vi "Position_TOTAL_R21_april_18.vi"(5 "Distance Between \nCameras  (*unit)":sgl=2.5) -> (12 "dX, dY\nLeft Cam":cluster{"X":sgl[], "Y":sgl[]}={"X"=[-5.750775, -4.1849813, -3.081379, -2.0098581, 0.0], "Y"=[7.9585915, 7.9595685, 7.960258, 7.960927, 0.0]}, 13 "Position Valid":bool=TRUE, 14 "Left Camera Real Coordinates":cluster{"X":sgl, "Y":sgl}={"X"=7.9602513, "Y"=5.592073}, 16 "dX, dY\nRight Cam":cluster{"X":sgl[], "Y":sgl[]}={"X"=[-7.3032045, -5.737411, -4.6338086, -3.5622878, -1.5524296], "Y"=[7.2714148, 7.2723923, 7.2730813, 7.273751, -0.68717635]}, 18 "Robot Coordinates":cluster{"X":sgl, "Y":sgl}={"X"=7.616663, "Y"=6.3682876}, 19 "Orietnation\n(current)":sgl=-23.843685 format="%#_13g")   [LabVIEW 2015]
uses:
  <vilib>/Analysis/NI_AALPro.lvlib
  <vilib>/myRIO/Instrument Drivers/Onboard IO/DIO/DIO.lvlib
  <vilib>/Analysis/coordinate.llb/2D Cartesian Coordinate Rotation (Array).vi
  <vilib>/Instr/_visa.llb/VISA Configure Serial Port (Instr).vi
panel:
  out "Current Cam State - L":T1(ring)
  out "Valid Beacon Sets_":bool[](array[boolean])=[TRUE, TRUE, TRUE, TRUE, FALSE]
  in  "Distance Threshold\nRef Triangles (*unit)":sgl=30.0
  out "dA2 4":sgl=9.6935425 format="%#_13g"
  out "dA2 2":sgl=9.6935425 format="%#_13g"
  out "dA2 3":sgl=9.6935425 format="%#_13g"
  out "Current Cam State - R":T1(ring)
  out "Beacon Scales - Left":sgl[](array[numeric])=[76.306, 116.841255, 157.35043, 195.67218, 0.0]
  out "Beacon Scales - Right":sgl[](array[numeric])=[76.306, 116.841255, 157.35043, 195.67218, 0.0]
  in  "New Orientation \nThreshold":sgl=10.0
  in  "Moving Average\nWindow Length":u8=5
  out "Current Recovery State -L":enum16{"Generic Sweep", "Recovery Search"}(ring)=enum."Recovery Search"
  out "Current Move Delta - L 2":u16
  out "Next Recovery State - Left":enum16{"Generic Sweep", "Recovery Search"}(ring)=enum."Recovery Search"
  out "Next Recovery State - Right":enum16{"Generic Sweep", "Recovery Search"}(ring)=enum."Recovery Search"
  out "Current Recovery State - Right":enum16{"Generic Sweep", "Recovery Search"}(ring)=enum."Recovery Search"
  in  "Initial Recovery State  - Right":enum16{"Generic Sweep", "Recovery Search"}(ring)=enum."Recovery Search"
  in  "Initial Recovery State - L":enum16{"Generic Sweep", "Recovery Search"}(ring)=enum."Recovery Search"
  out "Next Tracking State - Right":enum16{"Track", "Reactive Predict", ""}(ring)
  out "Current Tracking State - Right 2":enum16{"Track", "Reactive Predict", ""}(ring)
  in  "Initial Tracking State - Right":enum16{"Track", "Reactive Predict", ""}(ring)
  out "Last Track Angle - R":sgl=98.61328
  out "Next Tracking State - Left":enum16{"Track", "Reactive Predict", ""}(ring)
  in  "Initial Tracking State - Left":enum16{"Track", "Reactive Predict", ""}(ring)
  out "Current Tracking State - Left":enum16{"Track", "Reactive Predict", ""}(ring)
  in  "Timeout to \nEnable Reactive Predict":u16=5
  out "Tracking Timeout\nCount - R":i32
  in  "Tracking Timeout\nThreshold":i32=10
  out "Tracking Timeout\nCount - L":i32
  in  "Search Direction - in - Right":bool=TRUE
  out "Next Main State - Right":T2(ring)=enum."Tracking"
  in  "Recovery Search\nDirection - R":bool
  out "Recovery Mode Count in Right":i32
  out "Frames Processed\nCount - in Right":i32
  out "Recovery Search\nmove Count - Right":u16
  out "Recovery Search\nAttempt Count - Right":u16
  in  "Mounting Offset - Right":sgl=45.0
  in  "Tracking Angle - Right":sgl=98.60307
  in  "Current Servo Position\n- Right":u16
  out "New Data  Flag\nRight Servo":bool
  in  "Track Angle Valid  - Right":bool=TRUE
  out "Current Main State - Right":T2(ring)=enum."Tracking"
  in  "Initial Main State- Right":T2(ring)
  in  "Recovery Search\nDirection - L 2":bool
  in  "Max Recovery Count\n(Recovery Search) 2":u16
  in  "Max Recovery\nSearch Attempts 2":u16
  in  "Image Lock - Right 2":bool
  out "Last Track Angle - L":sgl=87.24609
  in  "Recovery Search\nDirection - L":bool=TRUE
  out "Next Main State - Left":T2(ring)=enum."Tracking"
  out "Current Move Delta - L":u16
  in  "Max Recovery Count\n(Recovery Search)":u16=10
  in  "Max Recovery\nSearch Attempts":u16=3
  out "Recovery Search\nAttempt Count - in - L":u16
  out "Recovery Search\nmove Count - in - L":u16
  in  "Image Lock - Right":bool=TRUE
  out "Recovery Mode Count - in Left":u16
  in  "Middle Beacon\nCoordinates":cluster{"X":sgl, "Y":sgl}={"X"=0.0, "Y"=2.5}
  in  "Min Num Frames\nper Search":i32=2
  in  "Wait Tick Threshold":i32=10
  out "Frames Processed\nCount - in -L":i32
  in  "Maximum Move \nServo Threshold":i16=300
  in  "Minimum Delta \nServo Threshold":i16=3
  in  "Mounting Offset - Left":sgl=-45.0
  in  "Search Step Size":u16=50
  in  "Search Direction - in - L":bool
  in  "Current Servo Position\n- Left":u16
  in  "Tracking Angle - Left":sgl=87.25689
  out "New Data  Flag\nLeft Servo":bool
  in  "Track Angle Valid - Left":bool=TRUE
  in  "Image Lock - Left":bool=TRUE
  in  "Initial Main State - Left":T2(ring)
  out "Current Main State - Left":T2(ring)=enum."Tracking"
  in  "Position Calc\nTimer":u32=100 caption="Position Calc Timer"
  in  "Fetch Input\n(mSec)":u32=20 caption="Update Camera Input\n(mSec)"
  out "Right Data\nInput Flag\n- Internal":bool=TRUE
  in  "Position Calc\nReady":bool
  out "This Servo \nAngle - Right":sgl=98.90625
  in  "Beacon Angles -R":sgl[](array[numeric])=[111.28093, 105.355774, 98.60307, 92.04714, 103.90625]
  in  "Beacon Angles - L":sgl[](array[numeric])=[101.98467, 94.59042, 87.25689, 80.30646, 91.66016]
  in  "Valid Angles -R":bool[](array[boolean])=[TRUE, TRUE, TRUE, TRUE, FALSE]
  in  "Valid Angles - L":bool[](array[boolean])=[TRUE, TRUE, TRUE, TRUE, FALSE]
  out "Left Data\nInput Flag\n- Internal":bool
  in  "Check Shared Var Timer":u32=50 caption="Main Loop\n Timer (ms)"
  out "Left_Flag 2":bool
  out "Right_Flag 2":bool
  out "Beacons Found\n- Left (Bool Array) 2":bool[](array[boolean])=[TRUE, TRUE, TRUE, TRUE, FALSE]
  out "LEFT Beacon Coord - X px (IN) 2":sgl[](array[numeric])=[76.306, 116.841255, 157.35043, 195.67218, 0.0]
  out "LEFT Beacon Position - Y px (IN) 2":sgl[](array[numeric])=[154.30304, 148.59094, 148.39949, 146.94655, 0.0]
  out "This Servo \nAngle - Left":sgl=86.66016
  in  "Compliance Slope":u8=128
  out "deltaMoveServo\n- R":i16
  out "Move Respond - R":bool
  out "Move Respond - L":bool
  out "Last Position":cluster{"X":sgl, "Y":sgl}={"X"=7.6261, "Y"=6.350474}
  out "Last Orientation":sgl=-23.876373
  in  "Distance\nBetween Beacons \n- Tolerance":sgl=0.35 format="%#_13g"
  in  "Distance\nBetween Beacons":sgl=1.0 format="%#_13g"
  out "dT":dbl=143.499
  out "Position Valid\nHistory":bool[](array[boolean])=[TRUE, FALSE, FALSE, TRUE, TRUE, FALSE, TRUE, TRUE, TRUE, TRUE, TRUE, TRUE, FALSE, TRUE, FALSE]
  out "Orientation\nHistory":sgl[](array[numeric])=[-23.876373, 0.0, 0.0, -23.938759, -24.0458, 0.0, -23.14014, -22.504314, -22.596928, -22.90728, -23.237453, -23.75214, 0.0, -23.808718, 0.0]
  out "Robot Coordinates\nHistory":cluster{sgl, sgl}[](array[cluster])=[{7.6261, 6.350474}, {0.0, 0.0}, {0.0, 0.0}, {7.63815, 6.33973}, {7.6316156, 6.322055}, {0.0, 0.0}, {7.6863523, 6.2558875}, {7.688662, 6.2228284}, {7.6736236, 6.2455945}, {7.6880507, 6.2819676}, {7.6893277, 6.3140097}, {7.668109, 6.3330927}, {0.0, 0.0}, {7.6506357, 6.3142757}, {0.0, 0.0}]
  in  "New Position \nThreshold":sgl=2.5
  out "Orientation Avgd":sgl=-23.876373
  in  "History Size":u8=15
  in  "Max Y (arena)":sgl=15.0
  in  "Max X (arena)":sgl=35.0
  in  "New Position\nWeight":sgl=0.5 format="%#_13g"
  in  "Max Std Dev (3)":sgl=0.2 format="%#_13g"
  in  "Max Std Dev (4)":sgl=0.2 format="%#_13g"
  out "Post Filtering\n- Valid Beacons":bool[](array[boolean])=[FALSE, TRUE, TRUE, TRUE, FALSE]
  out "Robot Coordinates - Avgd":cluster{"X":sgl, "Y":sgl}={"X"=7.6261, "Y"=6.350474}
  out "Real Position in Course 2":cluster{"X":dbl[], "Y":dbl[]}(graph)={"X"=[7.626100046018056], "Y"=[6.35047366782369]}
  out "Position \nLock Status":bool=TRUE
  out "Right Camera Real Coordinate":cluster{"X":sgl, "Y":sgl}={"X"=7.2730746, "Y"=7.1445026}
  out "deltaMoveServo\n- L":i16
  in  "Search Step Size\n(deg)":sgl=15.0 format="%#_13g"
  out "Beacons Found\n- Right (Bool Array)":bool[](array[boolean])=[TRUE, TRUE, TRUE, TRUE, FALSE]
  out "RIGHT Beacon Position - Y px (IN)":sgl[](array[numeric])=[153.02994, 149.48933, 150.4864, 150.33003, 0.0]
  out "RIGHT Beacon Coord - X px (IN)":sgl[](array[numeric])=[91.3685, 123.99656, 161.27843, 197.4523, 0.0]
  in  "Right Servo\nID":string="\u0001"
  in  "Servo Comm\nWait Time - (ms)":i32
  in  "Left Servo\nID":string="\u0000"
  out "dT - Comm Loop":u32=19
  in  "Servo Comm\nLoop Time (ms)":i32=20
  in  "close comms":bool
  in  "Max Read\nTx Attempts":u8=3
  in  "Max Write\nTx Attempts":u8=3
  out "Current R (10bit)":u16=696
  out "Servo Moving - R":bool
  out "Servo Moving - L":bool
  out "Current L (10bit)":u16=347
  in  "SERVO ENABLE":bool=TRUE
  out "Move Servo - L":bool
  out "Move Servo - R":bool
  in  "Servo Goal Position\n - Right":u16=695
  in  "Move Servo\nThreshold (deg)":sgl=2.0 format="%#_13g"
  in  "Servo Algorithm\nCycle Time(ms)":i32=25
  in  "Servo Goal Position\n - Left":u16=349
  in  "Current Angle\n - Left (internal)":sgl=86.66016
  in  "Current Angle\n - Right (internal)":sgl=98.90625
  in  "stop":bool
  in  "Num of Beacons (Total)":i8=5
  out "Angle to Pixel Ratios":T3={"Angle to Pixel\nRatio - Horizontal"=0.18125, "Angle to Pixel\nRatio - Vertical"=0.1875} {"Angle to Pixel\nRatio - Vertical" format="%#_13g"; "Angle to Pixel\nRatio - Horizontal" format="%#_13g"}
  in  "Cam AOV Vertical (deg)":sgl=45.0
  in  "Cam AOV Horizontal (deg)":sgl=58.0
  in  "Image Height (px)":sgl=240.0
  in  "Image Width (px)":sgl=320.0
  out "Beacon Coordinates - Left Image":T4={"Beacon Position - X px"=[76.306, 116.841255, 157.35043, 195.67218, 0.0], "Beacon Position - Y px"=[154.30304, 148.59094, 148.39949, 146.94655, 0.0]}
  out "Beacon Coordinates - Right Image":T4={"Beacon Position - X px"=[91.3685, 123.99656, 161.27843, 197.4523, 0.0], "Beacon Position - Y px"=[153.02994, 149.48933, 150.4864, 150.33003, 0.0]}
  out "Distance to LBF":sgl[](array[numeric])=[0.024284193, 0.015691843, 0.008273765, 0.028971607, 0.03291407]
  out "Local Coordinates - Calculated":cluster{sgl[], sgl[]}(graph)={[-2.0384164, -0.70265853, 0.4090246, 1.3811935, 0.0], [9.602626, 8.751521, 8.536832, 8.085801, 0.0]}
  out "Local Coordinates - Rotated":cluster{dbl[], dbl[]}(graph)={[1.5524295802029098, -5.750774735805926, -4.1849814062260675, -3.0813788557258652, -2.009858210562305, 0.0], [0.6871763361707266, 7.9585912385832795, 7.959568450875426, 7.960257859242679, 7.960927027680405, 0.0]}
  out "All Object Coordinates \n- Local - Rotated":cluster{"X":sgl[], "Y":sgl[]}={"X"=[1.5524296, -5.750775, -4.1849813, -3.081379, -2.0098581, 0.0], "Y"=[0.68717635, 7.9585915, 7.9595685, 7.960258, 7.960927, 0.0]}
  out "Local Coordinates - Normalized":cluster{sgl[], dbl[]}(graph)={[1.6977187, -2.0372734, -0.60508364, 0.4043527, 1.3844445, 0.0], [0.0, 9.605212211608887, 8.972328186035156, 8.526259422302246, 8.093157768249512, 0.0]}
  in  "Max Std Dev (5)":sgl=0.2 format="%#_13g"
  out "All Object Coordinates \n- Local":cluster{"X":sgl[], "Y":sgl[]}={"X"=[1.6977187, -2.0372734, -0.60508364, 0.4043527, 1.3844445, 0.0], "Y"=[0.0, 9.605212, 8.972328, 8.526259, 8.093158, 0.0]}
  out "LOCAL\nBeacon Coordinates\nRelative to Robot":cluster{"dX_beacon":sgl[], "dY_beacon":sgl[]}={"dX_beacon"=[-2.0384164, -0.70265853, 0.4090246, 1.3811935, 0.0], "dY_beacon"=[9.602626, 8.751521, 8.536832, 8.085801, 0.0]}
  in  "Real Beacon\n - Coordinates":cluster{"X":dbl[], "Y":dbl[]}={"X"=[0.0, 0.0, 0.0, 0.0, 0.0, 0.0], "Y"=[0.5, 1.5, 2.5, 3.5, 4.5, 0.0]}
  # "POSITION CALCULATION VARIABLES"
  # "OUTPUT VALUES"
  # "CONFIG VALUES"
  # "FILTER CONFIG VALUES"
  # "FEEDBACK INPUT VALUES"
  # "INPUT VALUES"
  # "INTERMEDIATE VALUES"
  # "IMAGE TO ANGLE VARIABLES"
  # "VISION PROCESSEING INPUTS"
  # "Use moving average for previous orientation thresholds"
  # "INPUTS"
  # "CONFIG"
  # "OUTPUT VALUES"
  # "*********************"
  # "unfiltered"
  # "NEW FILTER VALS"
  # "Inter Beacon Distance Filtering"
  # "SERVO CONTROL VARIABLES"
  # "SERVO CONTROL VARIABLES"
  # "CONFIG"
  # "SHARED VARIABLE INPUTS"
  # "LOCAL VARIABLE INPUTS"
  # "INTERNRAL VARIABLES"
  # "SEARCH ROUTINE VARIABLES"
  # "MISC"
  # "SERVO IDs"
  # "CONTROL DELAYS"
  # "COMM LOOP DELAY"
  # "COMM PROTOCOL"
  # "SETTINGS"
  # "Make function of distance^^"
  # "**** only left side starts search\nat previously known good angle"
  # "LEFT SERVO"
  # "RIGHT SERVO"
  # "Main State Machine"
  # "Recovery State Machine"
  # "Current Track Angle Inputs"
  # "Servo Status Inputs"
  # "Main State Machine Inputs"
  # "Recovery State Machine Inputs"
  # "Current Track Angle Inputs"
  # "Servo Status Inputs"
  # "Recovery State Machine Feedback"
  # "Tracking State Machine Inputs"
  # "Tracking State Machine Inputs"
  # "NOTE: Must be 1 bigger than amount of beacons"
  # "NOTE: Must be 1 bigger than amount of beacons"
types:
  T1 = enum16{"Super Close Range", "Short Range", "Long Range"}
  T2 = enum16{"Start Up Search", "Tracking", "Recovery Mode", ""}
  T3 = cluster{"Angle to Pixel\nRatio - Horizontal":sgl, "Angle to Pixel\nRatio - Vertical":sgl}
  T4 = cluster{"Beacon Position - X px":sgl[], "Beacon Position - Y px":sgl[]}
  T5 = cluster{"Tracking Coordinates":cluster{"X":dbl, "Y":dbl}, "Current Valid":bool, "Current State - Out":enum16{"Sub - 2", "Sub - 3", "Sub - 4", "Normal - 5"}}
  T6 = enum16{"Sub - 2", "Sub - 3", "Sub - 4", "Normal - 5"}
  T7 = cluster{"Array of Double":dbl[], "Array of Double":dbl[]}
  T8 = typedef "DIO.lvlib/DIO Reference.ctl" = cluster{"myRIO Reference":T9, "DIO Channels List":T13}
  T9 = typedef "myRIO Generic Hardware Reference.ctl" = cluster{"myRIO Model":T10, "myRIO Hardware Reference":T11}
  T10 = typedef "Hardware Version Enum.ctl" = enum16{"Unknown", "myRIO-1900", "myRIO-1950", "roboRIO"}
  T11 = typedef "myRIO v1.0 Reference.ctl" = cluster{"Generic FPGA Reference":T12, "Allow multiple opens":bool}
  T12 = typedef "Generic FPGA Reference.ctl" = refnum<k20>
  T13 = typedef "DIO Channels List.ctl" = T14[]
  T14 = typedef "DIO Channels Enum.ctl" = enum16{"Not Connected", "C/DIO0", "C/DIO1", "C/DIO2", "C/DIO3", "C/DIO4", "C/DIO5", "C/DIO6", "C/DIO7", "A/DIO0", "A/DIO1", "A/DIO2", "A/DIO3", "A/DIO4", "A/DIO5", "A/DIO6", "A/DIO7", "A/DIO8", "A/DIO9", "A/DIO10", "A/DIO11", "A/DIO12", "A/DIO13", "A/DIO14", "A/DIO15", "B/DIO0", "B/DIO1", "B/DIO2", "B/DIO3", "B/DIO4", "B/DIO5", "B/DIO6", "B/DIO7", "B/DIO8", "B/DIO9", "B/DIO10", "B/DIO11", "B/DIO12", "B/DIO13", "B/DIO14", "B/DIO15", "LED0", "LED1", "LED2", "LED3", "Button0", "DIO/DIO0", "DIO/DIO1", "DIO/DIO2", "DIO/DIO3", "DIO/DIO4", "DIO/DIO5", "DIO/DIO6", "DIO/DIO7", "DIO/DIO8", "DIO/DIO9", "SPI/CS0", "SPI/CS1", "SPI/CS2", "SPI/CS3", "LED RADIO (Green)", "LED RADIO (Red)", "LED COMM (Green)", "LED COMM (Red)", "LED MODE (Green)", "LED MODE (Red)"}
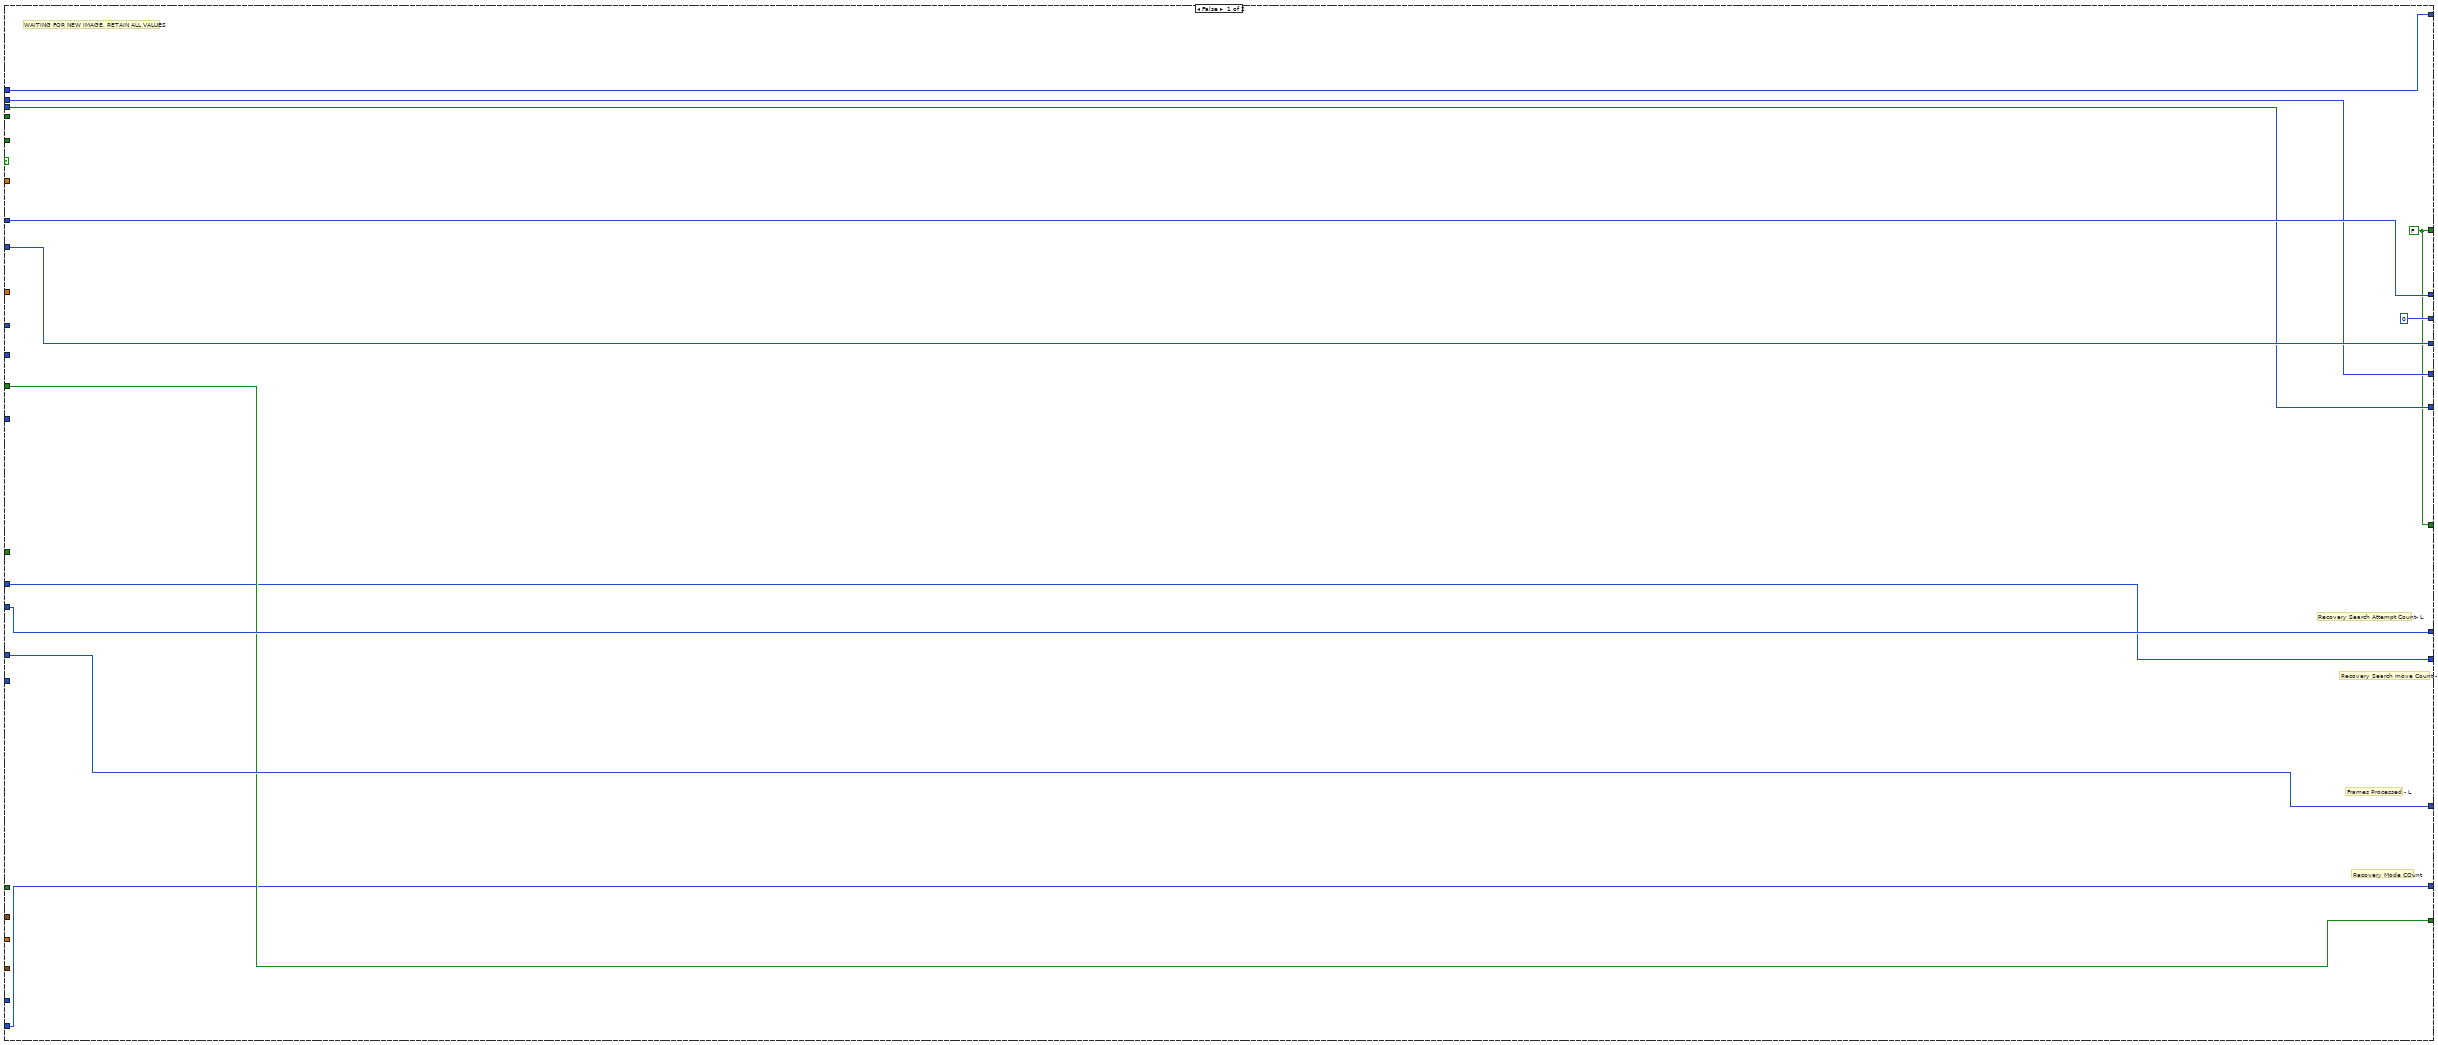
[diagram p2: hidden frame]
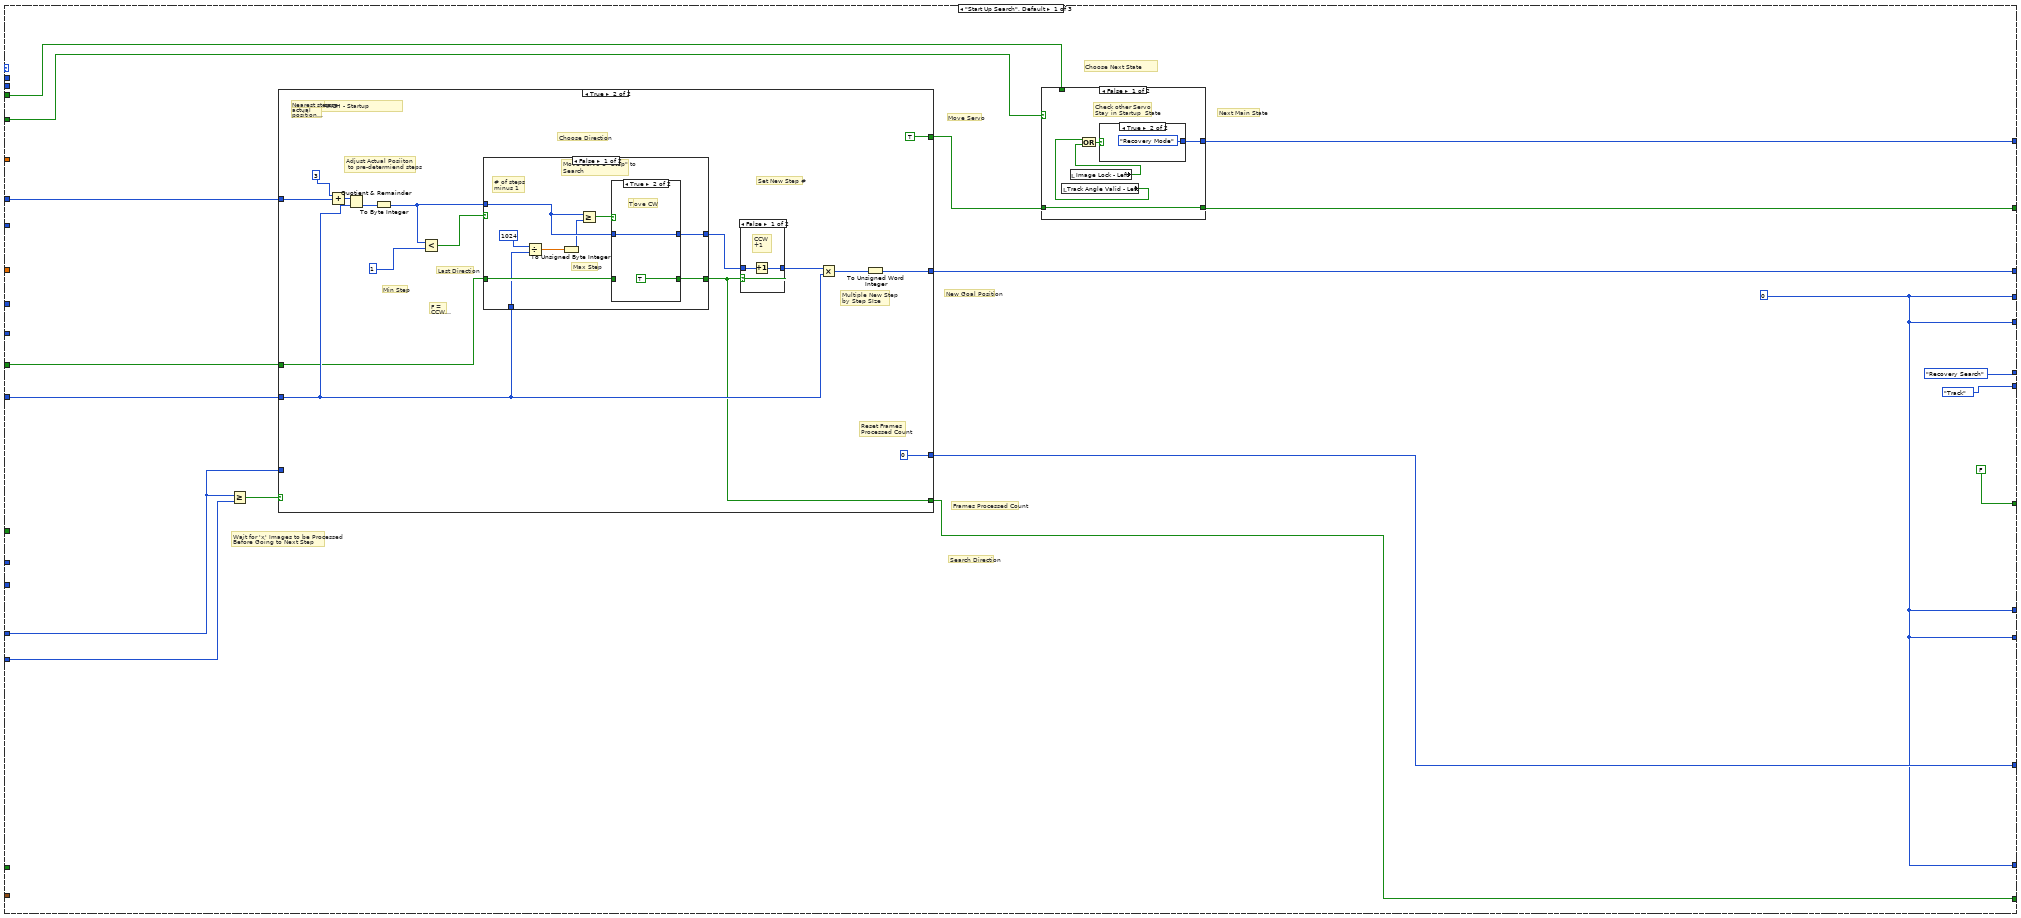
[diagram p3: hidden frame]
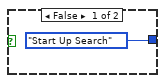
[diagram p4: hidden frame]
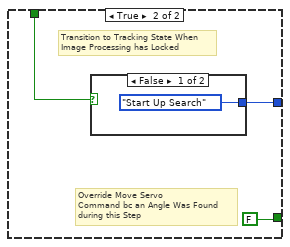
[diagram p5: hidden frame]
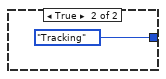
[diagram p6: hidden frame]
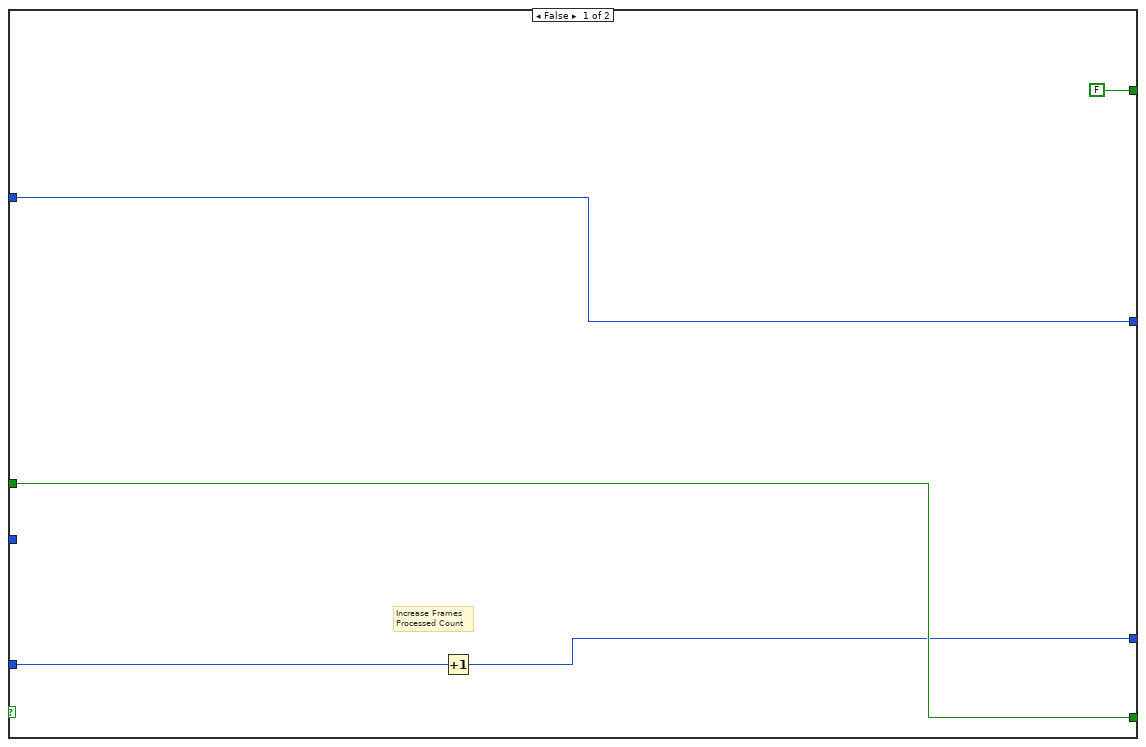
[diagram p7: hidden frame]
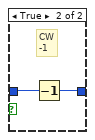
[diagram p8: hidden frame]
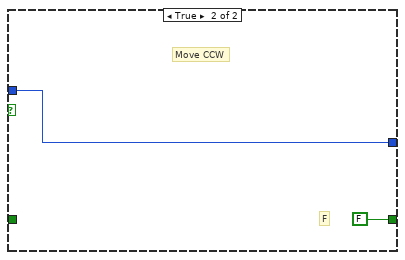
[diagram p10: hidden frame]
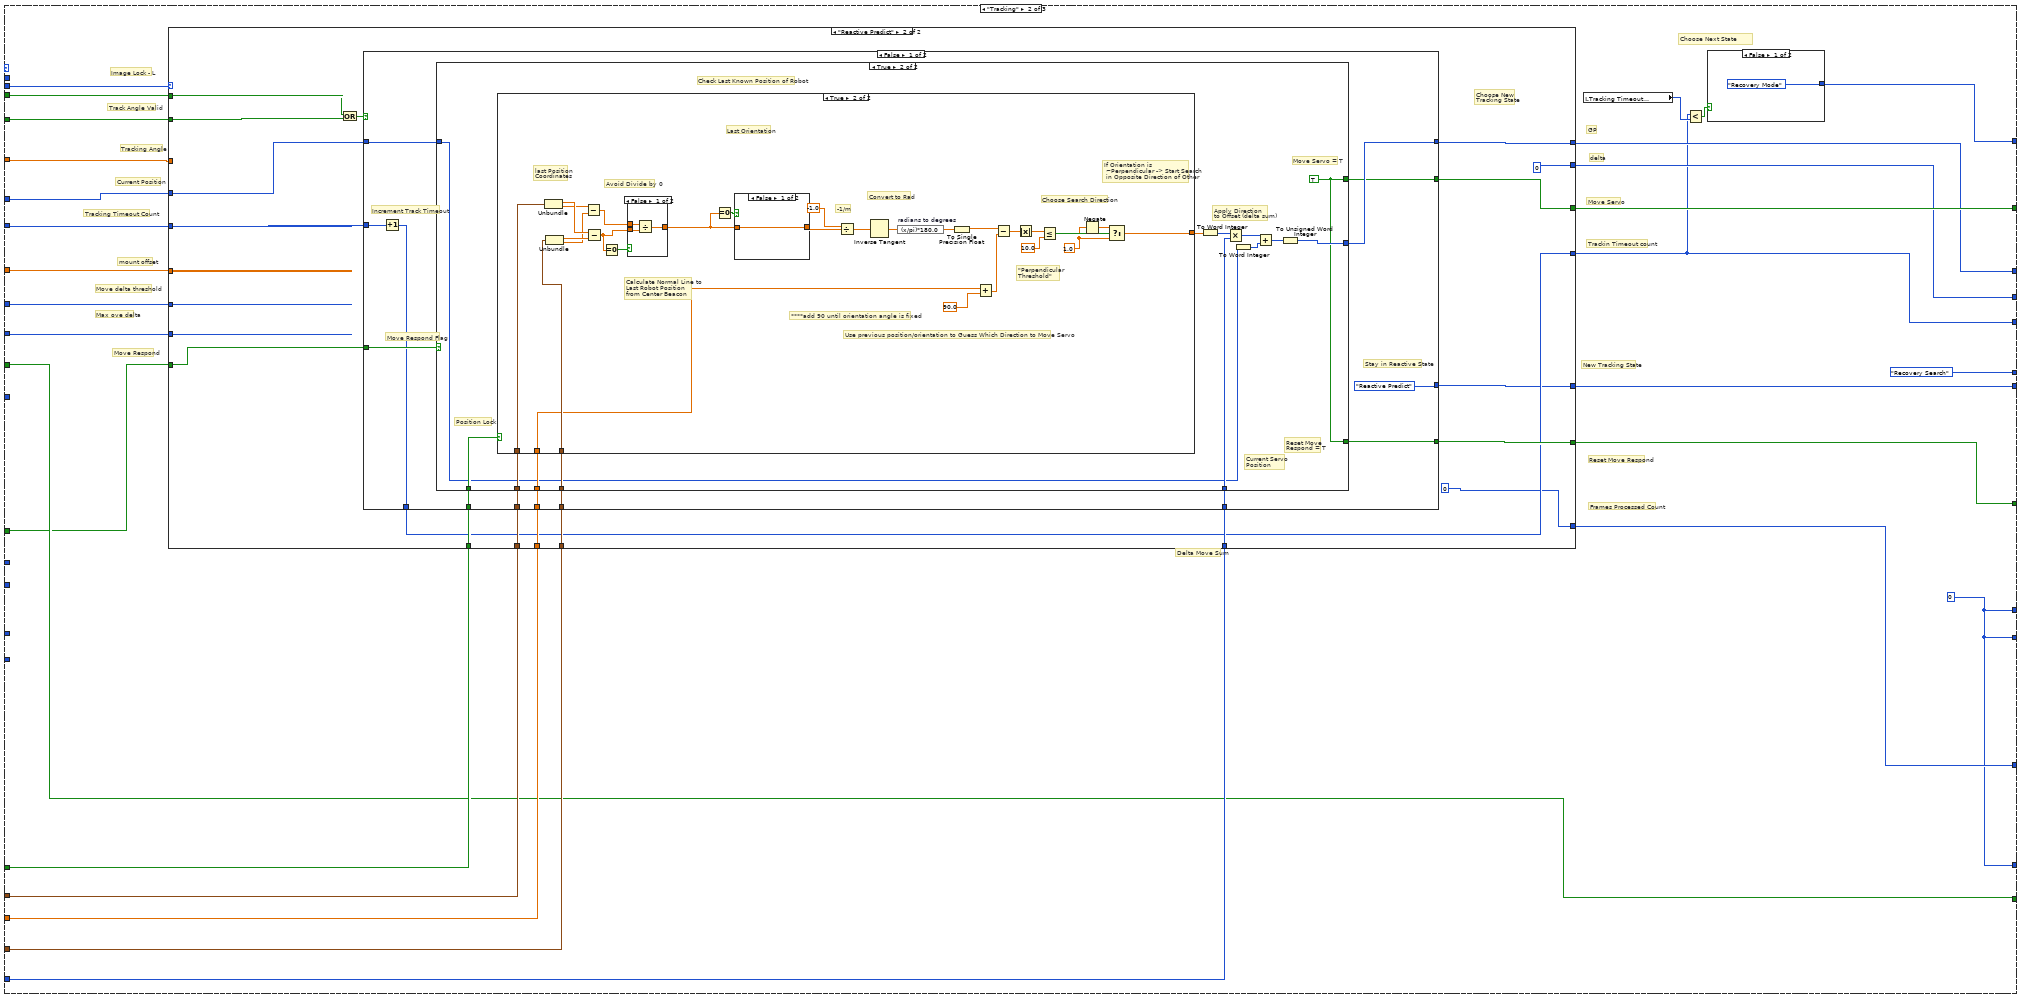
[diagram p11: hidden frame]
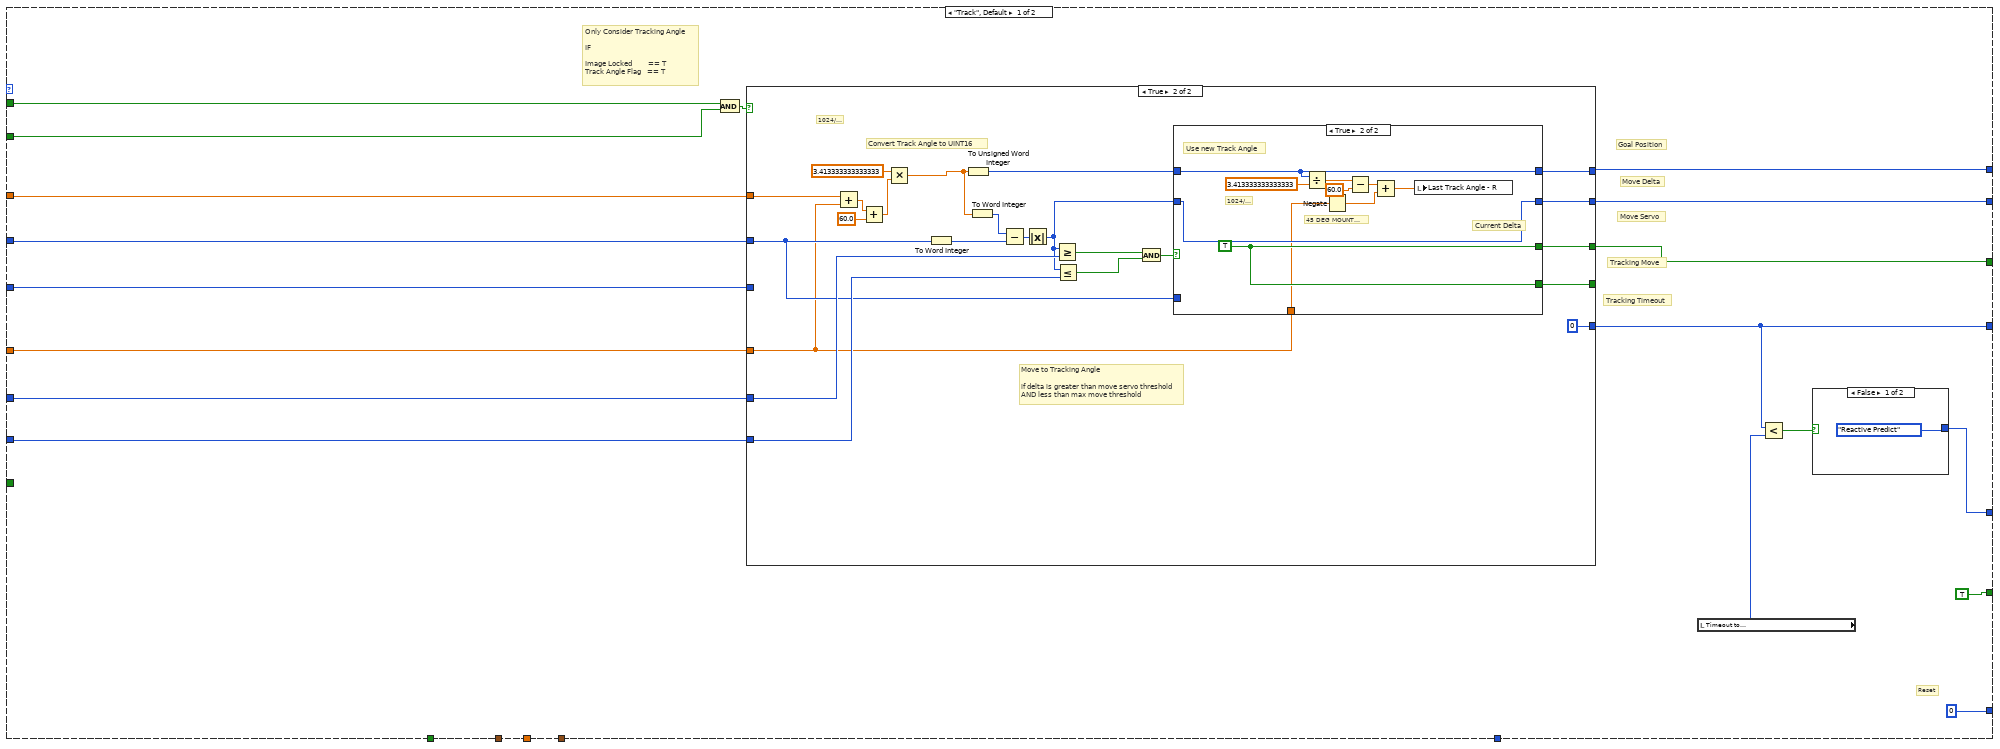
[diagram p12: hidden frame]
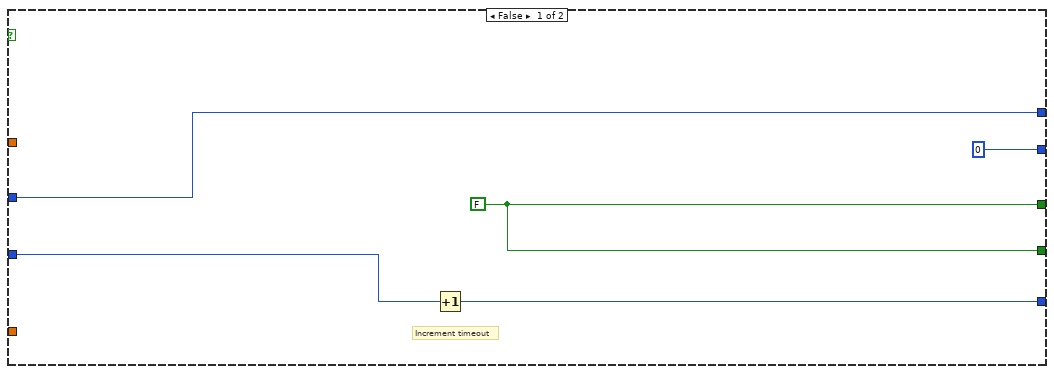
[diagram p13: hidden frame]
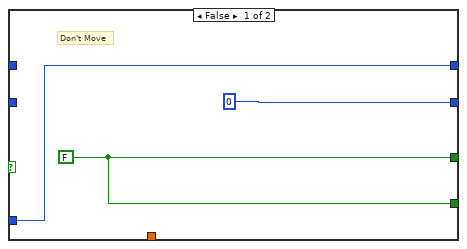
[diagram p14: hidden frame]
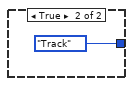
[diagram p15: hidden frame]
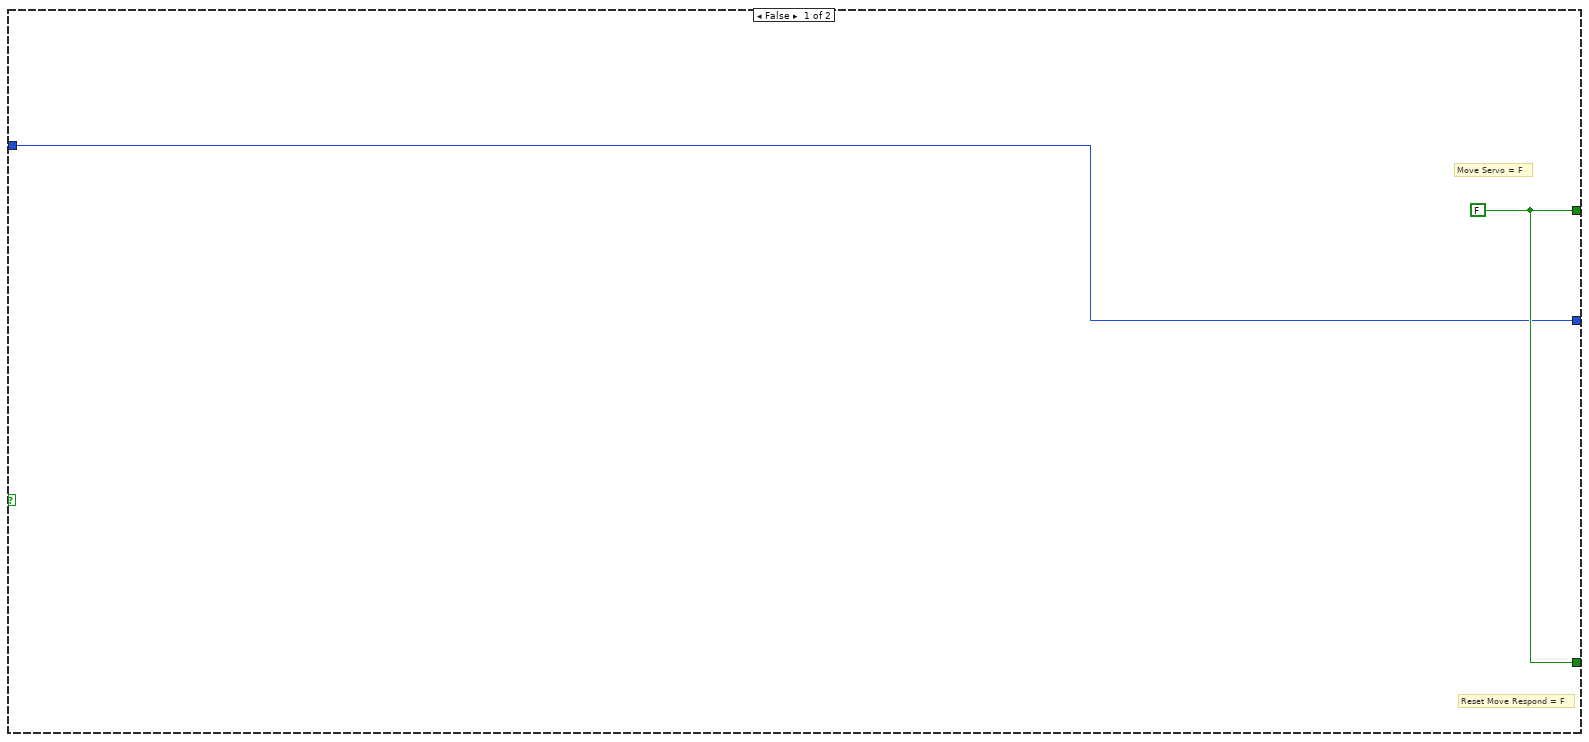
[diagram p16: hidden frame]
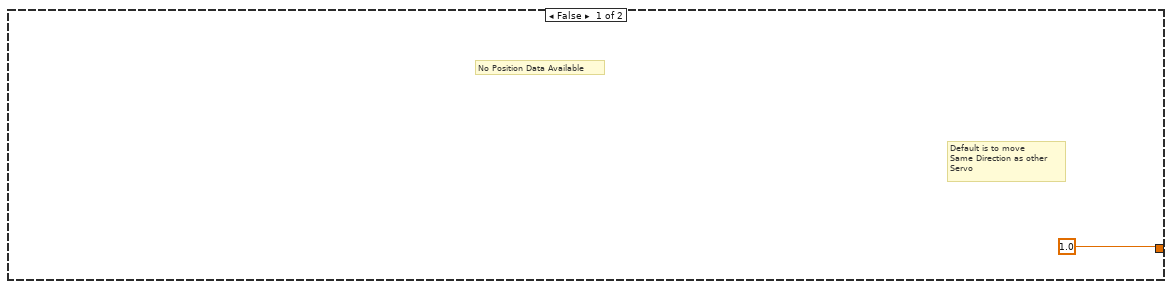
[diagram p17: hidden frame]
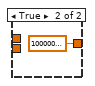
[diagram p18: hidden frame]
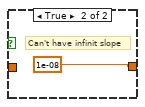
[diagram p19: hidden frame]
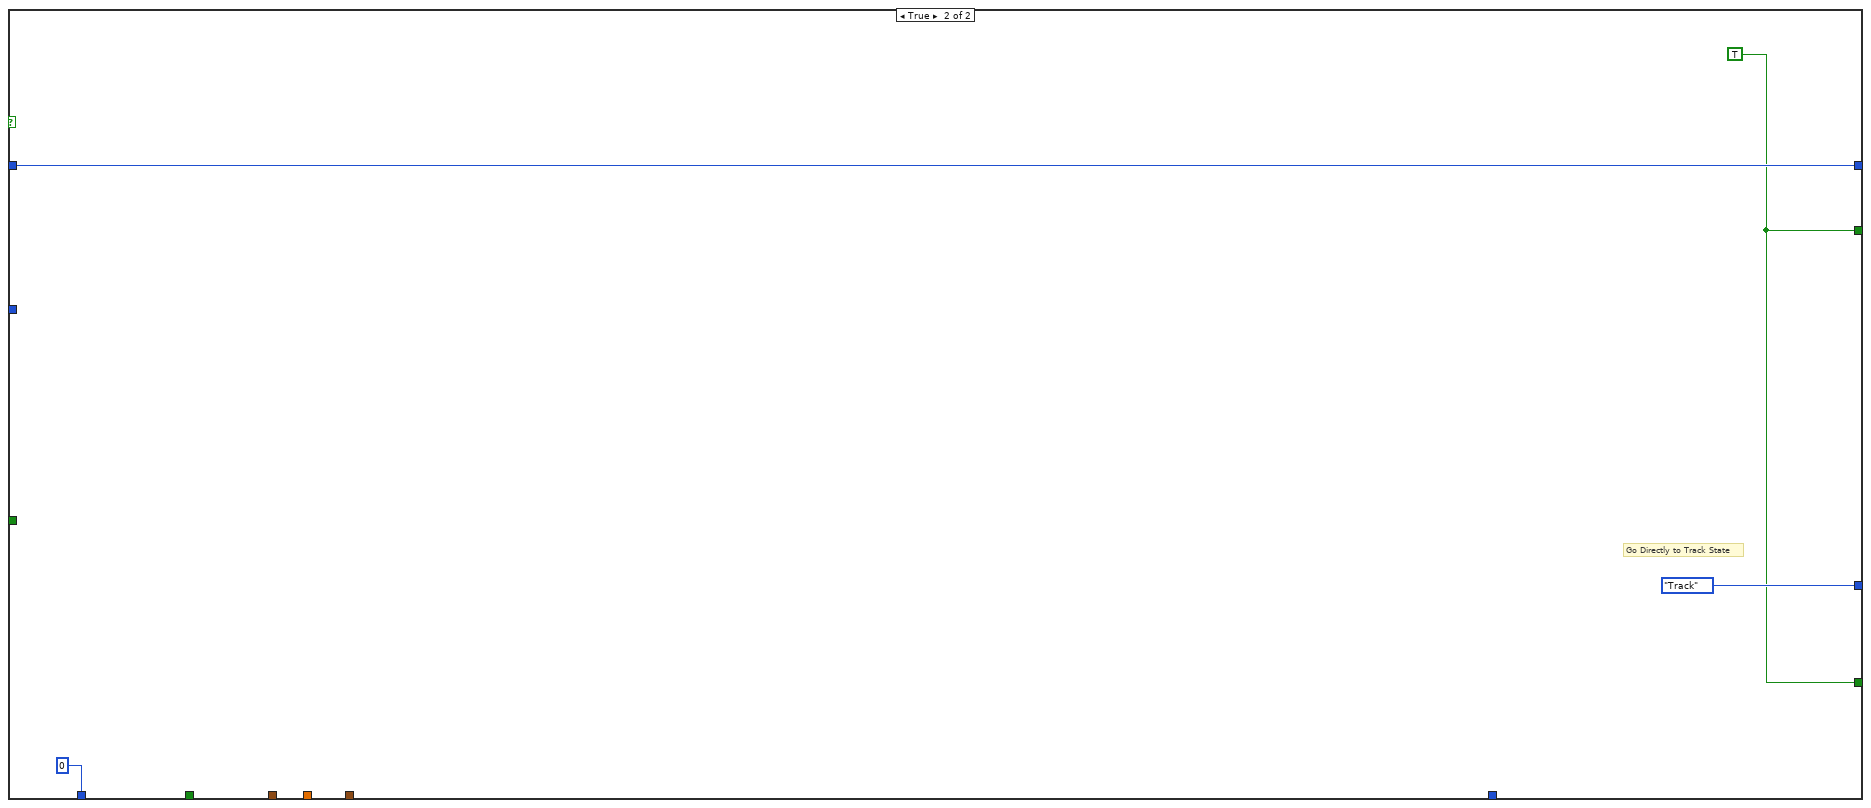
[diagram p20: hidden frame]
diagram:
  (unwired) enum16{"Generic Sweep", "Recovery Search"}."Recovery Search"
  w12 = 0 ("Frames Processed\nCount - in")
  w13 = 0 ("Frames Processed\nCount - in")
  w2 = FALSE
  w34 = sgl 0.0
  # "SERVO CONTROL FLAGS"
  # "***"
  # "Next Tracking State"
  # "Tracking Timeout Count"
  # "Search Direction - L"
  # "Next Recovery State"
  # "Move Respond"
  # "Recovery Mode Count - L"
  # "Delta Move Sum - L"
  # "Wait Tick Count - L"
  # "Frames Processed - L"
  # "Recovery Search move Count - L"
  # "Recovery Search Attempt Count- L"
  # "Next Main State"
  # "Search Direction - L"
  # "Next Recovery State"
  # "INPUTS - Local vars"
  # "Recovery Mode Count - L"
  # "Delta Move Sum - L"
  # "Frames Processed\nLeft"
  # "Move Respond - R"
  # "Initial Search Direction\n- Right"
  # "Move Respond"
  # "Recovery Mode Count - L"
  # "Delta Move Sum - L"
  # "Wait Tick Count - L"
  # "Frames Processed - L"
  # "Recovery Search move Count - L"
  # "Recovery Search Attempt Count- L"
  # "Next Main State"
  # "Settings -- Update in a slow loop"
  # "Recovery Mode Count - L"
  # "Delta Move Sum - L"
  # "Frames Processed\nLeft"
  # "Move Respond - L"
  # "Replace these with\nconstants"
  # "Initial Search Direction\n- Left"
  # "Read Inputs when Available"
  # "# of Physical Beacons"
  # "Right Data Internal Falg"
  # "Left Data Internal Falg"
  # "Initialize Shift Arrays"
  # "Robot Position (cluster)\nShift Array"
  # "Robot Position (cluster)\nShift Array"
  # "Position Valid Shift Array"
  # "Orientation Shift Array"
  # "Position Valid Shift Array"
  # "Orientation Shift Array"
  # "Servo Communication (to Servo- UART))"
  # "Internal Local Variables"
  # "Servo Control Logic"
  # "Local Variables"
  # "Images to Robot Position Calculation Process"
  # "SERVO MOTOR CONTROL"
  # "SERVO MOTOR CONTROL"
  n1 = Divide(x="Cam AOV Horizontal (deg)", y="Image Width (px)") -> (x/y=w25:sgl)
  n2 = Divide(x="Cam AOV Vertical (deg)", y="Image Height (px)") -> (x/y=w26:sgl)
  n3 = Bundle(w25, w26) -> (w20:cluster{sgl, sgl})  [unwired: 1 in]
  "Angle to Pixel Ratios" <- w20
  n4 = disable-structure shown="Disabled" {
    frame Disabled {
      # "Always Read Incoming Flags & Store"
      n5 = while {
        tunnel: "Check Shared Var Timer" -> [w46]
        stop <- FALSE stop-if-true
        n6 = shared-variable "myRIO-1900\\Lib1.lvlib\\RIGHT_FLAG"() -> (→"Right_Flag 2":bool)  [unwired: 1 in, 1 out]
        n7 = shared-variable "myRIO-1900\\Lib1.lvlib\\Left_Flag"() -> (→"Left_Flag 2":bool)  [unwired: 1 in, 1 out]
        n8 = call "Wait8"("Count(mSec)"=w46) -> ()  [unwired: 1 out]
      }
    }
    frame Enabled {
    }
  }
  n9 = while {
    shift-right: [w55] -> _
    shift-left: w2 -> [w60]
    shift-right: [w54] -> _
    shift-left: w2 -> [w58]
    tunnel: w20 -> [w56]
    tunnel: "Num of Beacons (Total)" -> [w57]
    stop <- FALSE stop-if-true
    # "Wait for Both Internal Flags"
    n10 = call "Wait6"("Count(mSec)"="Fetch Input\n(mSec)") -> ()  [unwired: 1 out]
    n11 = shared-variable "RT myRIO Target - Overlord\\Localization_Variables_r0.lvlib\\RIGHT_FLAG"() -> (w51:bool)  [unwired: 1 in, 1 out]
    n12 = shared-variable "RT myRIO Target - Overlord\\Localization_Variables_r0.lvlib\\Left_Flag"() -> (w52:bool)  [unwired: 1 in, 1 out]
    n13 = case shown="True" w51 {
      tunnel: w57 -> [_ w79]
      tunnel: w56 -> [_ w77]
      tunnel: [w61 w67] -> w49
      tunnel: w58 -> [w61 _]
      frame False {
        # "Don't Update Servo Position\nbc we're waiting on new Data to\ncome in and the servo position\nwas set at the previous set of data"
      }
      frame True {
        w67 = TRUE
        # "Store Values"
        # "Raise Internal Flag"
        # "If New Data Available"
        # "From Shift Reg"
        # "Perforrm Indivudual Angle Calculation"
        # "Pull Down Individual Flag"
        n14 = shared-variable "RT myRIO Target - Overlord\\Localization_Variables_r0.lvlib\\RIGHT_BEACON_X_array"() -> (w73:dbl[])  [unwired: 1 in, 1 out]
        "RIGHT Beacon Coord - X px (IN)" <- w73
        n15 = shared-variable "RT myRIO Target - Overlord\\Localization_Variables_r0.lvlib\\Image Lock - R"() -> (w68:bool)  [unwired: 1 in, 1 out]
        n16 = shared-variable "RT myRIO Target - Overlord\\Localization_Variables_r0.lvlib\\RIGHT_BEACON_Scales"() -> (→"Beacon Scales - Right":sgl[])  [unwired: 1 in, 1 out]
        n17 = shared-variable "RT myRIO Target - Overlord\\Localization_Variables_r0.lvlib\\Info - Right"() -> (w65:T5)  [unwired: 1 in, 1 out]
        n18 = shared-variable "RT myRIO Target - Overlord\\Localization_Variables_r0.lvlib\\RIGHT_BEACON_Y_array"() -> (w72:dbl[])  [unwired: 1 in, 1 out]
        "RIGHT Beacon Position - Y px (IN)" <- w72
        n19 = shared-variable "RT myRIO Target - Overlord\\Localization_Variables_r0.lvlib\\RIGHT_BEACON_BOOL_array"() -> (w71:bool[])  [unwired: 1 in, 1 out]
        "Beacons Found\n- Right (Bool Array)" <- w71
        n20 = Unbundle By Name(w65) -> ("Tracking Coordinates"=w64:cluster{"X":dbl, "Y":dbl}, "Current Valid"=w63:bool, "Current State - Out"=→"Current Cam State - R":T6)
        n21 = local write "Image Lock - Right"(w68) -> ()
        n22 = Bundle("Array of Double"=w73, "Array of Double"=w72) -> (w70:T7)  [unwired: 1 in]
        "Beacon Coordinates - Right Image" <- w70
        n23 = shared-variable "RT myRIO Target - Overlord\\Localization_Variables_r0.lvlib\\Right Servo Angle_Image"() -> (w69:dbl)  [unwired: 1 in, 1 out]
        "This Servo \nAngle - Right" <- w69
        n24 = shared-variable "RT myRIO Target - Overlord\\Localization_Variables_r0.lvlib\\RIGHT_FLAG"(FALSE) -> ()  [unwired: 1 in, 1 out]
        n25 = feedback #1() -> (w81:sgl[])  [unwired: 1 in]
        n26 = feedback #2() -> (w80:bool[])  [unwired: 1 in]
        n27 = call "Angle Calc_Individual Process R4.vi"("Angle to Pixel Ratios"=w77, "Previous Angles"=w81, "Num of Beacons"=w79, "Beacon Coordinates - Image"=w70, "Current Servo Angle"=w69, "Beacons Found (Bool Array)"=w71, "Previous Valid Angles"=w80, "Tracking Coordinates"=w64) -> ("Servo Goal Angle"=w76:sgl, "Valid Beacons (Bool Array)\nPosition Calc"=w75:bool[], "Angle Of Beacons \nRelative to Robot"=w74:sgl[])  [unwired: 4 in, 1 out]
        n28 = feedback-in #1(w74) -> ()
        n29 = feedback-in #2(w75) -> ()
        n30 = local write "Beacon Angles -R"(w74) -> ()
        n31 = local write "Tracking Angle - Right"(w76) -> ()
        n32 = local write "Valid Angles -R"(w75) -> ()
        n33 = local write "Track Angle Valid  - Right"(w63) -> ()
        n34 = local write "New Data  Flag\nRight Servo"(w67) -> ()
      }
    }
    "Right Data\nInput Flag\n- Internal" <- w49
    n35 = case shown="True" w52 {
      tunnel: [w82 w88] -> w48
      tunnel: w60 -> [w82 _]
      tunnel: w56 -> [_ w92]
      tunnel: w57 -> [_ w91]
      frame False {
        # "Don't Update Servo Position\nbc we're waiting on new Data to\ncome in and the servo position\nwas set at the previous set of data"
      }
      frame True {
        w88 = TRUE
        # "Store Values"
        # "Raise Internal Flag"
        # "If New Data Available"
        # "Perforrm Indivudual Angle Calculation"
        # "Pull Down Individual Flag"
        n36 = shared-variable ".\\Localization_Variables_r0.lvlib\\LEFT_BEACON_X_array"() -> (w98:dbl[])  [unwired: 1 in, 1 out]
        "LEFT Beacon Coord - X px (IN) 2" <- w98
        n37 = shared-variable "RT myRIO Target - Overlord\\Localization_Variables_r0.lvlib\\LEFT_BEACON_Scales"() -> (→"Beacon Scales - Left":sgl[])  [unwired: 1 in, 1 out]
        n38 = shared-variable "RT myRIO Target - Overlord\\Localization_Variables_r0.lvlib\\LEFT_BEACON_Y_array"() -> (w99:dbl[])  [unwired: 1 in, 1 out]
        "LEFT Beacon Position - Y px (IN) 2" <- w99
        n39 = shared-variable "RT myRIO Target - Overlord\\Localization_Variables_r0.lvlib\\LEFT_BEACON_BOOL_array"() -> (w100:bool[])  [unwired: 1 in, 1 out]
        "Beacons Found\n- Left (Bool Array) 2" <- w100
        n40 = shared-variable "RT myRIO Target - Overlord\\Localization_Variables_r0.lvlib\\Image Lock - L"() -> (w89:bool)  [unwired: 1 in, 1 out]
        n41 = shared-variable "RT myRIO Target - Overlord\\Localization_Variables_r0.lvlib\\Info - Left"() -> (w85:T5)  [unwired: 1 in, 1 out]
        n42 = Unbundle By Name(w85) -> ("Tracking Coordinates"=w84:cluster{"X":dbl, "Y":dbl}, "Current Valid"=w83:bool, "Current State - Out"=→"Current Cam State - L":T6)
        n43 = local write "Image Lock - Left"(w89) -> ()
        n44 = Bundle("Array of Double"=w98, "Array of Double"=w99) -> (w96:T7)  [unwired: 1 in]
        "Beacon Coordinates - Left Image" <- w96
        n45 = shared-variable "RT myRIO Target - Overlord\\Localization_Variables_r0.lvlib\\Left Servo Angle_Image"() -> (w90:dbl)  [unwired: 1 in, 1 out]
        "This Servo \nAngle - Left" <- w90
        n46 = shared-variable "RT myRIO Target - Overlord\\Localization_Variables_r0.lvlib\\Left_Flag"(FALSE) -> ()  [unwired: 1 in, 1 out]
        n47 = feedback #3() -> (w102:sgl[])  [unwired: 1 in]
        n48 = feedback #4() -> (w101:bool[])  [unwired: 1 in]
        n49 = call "Angle Calc_Individual Process R4.vi"("Angle to Pixel Ratios"=w92, "Previous Angles"=w102, "Num of Beacons"=w91, "Beacon Coordinates - Image"=w96, "Current Servo Angle"=w90, "Beacons Found (Bool Array)"=w100, "Previous Valid Angles"=w101, "Tracking Coordinates"=w84) -> ("Servo Goal Angle"=w95:sgl, "Valid Beacons (Bool Array)\nPosition Calc"=w94:bool[], "Angle Of Beacons \nRelative to Robot"=w93:sgl[])  [unwired: 4 in, 1 out]
        n50 = feedback-in #3(w93) -> ()
        n51 = feedback-in #4(w94) -> ()
        n52 = local write "Beacon Angles - L"(w93) -> ()
        n53 = local write "Valid Angles - L"(w94) -> ()
        n54 = local write "Tracking Angle - Left"(w95) -> ()
        n55 = local write "Track Angle Valid - Left"(w83) -> ()
        n56 = local write "New Data  Flag\nLeft Servo"(w88) -> ()
      }
    }
    "Left Data\nInput Flag\n- Internal" <- w48
    n57 = And(x=w48, y=w49) -> (x .and. y?=w59:bool)
    n58 = case shown="True" w59 {
      selector: w59 -> [_ w105]
      tunnel: w48 -> [w104 _]
      tunnel: [w104 w106] -> w55
      tunnel: [w103 w106] -> w54
      tunnel: w49 -> [w103 _]
      frame False {
      }
      frame True {
        w106 = FALSE
        # "Reset Internal Data Flags"
        # "Position Data\nReady Enabled"
        n59 = local write "Position Calc\nReady"(w105) -> ()
      }
    }
  }
  n60 = Bundle(w34, w34) -> (w37:cluster{sgl, sgl})  [unwired: 1 in]
  n61 = Initialize Array(w34, "History Size") -> (w32:sgl[])
  n62 = Initialize Array(w37, "History Size") -> (w33:cluster{sgl, sgl}[])
  n63 = Initialize Array(FALSE, "History Size") -> (w31:bool[])
  n64 = call "Tick Count4"() -> ("Tick Count(uSec)"=w30:u32)
  n65 = while {
    shift-right: [w117] -> _
    shift-left: w32 -> [w114]
    shift-right: [w116] -> _
    shift-left: w31 -> [w115]
    shift-right: [w118] -> _
    shift-left: w33 -> [w109]
    shift-right: [w110] -> _
    shift-left: w30 -> [w111]
    stop <- "stop" stop-if-true
    n66 = call "Wait5"("Count(mSec)"="Position Calc\nTimer") -> ()  [unwired: 1 out]
    n67 = case shown="True" "Position Calc\nReady" {
      selector: "Position Calc\nReady" -> [_ w161]
      tunnel: w109 -> [_ w184]
      tunnel: w109 -> [w127 w178]
      tunnel: w114 -> [w129 w177]
      tunnel: w115 -> [w128 w176]
      tunnel: [w129 w183] -> w117
      tunnel: [w128 w181] -> w116
      tunnel: [w127 w182] -> w118
      tunnel: w115 -> [_ w175]
      tunnel: w114 -> [_ w174]
      tunnel: [w126 w168] -> w112
      tunnel: w111 -> [_ w168]
      tunnel: [FALSE TRUE] -> w113
      tunnel: w109 -> [_ w163]
      frame False {
        n68 = call "Tick Count5"() -> ("Tick Count(uSec)"=w126:u32)
      }
      frame True {
        w139 = T1."Long Range" ("Current Cam State - R")
        # "At least 2+ Avaialbe"
        # "***********do for both"
        # "sTATE"
        # "CALCULATE AVERAGE ORIENTATION"
        # "Update Outputs\nif Current Calc is Invalid\n(shouldn't matter)"
        # "Estimate Orienation Based on Previous Position"
        # "****# of previous in history that must be true\nin order for position to be considered \"locked\""
        # "New Position is Valid if both \nOrientation and Positions\nis within range of previous"
        # "Robot Position\n Shift Array"
        # "Position Valid Shift Array"
        # "Orientation Shift Array"
        # "Orientation Value"
        # "Shift & Insert Current Position Valid"
        # "Position Valid\n(orientation)"
        # "Position Valid\n(position)"
        # "Update Shift Registers"
        # "Shift & Insert Current Calculated Orientation"
        # "Shift & Insert Current Robot Position"
        # "UPDATE FINAL OUTPUT\n VALUES"
        n69 = Not(x=w161) -> (.not. x?=w162:bool)
        n70 = local read "Num of Beacons (Total)"() -> (w146:i8)
        n71 = local write "Position Calc\nReady"(w162) -> ()
        n72 = local read "Current Cam State - L"() -> (w140:T1)
        n73 = local read "Current Cam State - R"() -> (w138:T1)
        n74 = local read "Beacon Scales - Left"() -> (w152:sgl[])
        n75 = local read "Beacon Scales - Right"() -> (w155:sgl[])
        n76 = Equal?(x=w140, y=w139) -> (x = y?=w136:bool)
        n77 = Equal?(x=w138, y=w139) -> (x = y?=w135:bool)
        n78 = And(x=w136, y=w135) -> (x .and. y?=w137:bool)
        n79 = case shown="False" w137 {
          tunnel: "Beacon Angles - L" -> [w502 w627]
          tunnel: w146 -> [w501 w615]
          tunnel: w152 -> [w500 _]
          tunnel: "Beacon Angles -R" -> [w499 w626]
          tunnel: w155 -> [w498 _]
          tunnel: "Valid Angles -R" -> [w497 w631]
          tunnel: "Valid Angles - L" -> [w496 w632]
          tunnel: "Distance Between \nCameras  (*unit)" -> [w495 w628]
          tunnel: [w494 w610] -> w145
          tunnel: [w493 w609] -> w148
          tunnel: [w492 w608] -> w147
          frame False {
            # "System is not in NORMAL (long range) Mode"
            # "Estimate Distance for each Available Beacon Angle\nPER Camera, indivduallly"
            n80 = for {
              N: w501 -> [_]
              tunnel: w496 -> [w507] mode=indexing
              tunnel: w502 -> [w516] mode=indexing
              tunnel: w500 -> [w517] mode=indexing
              tunnel: w497 -> [w506] mode=indexing
              tunnel: w499 -> [w515] mode=indexing
              tunnel: w498 -> [w514] mode=indexing
              tunnel: w495 -> [w513]
              tunnel: [w505] -> w493 mode=indexing
              tunnel: [w504] -> w492 mode=indexing
              tunnel: [w503] -> w494 mode=indexing
              # "dY"
              # "dX"
              # "Valid"
              # "If Both Cameras are using Same Beacon Data,\nAverage the 2 independently esitmated positions"
              # "dY"
              # "dX"
              # "dY"
              # "dX"
              n81 = case shown="True" w507 {
                tunnel: w516 -> [_ w594]
                tunnel: [w581 w585] -> w511
                tunnel: [w581 w586] -> w510
                tunnel: w517 -> [_ w584]
                frame False {
                  w581 = sgl 0.0
                  # "Current Data Set Was Not Valid\nFill with 0\nWill not be used later"
                }
                frame True {
                  # "Estimate Distance"
                  # "Negate dX if A2>90"
                  # "Find LOCAL Coordinate of Each Beacon"
                  # "Current - Valid Data Set"
                  n82 = call "Scaling and Mapping"("Signals"=w584) -> ("Scaled Signals"=w583:dynamicdata)  [unwired: 9 in, 1 out]
                  n83 = To Single Precision Float(number=w583) -> (single precision float=w582:sgl)
                  n84 = Less?(x=w594, y=sgl 90.0) -> (x < y?=w596:bool)
                  n85 = case shown="False" w596 {
                    tunnel: w594 -> [w603 w605]
                    tunnel: [w601 w606] -> w593
                    tunnel: [FALSE TRUE] -> w588
                    frame False {
                      # "Negative Y"
                      # "A2 is > 90"
                      n86 = Subtract(x=w603, y=sgl 90.0) -> (x-y=w601:sgl)
                    }
                    frame True {
                      # "Positive Y"
                      # "A2 is < 90"
                      n87 = Subtract(x=sgl 90.0, y=w605) -> (x-y=w606:sgl)
                    }
                  }
                  "dA2 2" <- w593
                  n88 = expression code="(x/180.0)*pi" "degrees to radians"(w593) -> (w591:sgl)
                  n89 = expression code="(x/180.0)*pi" "degrees to radians"(w593) -> (w592:sgl)
                  n90 = Cosine(x=w591) -> (cos(x)=w589:sgl)
                  n91 = Sine(x=w592) -> (sin(x)=w590:sgl)
                  n92 = Multiply(x=w582, y=w589) -> (x*y=w586:sgl)
                  n93 = Multiply(x=w582, y=w590) -> (x*y=w587:sgl)
                  n94 = case shown="True" w588 {
                    tunnel: w587 -> [w598 w599]
                    tunnel: [w597 w599] -> w585
                    frame False {
                      n95 = Negate(x=w598) -> (-x=w597:sgl)
                    }
                    frame True {
                    }
                  }
                }
              }
              n96 = case shown="True" w506 {
                tunnel: w515 -> [_ w567]
                tunnel: [w552 w554] -> w509
                tunnel: [w552 w553] -> w508
                tunnel: w514 -> [_ w559]
                tunnel: w513 -> [_ w556]
                frame False {
                  w552 = sgl 0.0
                  # "Current Data Set Was Not Valid\nFill with 0\nWill not be used later"
                }
                frame True {
                  # "Add delta for\nRIGHT camera ONLY"
                  # "Estimate Distance"
                  # "Negate dX if A2>90"
                  # "Find LOCAL Coordinate of Each Beacon"
                  # "Current - Valid Data Set"
                  n97 = call "Scaling and Mapping2"("Signals"=w559) -> ("Scaled Signals"=w558:dynamicdata)  [unwired: 9 in, 1 out]
                  n98 = To Single Precision Float(number=w558) -> (single precision float=w557:sgl)
                  n99 = Less?(x=w567, y=sgl 90.0) -> (x < y?=w569:bool)
                  n100 = case shown="False" w569 {
                    tunnel: w567 -> [w576 w578]
                    tunnel: [w574 w579] -> w566
                    tunnel: [FALSE TRUE] -> w561
                    frame False {
                      # "Negative Y"
                      # "A2 is > 90"
                      n101 = Subtract(x=w576, y=sgl 90.0) -> (x-y=w574:sgl)
                    }
                    frame True {
                      # "Positive Y"
                      # "A2 is < 90"
                      n102 = Subtract(x=sgl 90.0, y=w578) -> (x-y=w579:sgl)
                    }
                  }
                  "dA2 3" <- w566
                  n103 = expression code="(x/180.0)*pi" "degrees to radians"(w566) -> (w564:sgl)
                  n104 = expression code="(x/180.0)*pi" "degrees to radians"(w566) -> (w565:sgl)
                  n105 = Cosine(x=w564) -> (cos(x)=w562:sgl)
                  n106 = Sine(x=w565) -> (sin(x)=w563:sgl)
                  n107 = Multiply(x=w557, y=w562) -> (x*y=w553:sgl)
                  n108 = Multiply(x=w557, y=w563) -> (x*y=w560:sgl)
                  n109 = case shown="True" w561 {
                    tunnel: w560 -> [w571 w572]
                    tunnel: [w570 w572] -> w555
                    frame False {
                      n110 = Negate(x=w571) -> (-x=w570:sgl)
                    }
                    frame True {
                    }
                  }
                  n111 = Add(x=w556, y=w555) -> (x+y=w554:sgl)
                }
              }
              n112 = And(x=w507, y=w506) -> (x .and. y?=w512:bool)
              n113 = case shown="False" w512 {
                tunnel: w511 -> [w525 w551]
                tunnel: w510 -> [w522 w550]
                tunnel: w509 -> [w524 w549]
                tunnel: w508 -> [w523 w548]
                tunnel: [w520 w544] -> w505
                tunnel: [w519 w543] -> w504
                tunnel: w507 -> [w521 _]
                tunnel: w506 -> [w526 _]
                tunnel: [w518 TRUE] -> w503
                frame False {
                  n114 = Exclusive Or(1:w526, 2:w521) -> (0:w527:bool)
                  n115 = case shown="True" w527 {
                    tunnel: w525 -> [_ w535]
                    tunnel: w524 -> [_ w532]
                    tunnel: w523 -> [_ w531]
                    tunnel: w522 -> [_ w533]
                    tunnel: w521 -> [_ w537]
                    tunnel: [w528 w536] -> w520
                    tunnel: [w528 w534] -> w519
                    tunnel: [FALSE TRUE] -> w518
                    frame False {
                      w528 = sgl 0.0
                      # "None are valid,"
                    }
                    frame True {
                      # "Only 1 beacon is valid,\nUse the valid beacon"
                      n116 = case shown="False" w537 {
                        tunnel: [w539 w541] -> w536
                        tunnel: w535 -> [_ w541]
                        tunnel: [w538 w540] -> w534
                        tunnel: w533 -> [_ w540]
                        tunnel: w532 -> [w539 _]
                        tunnel: w531 -> [w538 _]
                        frame False {
                          # "Left is invalid,\nRight MUST be valid"
                        }
                        frame True {
                          # "Left is Valid"
                        }
                      }
                    }
                  }
                }
                frame True {
                  w545 = sgl 2.0 ("y")
                  # "Both are Valid"
                  n117 = Add(x=w551, y=w549) -> (x+y=w546:sgl)
                  n118 = Add(x=w550, y=w548) -> (x+y=w547:sgl)
                  n119 = Divide(x=w547, y=w545) -> (x/y=w543:sgl)
                  n120 = Divide(x=w546, y=w545) -> (x/y=w544:sgl)
                }
              }
            }
          }
          frame True {
            # "dY"
            # "dX"
            # "Valid"
            # "Find Local Coordinates"
            # "Valid COunt"
            # "Make sure 2+ Data Sets are Still available"
            # "Check 1st element\nwith rest of elements"
            # "Make Sure all Pointed \nIn Same Direction"
            # "For Each Valid Beacon\nCalculate Distance from Each Camera to Each Beacon"
            # "Find Common Beacons\nAmong Cameras"
            # "Currently will only\ncalculate position if 2+ \nbeacons are available \nfrom both cameras"
            # "System is in Normal (long range) State"
            n121 = And(x=w632, y=w631) -> (x .and. y?=w636:bool[])
            "Valid Beacon Sets_" <- w636
            n122 = Boolean To (0,1)(Boolean=w636) -> (0, 1=w633:i16[])
            n123 = Add Array Elements(numeric array=w633) -> (sum=w634:i16)
            n124 = Greater?(x=w634, y=1) -> (0:w630:bool)
            n125 = for {
              N: w615 -> [_]
              tunnel: w630 -> [w697]
              tunnel: w627 -> [w696] mode=indexing
              tunnel: w626 -> [w695] mode=indexing
              tunnel: w628 -> [w694]
              tunnel: "Distance Threshold\nRef Triangles (*unit)" -> [w693]
              tunnel: [w692] -> w613 mode=indexing
              tunnel: [w691] -> _ mode=indexing
              tunnel: [w690] -> w612 mode=indexing
              tunnel: [w689] -> _ mode=indexing
              tunnel: [w688] -> w614 mode=indexing
              tunnel: [w687] -> w621 mode=indexing
              n126 = case shown="True" w697 {
                tunnel: w696 -> [w702 w712]
                tunnel: w695 -> [w701 w711]
                tunnel: w694 -> [_ w703]
                tunnel: w693 -> [_ w704]
                tunnel: [w702 w710] -> w692
                tunnel: [w701 w709] -> w691
                tunnel: [FALSE w708] -> w690
                tunnel: [w699 w707] -> w689
                tunnel: [w699 w706] -> w688
                tunnel: [0 w705] -> w687
                frame False {
                  w699 = sgl 1.0
                }
                frame True {
                  # "Build Reference Triangle"
                  n127 = call "Position Calc_Build Reference Triangle_R1.vi"("A2_in"=w712, "A3_in"=w711, "S1 (Length Between\n Cameras - inches)"=w703, "Distance\nThreshold"=w704) -> ("S2"=w707:sgl, "S3"=w706:sgl, "Direction"=w705:i8, "A2"=w710:sgl, "A3"=w709:sgl, "Accept"=w708:bool)  [unwired: 6 in]
                }
              }
            }
            n128 = for {
              N: w615 -> [_]
              tunnel: w612 -> [w682] mode=indexing
              tunnel: w621 -> [w686] mode=indexing
              tunnel: [w686] -> w623 mode=indexing if=w682
              shift-right: [w685] -> w617
              shift-left: 0 -> [w683]
              # "Only add to array\nif valid distance"
              n129 = Increment(x=w683) -> (x+1=w684:i32)
              n130 = Select(t=w684, s=w682, f=w683) -> (s? t:f=w685:i32)
            }
            n131 = Index Array(array=w623, index=0) -> (element=w624:i32)
            n132 = Equal?(x=w623, y=w624) -> (x = y?=w625:bool[])
            n133 = And Array Elements(Boolean array=w625) -> (logical AND=w619:bool)
            n134 = Greater?(x=w617, y=1) -> (0:w618:bool)
            n135 = And(x=w619, y=w618) -> (x .and. y?=w611:bool)
            n136 = case shown="True" w611 {
              tunnel: w615 -> [w639 w648]
              tunnel: w614 -> [_ w647]
              tunnel: w613 -> [_ w646]
              tunnel: w612 -> [_ w645]
              tunnel: [w638 w644] -> w610
              tunnel: [w637 w643] -> w609
              tunnel: [w637 w642] -> w608
              frame False {
                # "Build Array for False"
                n137 = for {
                  N: w639 -> [_]
                  tunnel: [sgl 0.0] -> w637 mode=indexing
                  tunnel: [FALSE] -> w638 mode=indexing
                }
              }
              frame True {
                n138 = for {
                  N: w648 -> [_]
                  tunnel: w646 -> [w654] mode=indexing
                  tunnel: w647 -> [w653] mode=indexing
                  tunnel: [w652] -> w643 mode=indexing
                  tunnel: [w651] -> w642 mode=indexing
                  tunnel: [w650] -> w644 mode=indexing
                  tunnel: w645 -> [w649] mode=indexing
                  n139 = case shown="True" w649 {
                    selector: w649 -> [w656 w660]
                    tunnel: w654 -> [_ w668]
                    tunnel: [w655 w658] -> w652
                    tunnel: [w655 w659] -> w651
                    tunnel: w653 -> [_ w657]
                    tunnel: [w656 w660] -> w650
                    frame False {
                      w655 = sgl 0.0
                      # "Current Data Set Was Not Valid\nFill with 0\nWill not be used later"
                    }
                    frame True {
                      # "dY"
                      # "dX"
                      # "Negate dX if A2>90"
                      # "Find LOCAL Coordinate of Each Beacon"
                      # "Current - Valid Data Set"
                      n140 = Less?(x=w668, y=sgl 90.0) -> (x < y?=w670:bool)
                      n141 = case shown="False" w670 {
                        tunnel: w668 -> [w677 w679]
                        tunnel: [w675 w680] -> w667
                        tunnel: [FALSE TRUE] -> w662
                        frame False {
                          # "Negative Y"
                          # "A2 is > 90"
                          n142 = Subtract(x=w677, y=sgl 90.0) -> (x-y=w675:sgl)
                        }
                        frame True {
                          # "Positive Y"
                          # "A2 is < 90"
                          n143 = Subtract(x=sgl 90.0, y=w679) -> (x-y=w680:sgl)
                        }
                      }
                      "dA2 4" <- w667
                      n144 = expression code="(x/180.0)*pi" "degrees to radians"(w667) -> (w665:sgl)
                      n145 = expression code="(x/180.0)*pi" "degrees to radians"(w667) -> (w666:sgl)
                      n146 = Cosine(x=w665) -> (cos(x)=w663:sgl)
                      n147 = Sine(x=w666) -> (sin(x)=w664:sgl)
                      n148 = Multiply(x=w657, y=w663) -> (x*y=w659:sgl)
                      n149 = Multiply(x=w657, y=w664) -> (x*y=w661:sgl)
                      n150 = case shown="True" w662 {
                        tunnel: w661 -> [w672 w673]
                        tunnel: [w671 w673] -> w658
                        frame False {
                          n151 = Negate(x=w672) -> (-x=w671:sgl)
                        }
                        frame True {
                        }
                      }
                    }
                  }
                }
              }
            }
          }
        }
        n152 = Boolean To (0,1)(Boolean=w145) -> (0, 1=w144:i16[])
        n153 = Add Array Elements(numeric array=w144) -> (sum=w143:i16)
        n154 = Greater?(x=w143, y=i16 1) -> (0:w141:bool)
        n155 = case shown="True" w141 {
          tunnel: w184 -> [_ w270]
          tunnel: [0.0 ("f") w269] -> w180
          tunnel: [w187 w268] -> w179
          tunnel: w175 -> [_ w267]
          tunnel: w174 -> [_ w266]
          tunnel: [FALSE w265] -> w166
          tunnel: [FALSE w264] -> w165
          tunnel: w163 -> [_ w263]
          tunnel: [sgl 0.0 w261] -> w156
          tunnel: "Distance Between \nCameras  (*unit)" -> [_ w197]
          tunnel: w148 -> [_ w196]
          tunnel: w147 -> [_ w195]
          tunnel: w145 -> [_ w194]
          tunnel: w146 -> [_ w193]
          tunnel: "Moving Average\nWindow Length" -> [_ w191]
          frame False {
            w186 = 0.0 ("f")
            n156 = Bundle("f"=w186, "f"=w186) -> (w187:cluster{"f":dbl, "f":dbl})  [unwired: 1 in]
          }
          frame True {
            w233 = sgl 2.0
            w250 = 0
            # "Only Apply This Filtering \nif 3 or More Beacons Still Valid"
            # "Orientation Value"
            # "Orientation Valid"
            # "Y (current)"
            # "X (current)"
            # "Number of Valid\nPrevious Orientations"
            # "Position Valid Shift Array"
            # "More than 1 Previous\nValid Positions"
            # "More than\n2previous position\navailable"
            # "Choose Beacon Set\nwith Lowest Std Dev"
            # "Y value cannot be negative"
            # "Find New # Of Valid Beacons"
            # "Adjust/Normalize\nLocal Beacon Positions\nusing Line of Best fit"
            # "# Valid\nData Sets"
            # "cam, y"
            # "cam, x"
            # "Calculate dX and dY\nfor right cam"
            # "Average dX and dY from each (valid) beacon to find position of each camera\n\nthen average all  positions for each camera find center between"
            # "Convert Slope\nto Radians"
            # "*rotate CCW in rad"
            # "Rotate Coordinate\n System by Slope"
            n157 = Boolean To (0,1)(Boolean=w267) -> (0, 1=w218:i16[])
            n158 = Add Array Elements(numeric array=w218) -> (sum=w212:i16)
            n159 = Greater?(x=w212, y=w191) -> (0:w192:bool)
            n160 = Bundle(w196, w195) -> (→"LOCAL\nBeacon Coordinates\nRelative to Robot" →"Local Coordinates - Calculated":cluster{sgl[], sgl[]})  [unwired: 1 in]
            n161 = call "Coordinate_Outlier_Filtering_R2.vi"("Num of Beacons"=w193, "Max Std Dev(all 5)"="Max Std Dev (5)", "X in"=w196, "Valid Data\nSets in"=w194, "Y in"=w195, "Max Std Dev( 4 )"="Max Std Dev (4)", "Max Std Dev (3)"="Max Std Dev (3)") -> ("Y out"=w208:sgl[], "X out"=w209:sgl[], "Valid Beacons\nout"=w206:bool[], "Slope out"=w215:dbl)  [unwired: 3 in, 2 out]
            n162 = Inverse Tangent(1:w215) -> (0:w229:dbl)
            n163 = expression code="(x/pi)*180.0" "radians to degrees"(w229) -> (w214:dbl)
            n164 = Boolean To (0,1)(Boolean=w206) -> (0, 1=w205:i16[])
            n165 = To Single Precision Float(number=w214) -> (single precision float=w261:sgl)
            n166 = case shown="True" w192 {
              tunnel: w267 -> [_ w303]
              tunnel: [w280 w291] -> w264
              tunnel: w266 -> [_ w294]
              tunnel: w261 -> [w281 w287]
              tunnel: [w279 w292] -> w269
              tunnel: w263 -> [_ _]
              tunnel: w191 -> [_ w285]
              frame False {
                # "Since no history available,\ncheck that current is with 0-360"
                # "Use Current Orientation bc \nPrevious are not available"
                # "New Position\nValid"
                n167 = In Range and Coerce(upper limit=sgl 360.0, x=w281, lower limit=sgl -360.0 ("upper limit")) -> (In Range?=w280:bool)  [unwired: 1 out]
                n168 = Select(t=w281, s=w280, f=sgl 0.0) -> (s? t:f=w279:sgl)
              }
              frame True {
                # "Moving Average Out"
                # "Valid Position Ccount\n(up to 2)"
                # "Only Calculate MOving Avg\nif xx% of previous positions were valid"
                n169 = Initialize Array(u8 0, w285) -> (w299:u8[])
                n170 = local read "History Size"() -> (w300:u8)
                n171 = while {
                  shift-right: [w328] -> w295
                  shift-left: w299 -> [w330]
                  tunnel: w303 -> [w336] mode=indexing
                  shift-right: [w334] -> w289
                  shift-left: u8 0 -> [w337]
                  tunnel: w300 -> [w335]
                  tunnel: w285 -> [w327]
                  i -> [w329]
                  stop <- w331 stop-if-true
                  # "Grab Last 2 Valid Position Indexes"
                  n172 = case shown="True" w336 {
                    tunnel: w337 -> [w339 w341]
                    tunnel: [w339 w344] -> w334
                    tunnel: w330 -> [w338 w343]
                    tunnel: w329 -> [_ w342]
                    tunnel: [w338 w340] -> w328
                    frame False {
                    }
                    frame True {
                      # "Update Index\nto use"
                      # "Increment\nValid Count"
                      n173 = Replace Array Subset(array=w343, new element=w342, index=w341) -> (w340:u8[])
                      n174 = Increment(x=w341) -> (x+1=w344:u8)
                    }
                  }
                  n175 = Greater?(x=w329, y=w335) -> (0:w332:bool)
                  n176 = Greater Or Equal?(x=w334, y=w327) -> (x >= y?=w333:bool)
                  n177 = Or(x=w333, y=w332) -> (x .or. y?=w331:bool)
                }
                n178 = for {
                  N: w289 -> [_]
                  shift-right: [w326] -> w297
                  shift-left: 0.0 -> [w325]
                  tunnel: w295 -> [w324] mode=indexing
                  tunnel: w294 -> [w322]
                  # "Fetch Last Valid Values\nand Sum"
                  n179 = Index Array(array=w322, index=w324) -> (element=w323:sgl)
                  n180 = Add(x=w323, y=w325) -> (x+y=w326:dbl)
                }
                n181 = Increment(x=w289) -> (x+1=w286:u8)
                n182 = Add(x=w287, y=w297) -> (x+y=w288:dbl)
                n183 = To Double Precision Float(number=w286) -> (double precision float=w296:dbl)
                n184 = Divide(x=w288, y=w296) -> (x/y=w293:dbl)
                n185 = Greater Than 0?(x=w286) -> (x > 0?=w290:bool)
                n186 = case shown="True" w290 {
                  tunnel: w293 -> [w306 w312]
                  tunnel: w295 -> [_ w319]
                  tunnel: w294 -> [_ w318]
                  tunnel: [w305 w311] -> w292
                  tunnel: [w304 w314] -> w291
                  frame False {
                    # "No Pevious is Available to Compare\ncheck that current is real angle"
                    n187 = In Range and Coerce(upper limit=sgl 360.0, x=w306, lower limit=sgl -360.0 ("upper limit")) -> (In Range?=w304:bool)  [unwired: 1 out]
                    n188 = Select(t=w306, s=w304, f=sgl 0.0) -> (s? t:f=w305:dbl)
                  }
                  frame True {
                    # "Calculate New, Weighted\nOrientation"
                    # "Check That New Value\nis within Range of Old\n(avg)"
                    # "(X1 - X2)^2"
                    # "Previous"
                    # "Pevious is Available to Compare"
                    n189 = Index Array(array=w319, index=u8 0) -> (element=w320:u8)
                    n190 = Index Array(array=w318, index=w320) -> (element=w317:sgl)
                    n191 = Subtract(x=w317, y=w312) -> (x-y=w316:dbl)
                    n192 = Absolute Value(x=w316) -> (abs(x)=w315:dbl)
                    n193 = Less Or Equal?(x=w315, y="New Orientation \nThreshold") -> (x <= y?=w314:bool)
                    n194 = Select(t=w312, s=w314, f=sgl 0.0) -> (s? t:f=w311:dbl)
                  }
                }
              }
            }
            n195 = Add Array Elements(numeric array=w205) -> (sum=w204:i16)
            n196 = Greater?(x=w204, y=i16 2) -> (0:w202:bool)
            n197 = case shown="True" w202 {
              tunnel: w193 -> [_ w278]
              tunnel: w206 -> [w271 w277]
              tunnel: w209 -> [_ w276]
              tunnel: w208 -> [_ w275]
              tunnel: [w271 w274] -> w207
              tunnel: "Distance\nBetween Beacons" -> [_ w273]
              tunnel: "Distance\nBetween Beacons \n- Tolerance" -> [_ w272]
              frame False {
                # "Don't apply filtering,\nnot enough data points"
              }
              frame True {
                # "This will filter beacons if they are calculate to be \ntoo close to each other. The beacon(s) that is\n discarded is chosen based distance between each/every\nbeacon,. Capable of filtering as long as 1/2 of sample\nset has uniform distances (between beacons)."
                # "Validate Distance Between\nEach Beacon"
                n198 = call "Beacon_Filtering_Inter_Beacon_Distance_R1.vi"("Num of Beacons"=w278, "Inter Beacon\nReal Distance"=w273, "X in"=w276, "Inter Beacon\ndelta Threshold"=w272, "Y in"=w275, "Valid Data\nSets in"=w277) -> ("Beacons Valid - Out"=w274:bool[])  [unwired: 9 in]
              }
            }
            "Post Filtering\n- Valid Beacons" <- w207
            n199 = Increment(x=w193) -> (x+1=w251:i8)
            n200 = for {
              N: w251 -> [_]
              tunnel: [w482] -> w252 mode=indexing
              tunnel: w209 -> [w478]
              tunnel: w208 -> [w481]
              tunnel: [w480] -> w253 mode=indexing
              tunnel: w197 -> [w477]
              i -> [w479]
              # "Build Array's of Coordinates\nFor All Objects"
              n201 = Greater Than 0?(x=w479) -> (x > 0?=w483:bool)
              n202 = case shown="True" w483 {
                tunnel: [w485 w491] -> w482
                tunnel: w478 -> [w488 _]
                tunnel: w481 -> [w487 _]
                tunnel: [w484 0.0] -> w480
                tunnel: w479 -> [w489 _]
                tunnel: w477 -> [_ w491]
                frame True {
                  # "Rest of Array is\nBeacon Coordinates"
                  n203 = Decrement(x=w489) -> (x-1=w486:i32)
                  n204 = Index Array(array=w488, index=w486) -> (element=w485:sgl)
                  n205 = Index Array(array=w487, index=w486) -> (element=w484:sgl)
                }
                frame False {
                  # "First object is the\nother Camera\n\nthis coordinate\nis simply:\nx = 0\ny = distance btween cams"
                }
              }
            }
            n206 = Bundle(w252, w253) -> (→"All Object Coordinates \n- Local" →"Local Coordinates - Normalized":cluster{sgl[], dbl[]})  [unwired: 1 in]
            n207 = expression code="(x/180.0)*pi" "degrees to radians"(w269) -> (w213:dbl)
            n208 = call-poly <vilib>:"2D Cartesian Coordinate Rotation.vi"("theta"=w213, "Y"=w253, "X"=w252) -> ("Y Out"=w230:dbl[], "X Out"=w231:dbl[])  [unwired: 6 in, 1 out]
            n209 = Bundle("X Out"=w231, "Y Out"=w230) -> (→"All Object Coordinates \n- Local - Rotated" →"Local Coordinates - Rotated":cluster{"X Out":dbl[], "Y Out":dbl[]})  [unwired: 1 in]
            n210 = Index Array(array=w230, index=w250) -> (element=w226:dbl)
            n211 = Index Array(array=w231, index=w250) -> (element=w249:dbl)
            n212 = for {
              N: w193 -> [_]
              tunnel: w230 -> [w473]
              tunnel: w231 -> [w474]
              tunnel: w249 -> [w472]
              tunnel: w226 -> [w471]
              tunnel: [w470] -> w223 mode=indexing
              tunnel: [w469] -> w222 mode=indexing
              tunnel: [w468] -> w199 mode=indexing
              tunnel: [w467] -> w224 mode=indexing
              i -> [w476]
              n213 = Increment(x=w476) -> (x+1=w475:i32)
              n214 = Index Array(array=w473, index=w475) -> (element=w467:dbl)
              n215 = Index Array(array=w474, index=w475) -> (element=w468:dbl)
              n216 = Subtract(x=w467, y=w471) -> (x-y=w469:dbl)
              n217 = Subtract(x=w468, y=w472) -> (x-y=w470:dbl)
            }
            n218 = Bundle(w223, w222) -> (→"dX, dY\nRight Cam":cluster{dbl[], dbl[]})  [unwired: 1 in]
            n219 = Bundle(w199, w224) -> (→"dX, dY\nLeft Cam":cluster{dbl[], dbl[]})  [unwired: 1 in]
            n220 = Unbundle("Real Beacon\n - Coordinates") -> ("X"=w247:dbl[], "Y"=w227:dbl[])
            n221 = Boolean To (0,1)(Boolean=w207) -> (0, 1=w225:i16[])
            n222 = for {
              N: w193 -> [_]
              tunnel: w207 -> [w453] mode=indexing
              tunnel: w247 -> [w450] mode=indexing
              tunnel: w227 -> [w449] mode=indexing
              tunnel: w199 -> [w452] mode=indexing
              tunnel: w224 -> [w448] mode=indexing
              tunnel: w223 -> [w451] mode=indexing
              tunnel: w222 -> [w447] mode=indexing
              tunnel: [w446] -> w246 mode=indexing
              tunnel: [w445] -> w245 mode=indexing
              tunnel: [w444] -> w244 mode=indexing
              tunnel: [w443] -> w243 mode=indexing
              n223 = case shown="True" w453 {
                tunnel: w452 -> [_ w466]
                tunnel: w451 -> [_ w465]
                tunnel: w450 -> [_ w456]
                tunnel: w449 -> [_ w455]
                tunnel: w448 -> [_ w464]
                tunnel: w447 -> [_ w457]
                tunnel: [w454 w462] -> w446
                tunnel: [w454 w461] -> w445
                tunnel: [w454 w460] -> w444
                tunnel: [w454 w459] -> w443
                frame False {
                  w454 = sgl 0.0
                  # "Add Nothing"
                }
                frame True {
                  # "realX = beaconX + dY\nrealY = beaconY + (-dx)"
                  # "Right Cam"
                  # "Left Cam"
                  # "dX = -dX\nSwap dX, dY"
                  # "Translate to Real Coordinates\nOnly Apply for Valid Beacons"
                  n224 = Negate(x=w466) -> (-x=w463:dbl)
                  n225 = Negate(x=w465) -> (-x=w458:dbl)
                  n226 = Add(x=w456, y=w464) -> (x+y=w462:dbl)
                  n227 = Add(x=w455, y=w463) -> (x+y=w461:dbl)
                  n228 = Add(x=w456, y=w457) -> (x+y=w460:dbl)
                  n229 = Add(x=w455, y=w458) -> (x+y=w459:dbl)
                }
              }
            }
            n230 = Add Array Elements(numeric array=w225) -> (sum=w228:i16)
            n231 = Add Array Elements(numeric array=w246) -> (sum=w242:dbl)
            n232 = Add Array Elements(numeric array=w245) -> (sum=w241:dbl)
            n233 = Add Array Elements(numeric array=w244) -> (sum=w240:dbl)
            n234 = Add Array Elements(numeric array=w243) -> (sum=w239:dbl)
            n235 = Divide(x=w242, y=w228) -> (x/y=w238:dbl)
            n236 = Divide(x=w241, y=w228) -> (x/y=w236:dbl)
            n237 = Divide(x=w240, y=w228) -> (x/y=w237:dbl)
            n238 = Divide(x=w239, y=w228) -> (x/y=w235:dbl)
            n239 = Bundle(w238, w236) -> (→"Left Camera Real Coordinates":cluster{dbl, dbl})  [unwired: 1 in]
            n240 = Bundle(w237, w235) -> (→"Right Camera Real Coordinate":cluster{dbl, dbl})  [unwired: 1 in]
            n241 = Add(x=w238, y=w237) -> (x+y=w234:dbl)
            n242 = Add(x=w236, y=w235) -> (x+y=w232:dbl)
            n243 = local read "Moving Average\nWindow Length"() -> (w198:u8)
            n244 = Divide(x=w234, y=w233) -> (x/y=w217:dbl)
            n245 = Divide(x=w232, y=w233) -> (x/y=w216:dbl)
            n246 = case shown="True" w192 {
              tunnel: w267 -> [_ w388]
              tunnel: w212 -> [_ _]
              tunnel: w217 -> [w349 w365]
              tunnel: [w350 w379] -> w265
              tunnel: w270 -> [_ w367]
              tunnel: w216 -> [w348 w364]
              tunnel: [w347 w387] -> w268
              tunnel: "Max X (arena)" -> [w346 w378]
              tunnel: "Max Y (arena)" -> [w345 w377]
              tunnel: w198 -> [_ w371]
              frame False {
                # "New Position\nValid"
                # "Since no history available,\ncheck that current is within\nthe bounds of the arena size"
                # "Use Current Position bc \nPrevious are not available"
                n247 = In Range and Coerce(upper limit=w346, x=w349, lower limit=sgl 0.0 ("upper limit")) -> (In Range?=w352:bool)  [unwired: 1 out]
                n248 = In Range and Coerce(upper limit=w345, x=w348, lower limit=sgl 0.0 ("upper limit")) -> (In Range?=w351:bool)  [unwired: 1 out]
                n249 = Bundle(w349, w348) -> (w347:cluster{dbl, dbl})  [unwired: 1 in]
                n250 = And(x=w352, y=w351) -> (x .and. y?=w350:bool)
              }
              frame True {
                w376 = 0.0
                # "If needed, make seperate FOR Loop for \nY only... Using more previous values than X"
                # "New Y"
                # "New X"
                # "Only consider if velocity is\ngreater than certain speed"
                # "Valid Position Ccount\n(up to 2)"
                # "Weighted Robot \nCoordinates"
                # "Position\nValid\n(current)"
                # "Only Calculate MOving Avg\nif xx% of previous positions were valid"
                n251 = Initialize Array(u8 0, w371) -> (w383:u8[])
                n252 = local read "History Size"() -> (w384:u8)
                n253 = while {
                  shift-right: [w427] -> w368
                  shift-left: w383 -> [w429]
                  tunnel: w388 -> [w434] mode=indexing
                  shift-right: [w432] -> w375
                  shift-left: u8 0 -> [w435]
                  tunnel: w384 -> [w433]
                  tunnel: [w426] -> _
                  tunnel: w371 -> [w425]
                  i -> [w428]
                  stop <- w430 stop-if-true
                  # "Grab Last 3 Valid Position Indexes"
                  n254 = case shown="True" w434 {
                    tunnel: w435 -> [w437 w439]
                    tunnel: [w437 w442] -> w432
                    tunnel: w429 -> [w436 w441]
                    tunnel: w428 -> [_ w440]
                    tunnel: [w436 w438] -> w427
                    frame False {
                    }
                    frame True {
                      # "Update Index\nto use"
                      # "Increment\nValid Count"
                      n255 = Replace Array Subset(array=w441, new element=w440, index=w439) -> (w438:u8[])
                      n256 = Increment(x=w439) -> (x+1=w442:u8)
                    }
                  }
                  n257 = Greater?(x=w428, y=w433) -> (0:w431:bool)
                  n258 = Greater Or Equal?(x=w432, y=w425) -> (x >= y?=w426:bool)
                  n259 = Or(x=w426, y=w431) -> (x .or. y?=w430:bool)
                }
                n260 = for {
                  N: w375 -> [_]
                  shift-right: [w397] -> w360
                  shift-left: w376 -> [w396]
                  shift-right: [w395] -> w359
                  shift-left: w376 -> [w394]
                  tunnel: w368 -> [w392] mode=indexing
                  tunnel: w367 -> [w390]
                  # "Fetch Last Valid Values\nand Sum"
                  n261 = Index Array(array=w390, index=w392) -> (element=w391:cluster{sgl, sgl})
                  n262 = Unbundle(w391) -> (w393:sgl, w389:sgl)
                  n263 = Add(x=w389, y=w394) -> (x+y=w395:dbl)
                  n264 = Add(x=w393, y=w396) -> (x+y=w397:dbl)
                }
                n265 = Increment(x=w375) -> (x+1=w366:u8)
                n266 = Subtract(x=1.0, y="New Position\nWeight") -> (x-y=w361:dbl)
                n267 = Multiply(x=w360, y=w361) -> (x*y=w358:dbl)
                n268 = Multiply(x=w365, y="New Position\nWeight") -> (x*y=w355:dbl)
                n269 = Add(x=w358, y=w355) -> (x+y=w370:dbl)
                n270 = To Single Precision Float(number=w366) -> (single precision float=w374:sgl)
                n271 = Multiply(x=w359, y=w361) -> (x*y=w357:dbl)
                n272 = Multiply(x=w364, y="New Position\nWeight") -> (x*y=w356:dbl)
                n273 = Add(x=w356, y=w357) -> (x+y=w369:dbl)
                n274 = Divide(x=w370, y=w374) -> (x/y=w373:dbl)
                n275 = Divide(x=w369, y=w374) -> (x/y=w372:dbl)
                n276 = Greater Than 0?(x=w366) -> (x > 0?=w382:bool)
                n277 = case shown="True" w382 {
                  tunnel: w373 -> [w402 w409]
                  tunnel: w372 -> [w401 w408]
                  tunnel: w368 -> [_ w421]
                  tunnel: w367 -> [_ w420]
                  tunnel: [w399 w409] -> w381
                  tunnel: [w398 w408] -> w380
                  tunnel: [w403 w410] -> w379
                  tunnel: w378 -> [w405 _]
                  tunnel: w377 -> [w404 _]
                  frame False {
                    w400 = sgl 0.0 ("upper limit")
                    # "Check that within bounds of arena"
                    # "No Pevious is Available to Compare"
                    n278 = In Range and Coerce(upper limit=w405, x=w402, lower limit=w400) -> (In Range?=w407:bool)  [unwired: 1 out]
                    n279 = In Range and Coerce(upper limit=w404, x=w401, lower limit=w400) -> (In Range?=w406:bool)  [unwired: 1 out]
                    n280 = And(x=w407, y=w406) -> (x .and. y?=w403:bool)
                    n281 = Select(t=w402, s=w403, f=w400) -> (s? t:f=w399:dbl)
                    n282 = Select(t=w401, s=w403, f=w400) -> (s? t:f=w398:dbl)
                  }
                  frame True {
                    # "New"
                    # "(Y1 - Y2)^2"
                    # "(X1 - X2)^2"
                    # "Previous"
                    # "Pevious is Available to Compare"
                    n283 = Index Array(array=w421, index=u8 0) -> (element=w423:u8)
                    n284 = Index Array(array=w420, index=w423) -> (element=w422:cluster{sgl, sgl})
                    n285 = Unbundle(w422) -> (w412:sgl, w411:sgl)
                    n286 = Subtract(x=w412, y=w409) -> (x-y=w417:dbl)
                    n287 = Subtract(x=w408, y=w411) -> (x-y=w416:dbl)
                    n288 = Square(x=w417) -> (x^2=w415:dbl)
                    n289 = Square(x=w416) -> (x^2=w414:dbl)
                    n290 = Add(x=w415, y=w414) -> (x+y=w418:dbl)
                    n291 = Square Root(x=w418) -> (sqrt(x)=w413:dbl)
                    n292 = Less Or Equal?(x=w413, y="New Position \nThreshold") -> (x <= y?=w410:bool)
                  }
                }
                n293 = Bundle("upper limit"=w381, "upper limit"=w380) -> (w387:cluster{"upper limit":dbl, "upper limit":dbl})  [unwired: 1 in]
              }
            }
            n294 = Bundle(w217, w216) -> (→"Robot Coordinates":cluster{dbl, dbl})  [unwired: 1 in]
            n295 = Less Than 0?(x=w216) -> ()  [unwired: 1 out]
          }
        }
        "Orietnation\n(current)" <- w156
        n296 = And(x=w166, y=w165) -> (x .and. y?=w169:bool)
        "Position Valid" <- w169
        n297 = Exclusive Or(1:w165, 2:w166) -> (0:w164:bool)
        n298 = case shown="True" w169 {
          tunnel: [w719 w722] -> w132
          tunnel: [w720 w721] -> w134
          tunnel: w180 -> [_ w722]
          tunnel: w179 -> [_ w721]
          tunnel: w164 -> [_ _]
          frame False {
            w719 = sgl 0.0 ("f")
            n299 = Bundle("f"=w719, "f"=w719) -> (w720:cluster{"f":sgl, "f":sgl})  [unwired: 1 in]
          }
          frame True {
            # "For Servos"
            "Last Orientation" <- w722
            "Last Position" <- w721
          }
        }
        "Robot Coordinates - Avgd" <- w134
        "Orientation Avgd" <- w132
        n300 = local read "History Size"() -> (w158:u8)
        n301 = Decrement(x=w158) -> (x-1=w159:u8)
        n302 = for {
          N: w158 -> [_]
          shift-right: [w760] -> w182
          shift-left: w178 -> [w759]
          tunnel: w134 -> [w758]
          tunnel: w159 -> [w757]
          i -> [w756]
          n303 = Subtract(x=w757, y=w756) -> (x-y=w755:i32)
          n304 = Equal To 0?(x=w755) -> (x = 0?=w754:bool)
          n305 = case shown="False" w754 {
            tunnel: w755 -> [w762 w767]
            tunnel: w759 -> [w765 w768]
            tunnel: [w763 w769] -> w760
            tunnel: w758 -> [_ w766]
            frame False {
              n306 = Decrement(x=w762) -> (x-1=w761:i32)
              n307 = Index Array(array=w765, index=w761) -> (element=w764:cluster{sgl, sgl})
              n308 = Replace Array Subset(array=w765, new element=w764, index=w762) -> (w763:cluster{sgl, sgl}[])
            }
            frame True {
              n309 = Replace Array Subset(array=w768, new element=w766, index=w767) -> (w769:cluster{sgl, sgl}[])
            }
          }
        }
        n310 = Decrement(x=w158) -> (x-1=w160:u8)
        n311 = for {
          N: w158 -> [_]
          shift-right: [w744] -> w183
          shift-left: w177 -> [w743]
          tunnel: w132 -> [w742]
          tunnel: w160 -> [w741]
          i -> [w740]
          n312 = Subtract(x=w741, y=w740) -> (x-y=w738:i32)
          n313 = Equal To 0?(x=w738) -> (x = 0?=w739:bool)
          n314 = case shown="False" w739 {
            tunnel: w738 -> [w746 w751]
            tunnel: w743 -> [w749 w752]
            tunnel: [w747 w753] -> w744
            tunnel: w742 -> [_ w750]
            frame False {
              # "Shift"
              n315 = Decrement(x=w746) -> (x-1=w745:i32)
              n316 = Index Array(array=w749, index=w745) -> (element=w748:sgl)
              n317 = Replace Array Subset(array=w749, new element=w748, index=w746) -> (w747:sgl[])
            }
            frame True {
              # "insert new"
              n318 = Replace Array Subset(array=w752, new element=w750, index=w751) -> (w753:sgl[])
            }
          }
        }
        n319 = Decrement(x=w158) -> (x-1=w157:u8)
        n320 = for {
          N: w158 -> [_]
          shift-right: [w729] -> w181
          shift-left: w176 -> [w728]
          tunnel: w169 -> [w727]
          tunnel: w157 -> [w726]
          i -> [w725]
          n321 = Subtract(x=w726, y=w725) -> (x-y=w723:i32)
          n322 = Equal To 0?(x=w723) -> (x = 0?=w724:bool)
          n323 = case shown="False" w724 {
            tunnel: w728 -> [w734 w736]
            tunnel: [w732 w737] -> w729
            tunnel: w727 -> [_ w735]
            tunnel: w723 -> [w730 _]
            frame False {
              n324 = Decrement(x=w730) -> (x-1=w731:i32)
              n325 = Index Array(array=w734, index=w731) -> (element=w733:bool)
              n326 = Replace Array Subset(array=w734, new element=w733, index=w730) -> (w732:bool[])
            }
            frame True {
              n327 = Replace Array Subset(array=w736, new element=w735) -> (w737:bool[])  [unwired: 1 in]
            }
          }
        }
        n328 = Boolean To (0,1)(Boolean=w181) -> (0, 1=w173:i16[])
        n329 = Add Array Elements(numeric array=w173) -> (sum=w171:i16)
        n330 = Greater Or Equal?(x=w171, y=i16 5) -> (x >= y?=→"Position \nLock Status":bool)
        n331 = case shown="True" w169 {
          tunnel: w134 -> [_ w718]
          frame False {
          }
          frame True {
            # "update debug graph\nif current is valid"
            n332 = Unbundle(w718) -> ("upper limit"=w717:dbl, "upper limit"=w716:dbl)
            n333 = Build Array(w716) -> (w714:dbl[])
            n334 = Build Array(w717) -> (w715:dbl[])
            n335 = Bundle(w715, w714) -> (→"Real Position in Course 2":cluster{dbl[], dbl[]})  [unwired: 1 in]
          }
        }
        n336 = Unbundle(w134) -> ("upper limit"=w133:dbl, "upper limit"=w131:dbl)
        n337 = shared-variable "RT myRIO Target - Overlord\\Localization_Variables_r0.lvlib\\loc_x"(w133) -> ()  [unwired: 1 in, 1 out]
        n338 = shared-variable "RT myRIO Target - Overlord\\Localization_Variables_r0.lvlib\\loc_y"(w131) -> ()  [unwired: 1 in, 1 out]
        n339 = shared-variable "RT myRIO Target - Overlord\\Localization_Variables_r0.lvlib\\loc_theta"(w132) -> ()  [unwired: 1 in, 1 out]
      }
    }
    n340 = case shown="True" w113 {
      tunnel: w112 -> [_ w120]
      frame False {
      }
      frame True {
        n341 = call "Tick Count3"() -> ("Tick Count(uSec)"=w121:u32)
        n342 = Subtract(x=w121, y=w120) -> (x-y=w124:u32)
        n343 = Divide(x=w124, y=u32 1000 ("x")) -> (x/y=→"dT":dbl)
      }
    }
    n344 = call "Tick Count6"() -> ("Tick Count(uSec)"=w110:u32)
    "Robot Coordinates\nHistory" <- w109
    "Orientation\nHistory" <- w114
    "Position Valid\nHistory" <- w115
  }
  n345 = disable-structure shown="Enabled" {
    disable-tunnel: [w772 _] -> _
    disable-tunnel: ["Search Step Size\n(deg)" _] -> _
    frame Enabled {
      n346 = Multiply(x=3.413333333333333, y="Search Step Size\n(deg)") -> (x*y=w770:dbl)
      n347 = To Unsigned Word Integer(number=w770) -> (unsigned 16bit integer=w772:u16)
    }
    frame Disabled {
    }
  }
  n348 = Multiply(x="Move Servo\nThreshold (deg)", y=3.413333333333333) -> (x*y=w18:dbl)
  n349 = To Unsigned Word Integer(number=w18) -> ()  [unwired: 1 out]
  n350 = call "Tick Count8"() -> ()  [unwired: 1 out]
  n351 = flat-sequence {
    tunnel: [w776] -> w42
    tunnel: [w775] -> w41
    tunnel: [w780] -> w40
    tunnel: ["Left Servo\nID"] -> w29
    tunnel: ["Right Servo\nID"] -> w28
    tunnel: ["Compliance Slope"] -> w27
    tunnel: [w820] -> w39
    tunnel: [w819] -> w38
    tunnel: w42 -> [w818]
    tunnel: w41 -> [w817]
    tunnel: w40 -> [w816]
    tunnel: w29 -> [w814]
    tunnel: w28 -> [w813]
    tunnel: w27 -> [w812]
    tunnel: w39 -> [w1093]
    tunnel: w38 -> [w1092]
    frame #0 {
      # "BAUD RATE"
      # "Initialize UART and DIO"
      n352 = call-poly "VISA Configure Serial Port"("VISA resource name"=refnum<visa-resource-name> "ASRL1::INSTR", "Enable Termination\nChar (T)"=FALSE ("Enable Termination\nChar (T)"), "baud rate (9600)"=u32 115200) -> ("VISA resource name out"=w776:refnum<visa-resource-name>)  [unwired: 11 in, 1 out]
      n353 = call <vilib>:"Smart Open.vi"("Channel Names"=tag[] ["A/DIO2"]) -> ("DIO Ref Out"=w775:T8)  [unwired: 9 in, 1 out]
      n354 = flat-sequence {
        tunnel: w776 -> [w788]
        tunnel: w775 -> [w787]
        tunnel: "Left Servo\nID" -> [w789]
        tunnel: [w786] -> w777
        tunnel: "Compliance Slope" -> [w785]
        tunnel: "Right Servo\nID" -> [w802]
        tunnel: w777 -> [w801]
        tunnel: "Compliance Slope" -> [w800]
        tunnel: w776 -> [w799]
        tunnel: w775 -> [w798]
        frame #0 {
          w786 = 3
          n355 = while {
            tunnel: w786 -> [w795]
            tunnel: w788 -> [w793]
            tunnel: w787 -> [w792]
            tunnel: w789 -> [w791]
            tunnel: w785 -> [w790]
            i -> [w796]
            stop <- w794 stop-if-true
            n356 = call "Set_Compliance_Slope_R2.vi"("Compliance Slope"=w790, "DIO Ref Out"=w792, "VISA resource name"=w793, "Servo ID"=w791) -> ()  [unwired: 6 in, 2 out]
            n357 = Increment(x=w796) -> (x+1=w797:i32)
            n358 = Greater Or Equal?(x=w797, y=w795) -> (x >= y?=w794:bool)
          }
        }
        frame #1 {
          n359 = while {
            tunnel: w801 -> [w808]
            tunnel: w802 -> [w806]
            tunnel: w799 -> [w805]
            tunnel: w798 -> [w804]
            tunnel: w800 -> [w803]
            i -> [w809]
            stop <- w807 stop-if-true
            n360 = call "Set_Compliance_Slope_R2.vi"("Compliance Slope"=w803, "DIO Ref Out"=w804, "VISA resource name"=w805, "Servo ID"=w806) -> ()  [unwired: 6 in, 2 out]
            n361 = Increment(x=w809) -> (x+1=w810:i32)
            n362 = Greater Or Equal?(x=w810, y=w808) -> (x >= y?=w807:bool)
          }
        }
      }
      n363 = call "Tick Count"() -> ("Tick Count(uSec)"=w780:u32)
    }
    frame #1 {
      # "Service Count"
      n364 = while {
        shift-right: [w823] -> _
        shift-left: w816 -> [w840]
        tunnel: "Max Write\nTx Attempts" -> [w835]
        tunnel: "Max Read\nTx Attempts" -> [w834]
        shift-right: [w830] -> w820
        shift-left: w818 -> [w833]
        shift-right: [w829] -> w819
        shift-left: w817 -> [w832]
        tunnel: w814 -> [w828]
        tunnel: w813 -> [w827]
        tunnel: w812 -> [w826]
        shift-right: [w824] -> _
        shift-left: u16 0 -> [w825]
        stop <- "close comms" stop-if-true
        # "Loop Timer"
        n365 = local read "SERVO ENABLE"() -> (w822:bool)
        n366 = call "Tick Count2"() -> ("Tick Count(uSec)"=w823:u32)
        n367 = Subtract(x=w823, y=w840) -> (x-y=w839:u32)
        n368 = call "Wait4"("Count(mSec)"="Servo Comm\nLoop Time (ms)") -> ()  [unwired: 1 out]
        n369 = Divide(x=w839, y=u32 1000) -> (x/y=→"dT - Comm Loop":dbl)
        n370 = case shown="True" w822 {
          tunnel: w835 -> [_ w849]
          tunnel: w834 -> [_ w880]
          tunnel: w833 -> [w843 w844]
          tunnel: w832 -> [w842 w873]
          tunnel: [w843 w846] -> w830
          tunnel: [w842 w845] -> w829
          tunnel: w828 -> [_ w852]
          tunnel: w827 -> [_ w851]
          tunnel: w826 -> [_ w850]
          tunnel: w825 -> [_ w848]
          tunnel: [u16 100 w847] -> w824
          frame False {
            # "Restart at same value\nUsed to Periodically update \nCompliance Slope"
          }
          frame True {
            n371 = flat-sequence {
              tunnel: [w886] -> w884
              tunnel: [w887] -> w883
              tunnel: [w885] -> w882
              tunnel: w880 -> [w888]
              tunnel: [w890] -> w871
              tunnel: [w889] -> w869
              tunnel: w844 -> [w890]
              tunnel: w873 -> [w889]
              tunnel: w852 -> [w885]
              tunnel: w884 -> [w908]
              tunnel: w883 -> [w909]
              tunnel: w882 -> [w907]
              tunnel: [w907] -> w881
              tunnel: [w906] -> w874
              tunnel: [w905] -> w872
              tunnel: w871 -> [w905]
              tunnel: [w904] -> w870
              tunnel: w869 -> [w904]
              tunnel: w881 -> [w930]
              tunnel: w849 -> [w929]
              tunnel: w874 -> [w924]
              tunnel: w872 -> [w926]
              tunnel: w870 -> [w925]
              tunnel: [w926] -> w867
              tunnel: [w925] -> w865
              tunnel: [w963] -> w868
              tunnel: w867 -> [w963]
              tunnel: [w962] -> w866
              tunnel: w865 -> [w962]
              tunnel: ["Servo Comm\nWait Time - (ms)"] -> w857
              tunnel: w880 -> [w970]
              tunnel: [w969] -> w879
              tunnel: [w968] -> w878
              tunnel: [w964] -> w876
              tunnel: w868 -> [w967]
              tunnel: w866 -> [w966]
              tunnel: [w967] -> w864
              tunnel: [w966] -> w861
              tunnel: [w965] -> w858
              tunnel: w857 -> [w965]
              tunnel: w851 -> [w964]
              tunnel: w879 -> [w990]
              tunnel: w878 -> [w989]
              tunnel: [w988] -> w877
              tunnel: w876 -> [w988]
              tunnel: [w987] -> w875
              tunnel: w864 -> [w986]
              tunnel: [w986] -> w863
              tunnel: [w985] -> w862
              tunnel: w861 -> [w985]
              tunnel: w858 -> [w984]
              tunnel: [w984] -> w856
              tunnel: w877 -> [w1012]
              tunnel: w875 -> [w1010]
              tunnel: w849 -> [w1011]
              tunnel: w863 -> [w1009]
              tunnel: w862 -> [w1008]
              tunnel: [w1009] -> w860
              tunnel: [w1008] -> w859
              tunnel: w856 -> [w1005]
              tunnel: [w1005] -> w855
              tunnel: w860 -> [w1045]
              tunnel: w859 -> [w1044]
              tunnel: w855 -> [w1043]
              tunnel: [w1045] -> w854
              tunnel: [w1044] -> w853
              tunnel: w854 -> [w1049]
              tunnel: w853 -> [w1048]
              tunnel: w852 -> [w1054]
              tunnel: w851 -> [w1053]
              tunnel: w850 -> [w1052]
              tunnel: w848 -> [w1047]
              tunnel: w849 -> [w1051]
              tunnel: [w1050] -> w847
              tunnel: [w1049] -> w846
              tunnel: [w1048] -> w845
              frame #0 {
                n372 = while {
                  tunnel: [w903] -> w886
                  tunnel: w885 -> [w902]
                  tunnel: [w895] -> w887
                  tunnel: w888 -> [w893]
                  tunnel: w890 -> [w892]
                  tunnel: w889 -> [w891]
                  i -> [w894]
                  stop <- w896 stop-if-true
                  # "Attemp to Read Until\nMax Read Tx Attemps Limit"
                  n373 = call "ReadServo_R3.vi"("DIO Ref In"=w891, "VISA resource name out"=w892, "Servo ID"=w902) -> ("Error"=w899:u8, "Valid Checksum"=w900:bool, "Current Position"=w903:u64)  [unwired: 6 in]
                  n374 = Increment(x=w894) -> (x+1=w897:i32)
                  n375 = Equal To 0?(x=w899) -> (x = 0?=w901:bool)
                  n376 = Greater Or Equal?(x=w897, y=w893) -> (x >= y?=w898:bool)
                  n377 = And(x=w900, y=w901) -> (x .and. y?=w895:bool)
                  n378 = Or(x=w895, y=w898) -> (x .or. y?=w896:bool)
                }
              }
              frame #1 {
                # "Read Position First"
                n379 = local read "Servo Goal Position\n - Left"() -> (w906:u16)
                n380 = case shown="True" w909 {
                  tunnel: w908 -> [_ w914]
                  tunnel: w906 -> [_ w912]
                  frame False {
                  }
                  frame True {
                    # "Convert Received Position to Angle Relative to Robot"
                    # "45 DEG MOUNT OFFSET"
                    # "1024/300"
                    n381 = local write "Current L (10bit)"(w914) -> ()
                    n382 = To Word Integer(number=w914) -> (16bit integer=w918:i16)
                    n383 = To Word Integer(number=w912) -> (16bit integer=w917:i16)
                    n384 = Subtract(x=w917, y=w918) -> (x-y=w916:i16)
                    n385 = Divide(x=w914, y=3.413333333333333) -> (x/y=w922:dbl)
                    n386 = Absolute Value(x=w916) -> (abs(x)=w915:i16)
                    n387 = Subtract(x=w922, y=sgl 60.0) -> (x-y=w920:dbl)
                    n388 = Greater?(x=w915, y=u16 5) -> (0:w911:bool)
                    n389 = Add(x=w920, y=sgl 45.0) -> (x+y=w910:dbl)
                    n390 = local write "Move Servo - L"(w911) -> ()
                    n391 = local write "Servo Moving - L"(w911) -> ()
                    n392 = local write "Current Angle\n - Left (internal)"(w910) -> ()
                    n393 = shared-variable "RT myRIO Target - Overlord\\Localization_Variables_r0.lvlib\\Left Servo Angle_Current"(w910) -> ()  [unwired: 1 in, 1 out]
                  }
                }
              }
              frame #2 {
                n394 = local read "Move Servo - L"() -> (w927:bool)
                n395 = case shown="True" w927 {
                  tunnel: w930 -> [_ w945]
                  tunnel: w924 -> [_ w932]
                  tunnel: [TRUE w943] -> w928
                  tunnel: w929 -> [_ w935]
                  tunnel: w926 -> [_ w934]
                  tunnel: w925 -> [_ w933]
                  frame False {
                    # "Only Send if Current Position is far enough"
                  }
                  frame True {
                    w941 = 1
                    # "High Byte"
                    # "Low Byte"
                    n396 = Type Cast(type="", x=w932) -> (*(type *) &x=w942:string)
                    n397 = local write "Servo Moving - L"(TRUE) -> ()
                    n398 = String Subset(string=w942, offset (0)=1, length (rest)=w941) -> (substring=w937:string)
                    n399 = String Subset(string=w942, offset (0)=0, length (rest)=w941) -> (substring=w936:string)
                    n400 = while {
                      tunnel: w945 -> [w959]
                      tunnel: [w951] -> w943
                      tunnel: w937 -> [w955]
                      tunnel: w936 -> [w954]
                      tunnel: w935 -> [w948]
                      tunnel: w934 -> [w947]
                      tunnel: w933 -> [w946]
                      i -> [w949]
                      stop <- w950 stop-if-true
                      # "Attemp to Write Until\nMax Write Tx Attemps Limit"
                      n401 = call "MoveServo_R3.vi"("DIO Ref Out"=w946, "VISA resource name out"=w947, "GP - Low Byte"=w955, "GP - High Byte"=w954, "Servo ID"=w959) -> ("Valid Checksum"=w956:bool, "Error"=w958:u64)  [unwired: 5 in]
                      n402 = Equal To 0?(x=w958) -> (x = 0?=w957:bool)
                      n403 = And(x=w956, y=w957) -> (x .and. y?=w951:bool)
                      n404 = Increment(x=w949) -> (x+1=w953:i32)
                      n405 = Greater Or Equal?(x=w953, y=w948) -> (x >= y?=w952:bool)
                      n406 = Or(x=w951, y=w952) -> (x .or. y?=w950:bool)
                    }
                  }
                }
                n407 = case shown="True" w928 {
                  frame False {
                  }
                  frame True {
                    # "Update Servo flag"
                    n408 = local write "Move Servo - L"(FALSE) -> ()
                  }
                }
              }
              frame #3 {
                n409 = call "Wait2"("Count(mSec)"="Servo Comm\nWait Time - (ms)") -> ()  [unwired: 1 out]
              }
              frame #4 {
                n410 = while {
                  tunnel: [w983] -> w969
                  tunnel: w964 -> [w982]
                  tunnel: [w975] -> w968
                  tunnel: w970 -> [w973]
                  tunnel: w967 -> [w972]
                  tunnel: w966 -> [w971]
                  i -> [w974]
                  stop <- w976 stop-if-true
                  # "Attemp to Read Until\nMax Read Tx Attemps Limit"
                  n411 = call "ReadServo_R3.vi"("DIO Ref In"=w971, "VISA resource name out"=w972, "Servo ID"=w982) -> ("Error"=w979:u8, "Valid Checksum"=w980:bool, "Current Position"=w983:u64)  [unwired: 6 in]
                  n412 = Increment(x=w974) -> (x+1=w977:i32)
                  n413 = Equal To 0?(x=w979) -> (x = 0?=w981:bool)
                  n414 = Greater Or Equal?(x=w977, y=w973) -> (x >= y?=w978:bool)
                  n415 = And(x=w980, y=w981) -> (x .and. y?=w975:bool)
                  n416 = Or(x=w975, y=w978) -> (x .or. y?=w976:bool)
                }
              }
              frame #5 {
                n417 = local read "Servo Goal Position\n - Right"() -> (w987:u16)
                n418 = case shown="True" w989 {
                  tunnel: w990 -> [_ w994]
                  tunnel: w987 -> [_ w993]
                  frame False {
                    # "Don't update current position"
                  }
                  frame True {
                    # "Convert Received Position to Angle Relative to Robot"
                    # "45 DEG MOUNT OFFSET"
                    # "1024/300"
                    n419 = local write "Current R (10bit)"(w994) -> ()
                    n420 = Divide(x=w994, y=3.413333333333333) -> (x/y=w1003:dbl)
                    n421 = Subtract(x=w1003, y=sgl 60.0) -> (x-y=w1001:dbl)
                    n422 = Subtract(x=w1001, y=sgl 45.0) -> (x-y=w991:dbl)
                    n423 = To Word Integer(number=w993) -> (16bit integer=w998:i16)
                    n424 = To Word Integer(number=w994) -> (16bit integer=w999:i16)
                    n425 = shared-variable "RT myRIO Target - Overlord\\Localization_Variables_r0.lvlib\\Right Servo Angle_Current"(w991) -> ()  [unwired: 1 in, 1 out]
                    n426 = local write "Current Angle\n - Right (internal)"(w991) -> ()
                    n427 = Subtract(x=w998, y=w999) -> (x-y=w997:i16)
                    n428 = Absolute Value(x=w997) -> (abs(x)=w996:i16)
                    n429 = Greater?(x=w996, y=u16 5) -> (0:w992:bool)
                    n430 = local write "Move Servo - R"(w992) -> ()
                    n431 = local write "Servo Moving - R"(w992) -> ()
                  }
                }
              }
              frame #6 {
                n432 = local read "Move Servo - R"() -> (w1006:bool)
                n433 = case shown="True" w1006 {
                  tunnel: w1010 -> [_ w1015]
                  tunnel: w1012 -> [_ w1022]
                  tunnel: [TRUE w1023] -> w1007
                  tunnel: w1011 -> [_ w1018]
                  tunnel: w1009 -> [_ w1017]
                  tunnel: w1008 -> [_ w1016]
                  frame False {
                  }
                  frame True {
                    w1025 = 1
                    # "High Byte"
                    # "Low Byte"
                    n434 = Type Cast(type="", x=w1015) -> (*(type *) &x=w1024:string)
                    n435 = local write "Servo Moving - R"(TRUE) -> ()
                    n436 = String Subset(string=w1024, offset (0)=1, length (rest)=w1025) -> (substring=w1021:string)
                    n437 = String Subset(string=w1024, offset (0)=0, length (rest)=w1025) -> (substring=w1020:string)
                    n438 = while {
                      tunnel: [w1034] -> w1023
                      tunnel: w1022 -> [w1039]
                      tunnel: w1021 -> [w1038]
                      tunnel: w1020 -> [w1037]
                      tunnel: w1018 -> [w1032]
                      tunnel: w1017 -> [w1030]
                      tunnel: w1016 -> [w1029]
                      i -> [w1033]
                      stop <- w1031 stop-if-true
                      # "Attemp to Write Until\nMax Write Tx Attemps Limit"
                      n439 = call "MoveServo_R3.vi"("DIO Ref Out"=w1029, "VISA resource name out"=w1030, "GP - Low Byte"=w1038, "GP - High Byte"=w1037, "Servo ID"=w1039) -> ("Valid Checksum"=w1041:bool, "Error"=w1040:u64)  [unwired: 5 in]
                      n440 = Increment(x=w1033) -> (x+1=w1035:i32)
                      n441 = Greater Or Equal?(x=w1035, y=w1032) -> (x >= y?=w1036:bool)
                      n442 = Equal To 0?(x=w1040) -> (x = 0?=w1042:bool)
                      n443 = And(x=w1041, y=w1042) -> (x .and. y?=w1034:bool)
                      n444 = Or(x=w1034, y=w1036) -> (x .or. y?=w1031:bool)
                    }
                  }
                }
                n445 = case shown="True" w1007 {
                  frame False {
                  }
                  frame True {
                    # "Update Servo flag"
                    n446 = local write "Move Servo - R"(FALSE) -> ()
                  }
                }
              }
              frame #7 {
                n447 = call "Wait3"("Count(mSec)"=w1043) -> ()  [unwired: 1 out]
              }
              frame #8 {
                # "Increment Service Count"
                # "Update Compliance Slope\nEvery x loops"
                n448 = Equal?(x=w1047, y=u16 1000) -> (x = y?=w1056:bool)
                n449 = case shown="True" w1056 {
                  tunnel: w1052 -> [_ w1066]
                  tunnel: w1049 -> [_ w1065]
                  tunnel: w1048 -> [_ w1064]
                  tunnel: w1049 -> [_ w1063]
                  tunnel: w1048 -> [_ w1062]
                  tunnel: w1054 -> [_ w1061]
                  tunnel: w1053 -> [_ w1060]
                  tunnel: w1047 -> [w1057 _]
                  tunnel: [w1057 u16 0] -> w1055
                  tunnel: w1051 -> [_ w1058]
                  frame False {
                  }
                  frame True {
                    # "Reset Service\nCount"
                    n450 = flat-sequence {
                      tunnel: w1065 -> [w1071]
                      tunnel: w1064 -> [w1070]
                      tunnel: w1061 -> [w1072]
                      tunnel: [w1068] -> w1067
                      tunnel: w1066 -> [w1069]
                      tunnel: w1058 -> [w1068]
                      tunnel: w1060 -> [w1084]
                      tunnel: w1067 -> [w1083]
                      tunnel: w1066 -> [w1082]
                      tunnel: w1063 -> [w1081]
                      tunnel: w1062 -> [w1080]
                      frame #0 {
                        n451 = while {
                          tunnel: w1068 -> [w1079]
                          tunnel: w1071 -> [w1077]
                          tunnel: w1070 -> [w1076]
                          tunnel: w1072 -> [w1075]
                          tunnel: w1069 -> [w1074]
                          i -> [w1073]
                          stop <- w1078 stop-if-true
                          n452 = call "Set_Compliance_Slope_R2.vi"("Compliance Slope"=w1074, "DIO Ref Out"=w1076, "VISA resource name"=w1077, "Servo ID"=w1075) -> ()  [unwired: 6 in, 2 out]
                          n453 = Greater Or Equal?(x=w1073, y=w1079) -> (x >= y?=w1078:bool)
                        }
                      }
                      frame #1 {
                        n454 = while {
                          tunnel: w1083 -> [w1091]
                          tunnel: w1084 -> [w1089]
                          tunnel: w1081 -> [w1088]
                          tunnel: w1080 -> [w1087]
                          tunnel: w1082 -> [w1086]
                          i -> [w1085]
                          stop <- w1090 stop-if-true
                          n455 = call "Set_Compliance_Slope_R2.vi"("Compliance Slope"=w1086, "DIO Ref Out"=w1087, "VISA resource name"=w1088, "Servo ID"=w1089) -> ()  [unwired: 6 in, 2 out]
                          n456 = Greater Or Equal?(x=w1085, y=w1091) -> (x >= y?=w1090:bool)
                        }
                      }
                    }
                  }
                }
                n457 = Increment(x=w1055) -> (x+1=w1050:u16)
              }
            }
          }
        }
      }
    }
    frame #2 {
      n458 = VISA Close(VISA resource name=w1093) -> ()  [unwired: 1 in, 1 out]
      n459 = call <vilib>:"Close.vi"("DIO Ref In"=w1092) -> ()  [unwired: 10 in, 1 out]
    }
  }
  n460 = while {
    stop <- FALSE stop-if-true
    n461 = call "Wait9"("Count(mSec)"=u32 1000) -> ()  [unwired: 1 out]
  }
  n462 = while {
    shift-right: [w1154] -> _
    shift-left: "Initial Main State - Left" -> [w1179]
    shift-right: [w1146] -> _
    shift-left: "Search Direction - in - L" -> [w1173]
    shift-right: [w1145] -> _
    shift-left: FALSE -> [w1172]
    shift-right: [w1148] -> _
    shift-left: w13 -> [w1147]
    shift-right: [w1149] -> _
    shift-left: w13 -> [w1166]
    shift-right: [w1150] -> _
    shift-left: w13 -> [w1171]
    shift-right: [w1151] -> _
    shift-left: w13 -> [w1165]
    shift-right: [w1152] -> _
    shift-left: w13 -> [w1164]
    shift-right: [w1097] -> _
    shift-left: "Search Direction - in - Right" -> [w1121]
    shift-right: [w1142] -> _
    shift-left: FALSE -> [w1119]
    shift-right: [w1143] -> _
    shift-left: w12 -> [w1110]
    shift-right: [w1098] -> _
    shift-left: w12 -> [w1109]
    shift-right: [w1099] -> _
    shift-left: w12 -> [w1116]
    shift-right: [w1100] -> _
    shift-left: w12 -> [w1118]
    shift-right: [w1101] -> _
    shift-left: w12 -> [w1117]
    shift-right: [w1108] -> _
    shift-left: "Initial Main State- Right" -> [w1133]
    shift-right: [w1138] -> _
    shift-left: 0 -> [w1140]
    shift-right: [w1105] -> _
    shift-left: 0 -> [w1125]
    shift-right: [w1137] -> _
    shift-left: "Initial Tracking State - Left" -> [w1139]
    shift-right: [w1103] -> _
    shift-left: "Initial Tracking State - Right" -> [w1131]
    shift-right: [w1104] -> _
    shift-left: "Initial Recovery State  - Right" -> [w1132]
    shift-right: [w1135] -> _
    shift-left: "Initial Recovery State - L" -> [w1136]
    stop <- FALSE stop-if-true
    w1158 = T2."Tracking" ("Next Main State")
    # "Wait for New"
    # "ADD TRACKING TIMEOUT COUNT**********************"
    # "Service Track Angle Flag"
    # "Add Logic to Have Search Directions\nopposite if Both Searching"
    # "REMOVE LAST GOAL POSITION WITH cURRENT"
    # "Go to Current State"
    # "Add Logic to Have Search Directions\nopposite if Both Searching"
    # "Manuallly Reset\nRespond Var"
    # "Manuallly Reset\nRespond Var"
    # "Update Comm Process Variables"
    # "Both Tracking"
    # "Current delta - L"
    # "delta move sum - R"
    # "delta move sum - L"
    # "Current delta - R"
    # "Service Move Respond Variables"
    n463 = local read "Min Num Frames\nper Search"() -> (w1144:i32)
    n464 = local read "Minimum Delta \nServo Threshold"() -> (w1163:i16)
    n465 = local read "Maximum Move \nServo Threshold"() -> (w1162:i16)
    n466 = local read "Middle Beacon\nCoordinates"() -> (w1111:cluster{"X":sgl, "Y":sgl})
    n467 = local read "Position \nLock Status"() -> (w1170:bool)
    n468 = local read "Position \nLock Status"() -> (w1114:bool)
    n469 = local read "Search Step Size"() -> (w1161:u16)
    n470 = local read "Last Orientation"() -> (w1168:sgl)
    n471 = local read "Last Orientation"() -> (w1112:sgl)
    n472 = local read "Last Position"() -> (w1169:cluster{"X":sgl, "Y":sgl})
    n473 = local read "Last Position"() -> (w1113:cluster{"X":sgl, "Y":sgl})
    n474 = local read "Min Num Frames\nper Search"() -> (w1115:i32)
    n475 = call "Wait"("Count(mSec)"="Servo Algorithm\nCycle Time(ms)") -> ()  [unwired: 1 out]
    n476 = local read "Minimum Delta \nServo Threshold"() -> (w1123:i16)
    n477 = local read "Maximum Move \nServo Threshold"() -> (w1122:i16)
    n478 = local read "Search Step Size"() -> (w1120:u16)
    n479 = local read "New Data  Flag\nRight Servo"() -> (w1128:bool)
    n480 = local read "New Data  Flag\nLeft Servo"() -> (w1134:bool)
    n481 = local read "Image Lock - Right"() -> (w1130:bool)
    n482 = local read "Image Lock - Left"() -> (w1178:bool)
    n483 = local read "Tracking Angle - Right"() -> (w1127:sgl)
    n484 = local read "Tracking Angle - Left"() -> (w1176:sgl)
    n485 = local read "Current R (10bit)"() -> (w1126:u16)
    n486 = local read "Current L (10bit)"() -> (w1175:u16)
    n487 = case shown="True" w1128 {
      tunnel: [w1206 w1244] -> w1096
      tunnel: [w1200 w1243] -> w1107
      tunnel: w1133 -> [w1201 w1242]
      tunnel: w1130 -> [_ w1241]
      tunnel: "Track Angle Valid  - Right" -> [_ w1240]
      tunnel: w1127 -> [_ w1239]
      tunnel: w1126 -> [w1206 w1238]
      tunnel: "Mounting Offset - Right" -> [_ w1237]
      tunnel: w1121 -> [w1197 w1236]
      tunnel: w1119 -> [_ w1235]
      tunnel: w1116 -> [w1198 w1234]
      tunnel: w1114 -> [_ w1233]
      tunnel: w1113 -> [_ w1232]
      tunnel: w1112 -> [_ w1231]
      tunnel: w1111 -> [_ w1230]
      tunnel: w1109 -> [w1196 w1229]
      tunnel: w1118 -> [w1195 w1228]
      tunnel: w1117 -> [w1199 w1227]
      tunnel: w1123 -> [_ w1226]
      tunnel: w1122 -> [_ w1225]
      tunnel: w1120 -> [_ w1224]
      tunnel: [0 w1223] -> w1106
      tunnel: [w1201 w1222] -> w1108
      tunnel: [w1200 w1221] -> w1102
      tunnel: [w1199 w1220] -> w1101
      tunnel: [w1195 w1219] -> w1100
      tunnel: [w1198 w1218] -> w1099
      tunnel: [w1196 w1217] -> w1098
      tunnel: w1110 -> [_ w1216]
      tunnel: [w1197 w1215] -> w1097
      tunnel: w1115 -> [_ w1214]
      tunnel: w1125 -> [w1204 w1213]
      tunnel: w1131 -> [w1203 w1212]
      tunnel: [w1204 w1211] -> w1105
      tunnel: [w1203 w1210] -> w1103
      tunnel: w1132 -> [w1202 w1209]
      tunnel: [w1202 w1208] -> w1104
      frame False {
        w1200 = FALSE
        # "Recovery Mode COunt"
        # "Frames Processed - L"
        # "Recovery Search move Count - L"
        # "Recovery Search Attempt Count- L"
        # "WAITING FOR NEW IMAGE, RETAIN ALL VALUES"
      }
      frame True {
        w1246 = u16 1023
        w1249 = u16 0
        # "New Tracking State"
        # "Tracking Timeout Count"
        # "Next Main State"
        # "Next Recovery State"
        # "Reset Respond"
        # "Search Direction"
        # "Recovery Count"
        # "Recovery Search move Count"
        # "Recovery Search Attempt Count"
        # "Frames Processed"
        # "Apply Floor/Ceiling to Goal Position"
        # "Current move Delta"
        # "Service Track Angle Flag"
        # "Move Servo"
        # "Goal Position"
        # "Go to Current State"
        n488 = case shown="\"Recovery Mode\"" w1242 {
          tunnel: w1238 -> [w1268 w1345 w1523]
          tunnel: w1239 -> [_ w1347 _]
          tunnel: w1224 -> [w1267 _ w1518]
          tunnel: w1236 -> [w1266 w1327 w1512]
          tunnel: [w1265 w1343 w1522] -> w1250
          tunnel: [w1263 w1344 w1521] -> w1243
          tunnel: w1240 -> [w1261 w1338 w1499]
          tunnel: [w1260 w1340 w1508] -> w1222
          tunnel: w1241 -> [w1259 w1339 w1498]
          tunnel: w1237 -> [_ w1348 w1519]
          tunnel: w1226 -> [_ w1346 _]
          tunnel: [w1253 w1342 w1503] -> w1223
          tunnel: w1225 -> [_ w1341 _]
          tunnel: w1234 -> [w1258 _ w1513]
          tunnel: [enum16{"Generic Sweep", "Recovery Search"}."Recovery Search" enum16{"Generic Sweep", "Recovery Search"}."Recovery Search" w1520] -> w1208
          tunnel: w1229 -> [_ _ w1517]
          tunnel: w1209 -> [_ _ w1500]
          tunnel: w1235 -> [_ w1324 w1529]
          tunnel: w1216 -> [_ w1329 w1524]
          tunnel: w1231 -> [_ w1331 w1526]
          tunnel: w1232 -> [_ w1332 w1527]
          tunnel: w1233 -> [_ w1333 w1528]
          tunnel: w1230 -> [_ w1330 w1525]
          tunnel: [FALSE w1326 w1501] -> w1221
          tunnel: w1214 -> [w1257 _ w1511]
          tunnel: [w1253 w1321 w1510] -> w1217
          tunnel: [w1253 w1321 w1516] -> w1220
          tunnel: [w1253 w1321 w1515] -> w1219
          tunnel: [w1256 w1322 w1514] -> w1218
          tunnel: w1228 -> [_ _ w1506]
          tunnel: w1227 -> [_ _ w1505]
          tunnel: [w1254 w1327 w1504] -> w1215
          tunnel: w1213 -> [_ w1337 _]
          tunnel: [w1253 w1328 w1503] -> w1211
          tunnel: w1212 -> [_ w1334 _]
          tunnel: [enum16{"Track", "Reactive Predict", ""}."Track" ("Initial Tracking State - Right") w1325 enum16{"Track", "Reactive Predict", ""}."Track" ("Initial Tracking State - Right")] -> w1210
          frame "Start Up Search", Default {
            w1253 = u16 0
            # "Search Direction"
            # "Wait for 'x' Images to be Processed\nBefore Going to Next Step"
            # "Next Main State"
            # "New Goal Position"
            # "Move Servo"
            # "Choose Next State"
            # "Frames Processed Count"
            n489 = Greater Or Equal?(x=w1258, y=w1257) -> (x >= y?=w1264:bool)
            n490 = case shown="True" w1264 {
              tunnel: w1268 -> [w1283 w1295]
              tunnel: w1267 -> [_ w1293]
              tunnel: w1266 -> [w1282 w1292]
              tunnel: [w1283 w1289] -> w1265
              tunnel: [w1281 0] -> w1256
              tunnel: [FALSE TRUE] -> w1262
              tunnel: w1258 -> [w1284 _]
              tunnel: [w1282 w1286] -> w1254
              frame False {
                # "Increase Frames\nProcessed Count"
                n491 = Increment(x=w1284) -> (x+1=w1281:i32)
              }
              frame True {
                # "Reset Frames\nProcessed Count"
                # "SWEEP SEARCH - Startup"
                # "Multiple New Step\nby Step SIze"
                # "F = CCW\nT = CW"
                # "Last Direction"
                # "Min Step"
                # "add 10 in case\nactual position\nis lower than GP"
                # "Set New Step #"
                # "Choose Direction"
                # "Nearest step"
                # "Adjust Actual Posiiton\n to pre-determiend steps"
                # "Move Servo 1 \"Step\" to\nSearch"
                n492 = Add(x=3, y=w1295) -> (x+y=w1301:i32)
                n493 = Quotient & Remainder(x=w1301, y=w1293) -> (floor(x/y)=w1299:i32)  [unwired: 1 out]
                n494 = To Byte Integer(number=w1299) -> (8bit integer=w1290:i8)
                n495 = Less?(x=w1290, y=1) -> (x < y?=w1296:bool)
                n496 = case shown="False" w1296 {
                  tunnel: w1290 -> [w1312 w1320]
                  tunnel: [w1314 FALSE] -> w1286
                  tunnel: [w1313 w1320] -> w1298
                  tunnel: w1292 -> [w1311 _]
                  tunnel: w1293 -> [w1309 _]
                  frame False {
                    # "Max Step"
                    # "# of steps\nminus 1"
                    n497 = Divide(x=1024, y=w1309) -> (x/y=w1306:dbl)
                    n498 = To Unsigned Byte Integer(number=w1306) -> (unsigned 8bit integer=w1307:u8)
                    n499 = Greater Or Equal?(x=w1312, y=w1307) -> (x >= y?=w1308:bool)
                    n500 = case shown="True" w1308 {
                      tunnel: [w1315 TRUE] -> w1314
                      tunnel: [w1316 w1317] -> w1313
                      tunnel: w1312 -> [w1316 w1317]
                      tunnel: w1311 -> [w1315 _]
                      frame False {
                        # "No Need to\nChange Direction"
                      }
                      frame True {
                        # "T"
                        # "Move CW"
                      }
                    }
                  }
                  frame True {
                    # "F"
                    # "Move CCW"
                  }
                }
                n501 = case shown="False" w1286 {
                  tunnel: w1298 -> [w1303 w1304]
                  tunnel: [w1302 w1305] -> w1294
                  frame False {
                    # "CCW\n+1"
                    n502 = Increment(x=w1303) -> (x+1=w1302:i8)
                  }
                  frame True {
                    # "CW\n-1"
                    n503 = Decrement(x=w1304) -> (x-1=w1305:i8)
                  }
                }
                n504 = Multiply(x=w1294, y=w1293) -> (x*y=w1291:u16)
                n505 = To Unsigned Word Integer(number=w1291) -> (unsigned 16bit integer=w1289:u16)
              }
            }
            n506 = case shown="False" w1261 {
              tunnel: [w1272 FALSE] -> w1263
              tunnel: w1262 -> [w1272 _]
              tunnel: [w1273 w1278] -> w1260
              tunnel: w1259 -> [_ w1276]
              frame False {
                # "Check other Servo\nStay in Startup  State"
                n507 = local read "Track Angle Valid - Left"() -> (w1269:bool)
                n508 = local read "Image Lock - Left"() -> (w1270:bool)
                n509 = Or(x=w1269, y=w1270) -> (x .or. y?=w1271:bool)
                n510 = case shown="True" w1271 {
                  tunnel: [T2."Start Up Search" ("Next Main State") T2."Recovery Mode" ("Next Main State")] -> w1273
                  frame False {
                  }
                  frame True {
                  }
                }
              }
              frame True {
                # "Override Move Servo\nCommand bc an Angle Was Found\nduring this Step"
                # "Transition to Tracking State When\nImage Processing has Locked"
                n511 = case shown="False" w1276 {
                  tunnel: [T2."Start Up Search" ("Next Main State") T2."Tracking" ("Next Main State")] -> w1278
                  frame False {
                  }
                  frame True {
                  }
                }
              }
            }
          }
          frame "Tracking" {
            w1321 = 0
            # "Frames Processed Count"
            # "Image Lock - L"
            # "Track Angle Valid"
            # "Tracking Angle"
            # "Tracking Timeout Count"
            # "Max ove delta"
            # "Move delta threshold"
            # "mount offset"
            # "Current Position"
            # "Move Respond"
            # "Trackin Timeout count"
            # "Move Servo"
            # "delta"
            # "GP"
            # "Reset Move Respond"
            # "New Tracking State"
            # "Delta Move Sum"
            # "Choose Next State"
            n512 = case shown="\"Reactive Predict\"" w1334 {
              tunnel: w1348 -> [w1366 _]
              tunnel: w1347 -> [w1365 _]
              tunnel: w1346 -> [w1364 _]
              tunnel: w1345 -> [w1363 w1421]
              tunnel: [w1362 w1419] -> w1344
              tunnel: [w1361 w1427] -> w1343
              tunnel: [w1360 0] -> w1342
              tunnel: w1341 -> [w1359 _]
              tunnel: w1339 -> [w1358 w1411]
              tunnel: w1338 -> [w1357 w1414]
              tunnel: w1337 -> [w1356 w1416]
              tunnel: w1333 -> [_ w1426]
              tunnel: w1332 -> [_ w1425]
              tunnel: w1331 -> [_ w1424]
              tunnel: w1330 -> [_ w1423]
              tunnel: w1324 -> [_ w1422]
              tunnel: w1329 -> [_ w1420]
              tunnel: [TRUE w1417] -> w1326
              tunnel: [w1353 w1415] -> w1328
              tunnel: [w1351 w1413] -> w1325
              tunnel: [0 0] -> w1322
              frame "Track", Default {
                # "Reset"
                # "Tracking Timeout"
                # "Move Delta"
                # "Goal Position"
                # "Tracking Move"
                # "Move Servo"
                # "Only Consider Tracking Angle\n\nIF\n\nImage Locked        == T\nTrack Angle Flag   == T"
                n513 = And(x=w1358, y=w1357) -> (x .and. y?=w1350:bool)
                n514 = case shown="True" w1350 {
                  tunnel: w1366 -> [_ w1372]
                  tunnel: w1365 -> [_ w1390]
                  tunnel: w1364 -> [_ w1387]
                  tunnel: w1363 -> [w1369 w1377]
                  tunnel: [w1369 w1386] -> w1361
                  tunnel: [w1371 w1385] -> w1362
                  tunnel: [w1371 w1384] -> _
                  tunnel: [u16 0 w1383] -> w1360
                  tunnel: w1359 -> [_ w1379]
                  tunnel: w1356 -> [w1368 _]
                  tunnel: [w1367 0] -> w1353
                  frame False {
                    w1371 = FALSE
                    # "Increment timeout"
                    n515 = Increment(x=w1368) -> (x+1=w1367:i32)
                  }
                  frame True {
                    # "Convert Track Angle to UINT16"
                    # "1024/300"
                    # "Move to Tracking Angle \n\nif delta is greater than move servo threshold\nAND less than max move threshold"
                    n516 = Add(x=w1390, y=w1372) -> (x+y=w1393:sgl)
                    n517 = Add(x=w1393, y=sgl 60.0) -> (x+y=w1392:sgl)
                    n518 = Multiply(x=3.413333333333333, y=w1392) -> (x*y=w1373:dbl)
                    n519 = To Word Integer(number=w1377) -> (16bit integer=w1375:i16)
                    n520 = To Unsigned Word Integer(number=w1373) -> (unsigned 16bit integer=w1389:u16)
                    n521 = To Word Integer(number=w1373) -> (16bit integer=w1388:i16)
                    n522 = Subtract(x=w1388, y=w1375) -> (x-y=w1378:i16)
                    n523 = Absolute Value(x=w1378) -> (abs(x)=w1374:i16)
                    n524 = Greater Or Equal?(x=w1374, y=w1387) -> (x >= y?=w1381:bool)
                    n525 = Less Or Equal?(x=w1374, y=w1379) -> (x <= y?=w1380:bool)
                    n526 = And(x=w1381, y=w1380) -> (x .and. y?=w1382:bool)
                    n527 = case shown="True" w1382 {
                      tunnel: w1389 -> [_ w1401]
                      tunnel: [w1396 w1401] -> w1386
                      tunnel: [w1397 w1407] -> w1385
                      tunnel: [w1397 w1407] -> w1384
                      tunnel: w1377 -> [w1396 _]
                      tunnel: w1374 -> [_ w1406]
                      tunnel: [u16 0 w1406] -> w1383
                      tunnel: w1372 -> [_ w1400]
                      frame False {
                        w1397 = FALSE
                        # "Don't Move"
                      }
                      frame True {
                        w1407 = TRUE
                        # "45 DEG MOUNT OFFSET"
                        # "1024/300"
                        # "Current Delta"
                        # "Use new Track Angle"
                        n528 = Divide(x=w1401, y=3.413333333333333) -> (x/y=w1403:dbl)
                        n529 = Negate(x=w1400) -> (-x=w1399:sgl)
                        n530 = Subtract(x=w1403, y=sgl 60.0) -> (x-y=w1405:dbl)
                        n531 = Add(x=w1405, y=w1399) -> (x+y=w1398:dbl)
                        n532 = local write "Last Track Angle - R"(w1398) -> ()
                      }
                    }
                  }
                }
                n533 = local read "Timeout to \nEnable Reactive Predict"() -> (w1354:u16)
                n534 = Less?(x=w1353, y=w1354) -> (x < y?=w1352:bool)
                n535 = case shown="False" w1352 {
                  tunnel: [enum16{"Track", "Reactive Predict", ""}."Reactive Predict" ("Initial Tracking State - Right") enum16{"Track", "Reactive Predict", ""}."Track" ("Initial Tracking State - Right")] -> w1351
                  frame False {
                  }
                  frame True {
                  }
                }
              }
              frame "Reactive Predict" {
                # "Choose New\nTracking State"
                n536 = Or(x=w1411, y=w1414) -> (x .or. y?=w1410:bool)
                n537 = case shown="False" w1410 {
                  tunnel: [w1440 w1492] -> w1427
                  tunnel: w1426 -> [w1439 _]
                  tunnel: w1425 -> [w1438 _]
                  tunnel: w1424 -> [w1437 _]
                  tunnel: w1423 -> [w1436 _]
                  tunnel: w1422 -> [w1435 _]
                  tunnel: w1420 -> [w1434 _]
                  tunnel: [w1433 w1491] -> w1419
                  tunnel: [w1432 w1491] -> w1417
                  tunnel: w1416 -> [w1431 _]
                  tunnel: [w1430 0] -> w1415
                  tunnel: [enum16{"Track", "Reactive Predict", ""}."Reactive Predict" ("Initial Tracking State - Right") enum16{"Track", "Reactive Predict", ""}."Track" ("Initial Tracking State - Right")] -> w1413
                  tunnel: w1421 -> [w1428 w1492]
                  frame False {
                    # "Stay in Reactive State"
                    # "Increment Track Timeout"
                    # "Move Respond Flag"
                    n538 = Increment(x=w1431) -> (x+1=w1430:i32)
                    n539 = case shown="True" w1435 {
                      tunnel: w1439 -> [_ w1455]
                      tunnel: w1438 -> [_ w1454]
                      tunnel: w1437 -> [_ w1453]
                      tunnel: w1436 -> [_ w1452]
                      tunnel: w1434 -> [_ w1449]
                      tunnel: [w1441 w1445] -> w1440
                      tunnel: [w1442 w1444] -> w1433
                      tunnel: [w1442 w1444] -> w1432
                      tunnel: w1428 -> [w1441 w1443]
                      frame False {
                        w1442 = FALSE
                        # "Reset Move Respond = F"
                        # "Move Servo = F"
                      }
                      frame True {
                        w1444 = TRUE
                        # "Position Lock"
                        # "Current Servo\nPosition"
                        # "Reset Move\nRespond = T"
                        # "Move Servo = T"
                        # "Apply Direction \nto Offset (delta sum)"
                        # "Check Last Known Position of Robot"
                        n540 = case shown="True" w1455 {
                          tunnel: w1454 -> [_ w1483]
                          tunnel: w1453 -> [_ w1458]
                          tunnel: w1452 -> [_ w1459]
                          tunnel: [sgl 1.0 ("y") w1457] -> w1451
                          frame False {
                            # "No Position Data Available"
                            # "Default is to move\nSame Direction as other\nServo"
                          }
                          frame True {
                            w1464 = sgl 1.0 ("y")
                            # "Use previous position/orientation to Guess Which Direction to Move Servo"
                            # "Choose Search Direction"
                            # "\"Perpendicular \nThreshold\""
                            # "If Orientation is\n ~Perpendicular -> Start Search\n in Opposite Direction of Other"
                            # "****add 90 until orientation angle is fixed"
                            # "Last Orientation"
                            # "Convert to Rad"
                            # "Avoid Divide by 0"
                            # "-1/m"
                            # "Calculate Normal Line to \nLast Robot Position\nfrom Center Beacon"
                            # "last Position \nCoordinates"
                            n541 = Unbundle(w1483) -> ("X"=w1463:sgl, "Y"=w1462:sgl)
                            n542 = Unbundle(w1459) -> ("X"=w1461:sgl, "Y"=w1460:sgl)
                            n543 = Subtract(x=w1462, y=w1460) -> (x-y=w1479:sgl)
                            n544 = Subtract(x=w1463, y=w1461) -> (x-y=w1477:sgl)
                            n545 = Equal To 0?(x=w1477) -> (x = 0?=w1478:bool)
                            n546 = case shown="False" w1478 {
                              tunnel: w1479 -> [w1486 _]
                              tunnel: w1477 -> [w1485 _]
                              tunnel: [w1484 1000000000000000.0] -> w1476
                              frame False {
                                n547 = Divide(x=w1486, y=w1485) -> (x/y=w1484:sgl)
                              }
                              frame True {
                              }
                            }
                            n548 = Equal To 0?(x=w1476) -> (x = 0?=w1481:bool)
                            n549 = case shown="False" w1481 {
                              tunnel: [w1488 1e-08] -> w1480
                              tunnel: w1476 -> [w1488 _]
                              frame False {
                              }
                              frame True {
                                # "Can't have infinit slope"
                              }
                            }
                            n550 = Divide(x=-1.0, y=w1480) -> (x/y=w1475:dbl)
                            n551 = Inverse Tangent(1:w1475) -> (0:w1473:dbl)
                            n552 = expression code="(x/pi)*180.0" "radians to degrees"(w1473) -> (w1474:dbl)
                            n553 = To Single Precision Float(number=w1474) -> (single precision float=w1471:sgl)
                            n554 = Add(x=w1458, y=sgl 90.0) -> (x+y=w1470:sgl)
                            n555 = Subtract(x=w1471, y=w1470) -> (x-y=w1469:sgl)
                            n556 = Absolute Value(x=w1469) -> (abs(x)=w1468:sgl)
                            n557 = Less Or Equal?(x=w1468, y=sgl 10.0) -> (x <= y?=w1466:bool)
                            n558 = Negate(x=w1464) -> (-x=w1465:sgl)
                            n559 = Select(t=w1465, s=w1466, f=w1464) -> (s? t:f=w1457:sgl)
                          }
                        }
                        n560 = To Word Integer(number=w1451) -> (16bit integer=w1450:i16)
                        n561 = Multiply(x=w1450, y=w1449) -> (x*y=w1448:i32)
                        n562 = To Word Integer(number=w1443) -> (16bit integer=w1447:i16)
                        n563 = Add(x=w1448, y=w1447) -> (x+y=w1446:i32)
                        n564 = To Unsigned Word Integer(number=w1446) -> (unsigned 16bit integer=w1445:u16)
                      }
                    }
                  }
                  frame True {
                    w1491 = TRUE
                    # "Go Directly to Track State"
                  }
                }
              }
            }
            n565 = local read "Tracking Timeout\nThreshold"() -> (w1335:i32)
            n566 = Less?(x=w1328, y=w1335) -> (x < y?=w1336:bool)
            n567 = case shown="False" w1336 {
              tunnel: [T2."Recovery Mode" ("Next Main State") T2."Tracking" ("Next Main State")] -> w1340
              frame False {
              }
              frame True {
              }
            }
          }
          frame "Recovery Mode" {
            w1503 = u16 0
            # "Increment Recovery Mode Count"
            # "Recovvery Mode\nCount"
            # "Frames Processed"
            # "Choose Next Main State"
            # "Reset recovery count"
            # "Recovery move\nCount"
            # "Recovery Search\nAttempt count"
            # "Move Servo = T"
            # "delta move sum"
            # "Robot Position Valid"
            n568 = local read "Image Lock - Left"() -> (w1507:bool)
            n569 = Or(x=w1498, y=w1499) -> (x .or. y?=w1497:bool)
            n570 = case shown="\"Recovery Search\"" w1500 {
              tunnel: w1529 -> [_ _]
              tunnel: w1528 -> [_ _]
              tunnel: w1527 -> [_ _]
              tunnel: w1526 -> [_ _]
              tunnel: w1525 -> [_ _]
              tunnel: w1524 -> [_ _]
              tunnel: w1523 -> [w1557 w1643]
              tunnel: [w1549 w1641] -> w1522
              tunnel: [w1546 w1635] -> w1521
              tunnel: [FALSE FALSE] -> w1501
              tunnel: [w1551 w1632] -> w1520
              tunnel: w1517 -> [w1555 _]
              tunnel: w1519 -> [w1558 _]
              tunnel: w1518 -> [w1556 w1638]
              tunnel: [w1548 w1631] -> w1515
              tunnel: [w1547 w1631] -> w1516
              tunnel: w1507 -> [w1545 _]
              tunnel: [w1536 w1642] -> w1514
              tunnel: w1513 -> [w1534 w1626]
              tunnel: w1512 -> [w1539 w1639]
              tunnel: w1511 -> [w1535 w1637]
              tunnel: w1498 -> [_ _]
              tunnel: w1499 -> [_ w1634]
              tunnel: [FALSE w1633] -> w1509
              tunnel: w1506 -> [w1543 _]
              tunnel: w1505 -> [w1542 _]
              tunnel: [w1539 w1630] -> w1504
              frame "Recovery Search" {
                # "Wait for 2 Images to be Processed\nBefore Going to Next Step"
                # "Choose Next Reovery State"
                # "Recovery Search \nAttempt Count"
                # "Move Servo"
                # "Goal Position"
                # "Recovery Search\nmove Count"
                # "Attempt Recovery Search if Other Servo has Valid Angle"
                n571 = local read "Last Track Angle - L"() -> (w1538:sgl)
                n572 = Greater Or Equal?(x=w1534, y=w1535) -> (x >= y?=w1537:bool)
                n573 = case shown="True" w1537 {
                  tunnel: w1558 -> [_ w1578]
                  tunnel: [w1563 w1577] -> w1547
                  tunnel: w1557 -> [w1566 w1576]
                  tunnel: w1556 -> [_ w1575]
                  tunnel: [w1564 w1574] -> w1548
                  tunnel: [w1566 w1573] -> w1549
                  tunnel: [FALSE w1572] -> w1546
                  tunnel: w1543 -> [w1564 w1571]
                  tunnel: w1542 -> [w1563 w1570]
                  tunnel: w1545 -> [_ w1569]
                  tunnel: w1538 -> [_ w1568]
                  tunnel: [w1561 0 ("Frames Processed\nCount - in")] -> w1536
                  tunnel: w1534 -> [w1562 _]
                  frame False {
                    # "Increment Frames Processed"
                    # "WAIT"
                    n574 = Increment(x=w1562) -> (x+1=w1561:i32)
                  }
                  frame True {
                    n575 = case shown="True" w1569 {
                      tunnel: w1568 -> [_ w1591]
                      tunnel: w1571 -> [w1579 w1587]
                      tunnel: w1578 -> [_ w1592]
                      tunnel: [w1582 w1590] -> w1573
                      tunnel: [w1580 w1589] -> w1577
                      tunnel: w1570 -> [w1580 w1588]
                      tunnel: w1576 -> [w1582 w1586]
                      tunnel: w1575 -> [_ w1585]
                      tunnel: [FALSE TRUE] -> w1572
                      tunnel: [w1579 w1583] -> w1574
                      frame False {
                        # "Don't Move bc Other Servo Doesn't Have Image Lock"
                      }
                      frame True {
                        # "Move Servo = T"
                        n576 = Greater Than 0?(x=w1587) -> (x > 0?=w1593:bool)
                        n577 = case shown="False" w1593 {
                          tunnel: w1592 -> [w1600 _]
                          tunnel: w1591 -> [w1594 _]
                          tunnel: [w1599 w1610] -> w1590
                          tunnel: [w1597 w1616] -> w1589
                          tunnel: w1588 -> [w1598 w1616]
                          tunnel: w1587 -> [w1596 w1613]
                          tunnel: [w1595 w1615] -> w1583
                          tunnel: w1586 -> [_ w1611]
                          tunnel: w1585 -> [_ w1608]
                          frame False {
                            # "Increment move count to transition\nto Pan mode"
                            # "Increment Recovery Search Attempt Count"
                            # "1024/300"
                            # "Move Parallel to Other Servo"
                            n578 = Increment(x=w1598) -> (x+1=w1597:i32)
                            n579 = Add(x=w1594, y=w1600) -> (x+y=w1606:sgl)
                            n580 = Add(x=w1606, y=sgl 60.0) -> (x+y=w1605:sgl)
                            n581 = Multiply(x=3.413333333333333, y=w1605) -> (x*y=w1603:dbl)
                            n582 = Add(x=0.5, y=w1603) -> (x+y=w1601:dbl)
                            n583 = To Unsigned Word Integer(number=w1601) -> (unsigned 16bit integer=w1599:u16)
                            n584 = Increment(x=w1596) -> (x+1=w1595:i32)
                          }
                          frame True {
                            # "Apply Direction"
                            # "Step SIze"
                            # "Current Position"
                            # "Attempt to Pan in Steps Towards other Servo"
                            # "Could be same or function of \nregular search step size"
                            # "Max # of Pan\nMoves"
                            # "Pan Towards Other Servo"
                            n585 = Greater Or Equal?(x=w1613, y=u16 20) -> (x >= y?=w1614:bool)
                            n586 = case shown="False" w1614 {
                              tunnel: w1613 -> [w1624 _]
                              tunnel: [w1623 u16 0] -> w1615
                              frame False {
                                # "Increment Pan Count"
                                n587 = Increment(x=w1624) -> (x+1=w1623:i32)
                              }
                              frame True {
                                # "Reset move count"
                              }
                            }
                            n588 = local read "Recovery Search\nDirection - R"() -> (w1609:bool)
                            n589 = case shown="False" w1609 {
                              tunnel: w1611 -> [w1618 w1622]
                              tunnel: w1608 -> [w1619 w1621]
                              tunnel: [w1617 w1620] -> w1610
                              frame False {
                                # "CCW"
                                n590 = Add(x=w1618, y=w1619) -> (x+y=w1617:u16)
                              }
                              frame True {
                                # "CW"
                                n591 = Subtract(x=w1622, y=w1621) -> (x-y=w1620:u16)
                              }
                            }
                          }
                        }
                      }
                    }
                  }
                }
                n592 = local read "Max Recovery Count\n(Recovery Search)"() -> (w1540:u16)
                n593 = local read "Max Recovery\nSearch Attempts"() -> (w1541:u16)
                n594 = Less Or Equal?(x=w1547, y=w1541) -> (x <= y?=w1553:bool)
                n595 = Less Or Equal?(x=w1555, y=w1540) -> (x <= y?=w1554:bool)
                n596 = And(x=w1553, y=w1554) -> (x .and. y?=w1552:bool)
                n597 = case shown="True" w1552 {
                  tunnel: [enum16{"Generic Sweep", "Recovery Search"}."Generic Sweep" enum16{"Generic Sweep", "Recovery Search"}."Recovery Search"] -> w1551
                  frame False {
                  }
                  frame True {
                  }
                }
              }
              frame "Generic Sweep" {
                w1631 = u16 0
                # "Angle Valid?"
                # "Choose Next Recovery State"
                # "Wait for 2 Images to be Processed\nBefore Going to Next Step"
                # "New Goal Position"
                # "Move Servo"
                # "Frames Processed Count"
                n598 = Greater Or Equal?(x=w1626, y=w1637) -> (x >= y?=w1644:bool)
                n599 = case shown="True" w1644 {
                  tunnel: w1643 -> [w1660 w1672]
                  tunnel: w1638 -> [_ w1670]
                  tunnel: w1639 -> [w1659 w1669]
                  tunnel: [w1660 w1666] -> w1641
                  tunnel: [w1658 0] -> w1642
                  tunnel: [FALSE TRUE] -> w1636
                  tunnel: w1626 -> [w1661 _]
                  tunnel: [w1659 w1663] -> w1630
                  frame False {
                    # "Increment Frames Processed"
                    n600 = Increment(x=w1661) -> (x+1=w1658:i32)
                  }
                  frame True {
                    # "Reset Frames\nProcessed Count"
                    # "SWEEP SEARCH - Startup"
                    # "Multiple New Step\nby Step SIze"
                    # "F = CCW\nT = CW"
                    # "Last Direction"
                    # "Min Step"
                    # "add 10 in case\nactual position\nis lower than GP"
                    # "Set New Step #"
                    # "Choose Direction"
                    # "Nearest step"
                    # "Adjust Actual Posiiton\n to pre-determiend steps"
                    # "Move Servo 1 \"Step\" to\nSearch"
                    n601 = Add(x=5, y=w1672) -> (x+y=w1678:i32)
                    n602 = Quotient & Remainder(x=w1678, y=w1670) -> (floor(x/y)=w1676:i32)  [unwired: 1 out]
                    n603 = To Byte Integer(number=w1676) -> (8bit integer=w1667:i8)
                    n604 = Less?(x=w1667, y=1) -> (x < y?=w1673:bool)
                    n605 = case shown="False" w1673 {
                      tunnel: w1667 -> [w1689 w1697]
                      tunnel: [w1691 FALSE] -> w1663
                      tunnel: [w1690 w1697] -> w1675
                      tunnel: w1669 -> [w1688 _]
                      tunnel: w1670 -> [w1686 _]
                      frame False {
                        # "Max Step"
                        # "# of steps\nminus 1"
                        n606 = Divide(x=1024, y=w1686) -> (x/y=w1683:dbl)
                        n607 = To Unsigned Byte Integer(number=w1683) -> (unsigned 8bit integer=w1684:u8)
                        n608 = Greater Or Equal?(x=w1689, y=w1684) -> (x >= y?=w1685:bool)
                        n609 = case shown="True" w1685 {
                          tunnel: [w1692 TRUE] -> w1691
                          tunnel: [w1693 w1694] -> w1690
                          tunnel: w1689 -> [w1693 w1694]
                          tunnel: w1688 -> [w1692 _]
                          frame False {
                            # "No Need to\nChange Direction"
                          }
                          frame True {
                            # "T"
                            # "Move CW"
                          }
                        }
                      }
                      frame True {
                        # "F"
                        # "Move CCW"
                      }
                    }
                    n610 = case shown="True" w1663 {
                      tunnel: w1675 -> [w1680 w1681]
                      tunnel: [w1679 w1682] -> w1671
                      frame False {
                        # "CCW\n+1"
                        n611 = Increment(x=w1680) -> (x+1=w1679:i8)
                      }
                      frame True {
                        # "CW\n-1"
                        n612 = Decrement(x=w1681) -> (x-1=w1682:i8)
                      }
                    }
                    n613 = Multiply(x=w1671, y=w1670) -> (x*y=w1668:u16)
                    n614 = To Unsigned Word Integer(number=w1668) -> (unsigned 16bit integer=w1666:u16)
                  }
                }
                n615 = local read "Track Angle Valid - Left"() -> (w1629:bool)
                n616 = local read "Image Lock - Left"() -> (w1628:bool)
                n617 = Or(x=w1628, y=w1629) -> (x .or. y?=w1627:bool)
                n618 = case shown="False" w1634 {
                  tunnel: [w1647 w1657] -> w1635
                  tunnel: w1636 -> [w1648 _]
                  tunnel: [w1649 enum16{"Generic Sweep", "Recovery Search"}."Generic Sweep"] -> w1632
                  tunnel: [w1646 w1657] -> w1633
                  tunnel: w1627 -> [w1645 _]
                  frame False {
                    # "Is other servo tracking?"
                    n619 = case shown="True" w1645 {
                      tunnel: [enum16{"Generic Sweep", "Recovery Search"}."Generic Sweep" enum16{"Generic Sweep", "Recovery Search"}."Recovery Search"] -> w1649
                      tunnel: w1648 -> [w1652 _]
                      tunnel: [w1652 FALSE] -> w1647
                      tunnel: [FALSE TRUE] -> w1646
                      frame False {
                        # "Stay in Sweep"
                      }
                      frame True {
                        # "G o to Recovery Search  State"
                      }
                    }
                  }
                  frame True {
                    w1657 = FALSE
                    # "Override Move Servo\nCommand bc an Angle Was Found\nduring this Step"
                    # "Stay In Sweep\nLet Main State Machine transition\ninto Tracking"
                  }
                }
              }
            }
            n620 = Increment(x=w1517) -> (x+1=w1496:i32)
            n621 = case shown="True" w1509 {
              tunnel: w1496 -> [w1532 _]
              tunnel: [w1532 0] -> w1510
              frame False {
              }
              frame True {
              }
            }
            n622 = case shown="False" w1497 {
              tunnel: [T2."Recovery Mode" ("Next Main State") T2."Tracking" ("Next Main State")] -> w1508
              frame False {
              }
              frame True {
              }
            }
          }
        }
        "Current Move Delta - L 2" <- w1223
        n623 = Less?(x=w1250, y=w1249) -> (x < y?=w1248:bool)
        n624 = local write "New Data  Flag\nRight Servo"(FALSE) -> ()
        n625 = Select(t=w1249, s=w1248, f=w1250) -> (s? t:f=w1245:u16)
        n626 = Greater?(x=w1245, y=w1246) -> (0:w1247:bool)
        n627 = Select(t=w1246, s=w1247, f=w1245) -> (s? t:f=w1244:u16)
      }
    }
    "Next Main State - Right" <- w1108
    "Next Tracking State - Right" <- w1103
    "Next Recovery State - Right" <- w1104
    n628 = case shown="True" w1134 {
      tunnel: [w1709 w1747] -> w1181
      tunnel: [w1703 w1746] -> w1180
      tunnel: w1179 -> [w1704 w1745]
      tunnel: w1178 -> [_ w1744]
      tunnel: "Track Angle Valid - Left" -> [_ w1743]
      tunnel: w1176 -> [_ w1742]
      tunnel: w1175 -> [w1709 w1741]
      tunnel: "Mounting Offset - Left" -> [_ w1740]
      tunnel: w1173 -> [w1700 w1739]
      tunnel: w1172 -> [_ w1738]
      tunnel: w1171 -> [w1701 w1737]
      tunnel: w1170 -> [_ w1736]
      tunnel: w1169 -> [_ w1735]
      tunnel: w1168 -> [_ w1734]
      tunnel: "Middle Beacon\nCoordinates" -> [_ w1733]
      tunnel: w1166 -> [w1699 w1732]
      tunnel: w1165 -> [w1698 w1731]
      tunnel: w1164 -> [w1702 w1730]
      tunnel: w1163 -> [_ w1729]
      tunnel: w1162 -> [_ w1728]
      tunnel: w1161 -> [_ w1727]
      tunnel: [0 w1726] -> w1155
      tunnel: [w1704 w1725] -> w1154
      tunnel: [w1703 w1724] -> w1153
      tunnel: [w1702 w1723] -> w1152
      tunnel: [w1698 w1722] -> w1151
      tunnel: [w1701 w1721] -> w1150
      tunnel: [w1699 w1720] -> w1149
      tunnel: w1147 -> [_ w1719]
      tunnel: [w1700 w1718] -> w1146
      tunnel: w1144 -> [_ w1717]
      tunnel: w1140 -> [w1707 w1716]
      tunnel: w1139 -> [w1706 w1715]
      tunnel: [w1707 w1714] -> w1138
      tunnel: [w1706 w1713] -> w1137
      tunnel: w1136 -> [w1705 w1712]
      tunnel: [w1705 w1711] -> w1135
      frame False {
        w1703 = FALSE
        # "Recovery Mode COunt"
        # "Frames Processed - L"
        # "Recovery Search move Count - L"
        # "Recovery Search Attempt Count- L"
        # "WAITING FOR NEW IMAGE, RETAIN ALL VALUES"
      }
      frame True {
        w1749 = u16 1023
        w1752 = u16 0
        # "New Tracking State"
        # "Tracking Timeout Count"
        # "Next Main State"
        # "Next Recovery State"
        # "Reset Respond"
        # "Search Direction"
        # "Recovery Count"
        # "Recovery Search move Count"
        # "Recovery Search Attempt Count"
        # "Frames Processed"
        # "Apply Floor/Ceiling to Goal Position"
        # "Current move Delta"
        # "Service Track Angle Flag"
        # "Move Servo"
        # "Goal Position"
        # "Go to Current State"
        n629 = case shown="\"Recovery Mode\"" w1745 {
          tunnel: w1741 -> [w1771 w1848 w2026]
          tunnel: w1742 -> [_ w1850 _]
          tunnel: w1727 -> [w1770 _ w2021]
          tunnel: w1739 -> [w1769 w1830 w2015]
          tunnel: [w1768 w1846 w2025] -> w1753
          tunnel: [w1766 w1847 w2024] -> w1746
          tunnel: w1743 -> [w1764 w1841 w2002]
          tunnel: [w1763 w1843 w2011] -> w1725
          tunnel: w1744 -> [w1762 w1842 w2001]
          tunnel: w1740 -> [_ w1851 w2022]
          tunnel: w1729 -> [_ w1849 _]
          tunnel: [w1756 w1845 w2006] -> w1726
          tunnel: w1728 -> [_ w1844 _]
          tunnel: w1737 -> [w1761 _ w2016]
          tunnel: [enum16{"Generic Sweep", "Recovery Search"}."Recovery Search" enum16{"Generic Sweep", "Recovery Search"}."Recovery Search" w2023] -> w1711
          tunnel: w1732 -> [_ _ w2020]
          tunnel: w1712 -> [_ _ w2003]
          tunnel: w1738 -> [_ w1827 w2032]
          tunnel: w1719 -> [_ w1832 w2027]
          tunnel: w1734 -> [_ w1834 w2029]
          tunnel: w1735 -> [_ w1835 w2030]
          tunnel: w1736 -> [_ w1836 w2031]
          tunnel: w1733 -> [_ w1833 w2028]
          tunnel: [FALSE w1829 w2004] -> w1724
          tunnel: w1717 -> [w1760 _ w2014]
          tunnel: [w1756 w1824 w2013] -> w1720
          tunnel: [w1756 w1824 w2019] -> w1723
          tunnel: [w1756 w1824 w2018] -> w1722
          tunnel: [w1759 w1825 w2017] -> w1721
          tunnel: w1731 -> [_ _ w2009]
          tunnel: w1730 -> [_ _ w2008]
          tunnel: [w1757 w1830 w2007] -> w1718
          tunnel: w1716 -> [_ w1840 _]
          tunnel: [w1756 w1831 w2006] -> w1714
          tunnel: w1715 -> [_ w1837 _]
          tunnel: [enum16{"Track", "Reactive Predict", ""}."Track" ("Initial Tracking State - Right") w1828 enum16{"Track", "Reactive Predict", ""}."Track" ("Initial Tracking State - Right")] -> w1713
          frame "Start Up Search", Default {
            w1756 = u16 0
            # "Search Direction"
            # "Wait for 'x' Images to be Processed\nBefore Going to Next Step"
            # "Next Main State"
            # "New Goal Position"
            # "Move Servo"
            # "Choose Next State"
            # "Frames Processed Count"
            n630 = Greater Or Equal?(x=w1761, y=w1760) -> (x >= y?=w1767:bool)
            n631 = case shown="True" w1767 {
              tunnel: w1771 -> [w1786 w1798]
              tunnel: w1770 -> [_ w1796]
              tunnel: w1769 -> [w1785 w1795]
              tunnel: [w1786 w1792] -> w1768
              tunnel: [w1784 0] -> w1759
              tunnel: [FALSE TRUE] -> w1765
              tunnel: w1761 -> [w1787 _]
              tunnel: [w1785 w1789] -> w1757
              frame False {
                # "Increase Frames\nProcessed Count"
                n632 = Increment(x=w1787) -> (x+1=w1784:i32)
              }
              frame True {
                # "Reset Frames\nProcessed Count"
                # "SWEEP SEARCH - Startup"
                # "Multiple New Step\nby Step SIze"
                # "F = CCW\nT = CW"
                # "Last Direction"
                # "Min Step"
                # "add 10 in case\nactual position\nis lower than GP"
                # "Set New Step #"
                # "Choose Direction"
                # "Nearest step"
                # "Adjust Actual Posiiton\n to pre-determiend steps"
                # "Move Servo 1 \"Step\" to\nSearch"
                n633 = Add(x=3, y=w1798) -> (x+y=w1804:i32)
                n634 = Quotient & Remainder(x=w1804, y=w1796) -> (floor(x/y)=w1802:i32)  [unwired: 1 out]
                n635 = To Byte Integer(number=w1802) -> (8bit integer=w1793:i8)
                n636 = Less?(x=w1793, y=1) -> (x < y?=w1799:bool)
                n637 = case shown="False" w1799 {
                  tunnel: w1793 -> [w1815 w1823]
                  tunnel: [w1817 FALSE] -> w1789
                  tunnel: [w1816 w1823] -> w1801
                  tunnel: w1795 -> [w1814 _]
                  tunnel: w1796 -> [w1812 _]
                  frame False {
                    # "Max Step"
                    # "# of steps\nminus 1"
                    n638 = Divide(x=1024, y=w1812) -> (x/y=w1809:dbl)
                    n639 = To Unsigned Byte Integer(number=w1809) -> (unsigned 8bit integer=w1810:u8)
                    n640 = Greater Or Equal?(x=w1815, y=w1810) -> (x >= y?=w1811:bool)
                    n641 = case shown="True" w1811 {
                      tunnel: [w1818 TRUE] -> w1817
                      tunnel: [w1819 w1820] -> w1816
                      tunnel: w1815 -> [w1819 w1820]
                      tunnel: w1814 -> [w1818 _]
                      frame False {
                        # "No Need to\nChange Direction"
                      }
                      frame True {
                        # "T"
                        # "Move CW"
                      }
                    }
                  }
                  frame True {
                    # "F"
                    # "Move CCW"
                  }
                }
                n642 = case shown="False" w1789 {
                  tunnel: w1801 -> [w1806 w1807]
                  tunnel: [w1805 w1808] -> w1797
                  frame False {
                    # "CCW\n+1"
                    n643 = Increment(x=w1806) -> (x+1=w1805:i8)
                  }
                  frame True {
                    # "CW\n-1"
                    n644 = Decrement(x=w1807) -> (x-1=w1808:i8)
                  }
                }
                n645 = Multiply(x=w1797, y=w1796) -> (x*y=w1794:u16)
                n646 = To Unsigned Word Integer(number=w1794) -> (unsigned 16bit integer=w1792:u16)
              }
            }
            n647 = case shown="False" w1764 {
              tunnel: [w1775 FALSE] -> w1766
              tunnel: w1765 -> [w1775 _]
              tunnel: [w1776 w1781] -> w1763
              tunnel: w1762 -> [_ w1779]
              frame False {
                # "Check other Servo\nStay in Startup  State"
                n648 = local read "Track Angle Valid  - Right"() -> (w1772:bool)
                n649 = local read "Image Lock - Right"() -> (w1773:bool)
                n650 = Or(x=w1772, y=w1773) -> (x .or. y?=w1774:bool)
                n651 = case shown="True" w1774 {
                  tunnel: [T2."Start Up Search" ("Next Main State") T2."Recovery Mode" ("Next Main State")] -> w1776
                  frame False {
                  }
                  frame True {
                  }
                }
              }
              frame True {
                # "Override Move Servo\nCommand bc an Angle Was Found\nduring this Step"
                # "Transition to Tracking State When\nImage Processing has Locked"
                n652 = case shown="False" w1779 {
                  tunnel: [T2."Start Up Search" ("Next Main State") T2."Tracking" ("Next Main State")] -> w1781
                  frame False {
                  }
                  frame True {
                  }
                }
              }
            }
          }
          frame "Tracking" {
            w1824 = 0
            # "Frames Processed Count"
            # "Image Lock - L"
            # "Track Angle Valid"
            # "Tracking Angle"
            # "Tracking Timeout Count"
            # "Max ove delta"
            # "Move delta threshold"
            # "mount offset"
            # "Current Position"
            # "Move Respond"
            # "Trackin Timeout count"
            # "Move Servo"
            # "delta"
            # "GP"
            # "Reset Move Respond"
            # "New Tracking State"
            # "Delta Move Sum"
            # "Choose Next State"
            n653 = case shown="\"Track\", Default" w1837 {
              tunnel: w1851 -> [w1869 _]
              tunnel: w1850 -> [w1868 _]
              tunnel: w1849 -> [w1867 _]
              tunnel: w1848 -> [w1866 w1924]
              tunnel: [w1865 w1922] -> w1847
              tunnel: [w1864 w1930] -> w1846
              tunnel: [w1863 0] -> w1845
              tunnel: w1844 -> [w1862 _]
              tunnel: w1842 -> [w1861 w1914]
              tunnel: w1841 -> [w1860 w1917]
              tunnel: w1840 -> [w1859 w1919]
              tunnel: w1836 -> [_ w1929]
              tunnel: w1835 -> [_ w1928]
              tunnel: w1834 -> [_ w1927]
              tunnel: w1833 -> [_ w1926]
              tunnel: w1827 -> [_ w1925]
              tunnel: w1832 -> [_ w1923]
              tunnel: [TRUE w1920] -> w1829
              tunnel: [w1856 w1918] -> w1831
              tunnel: [w1854 w1916] -> w1828
              tunnel: [0 0] -> w1825
              frame "Track", Default {
                # "Reset"
                # "Tracking Timeout"
                # "Move Delta"
                # "Goal Position"
                # "Tracking Move"
                # "Move Servo"
                # "Only Consider Tracking Angle\n\nIF\n\nImage Locked        == T\nTrack Angle Flag   == T"
                n654 = And(x=w1861, y=w1860) -> (x .and. y?=w1853:bool)
                n655 = case shown="True" w1853 {
                  tunnel: w1869 -> [_ w1875]
                  tunnel: w1868 -> [_ w1893]
                  tunnel: w1867 -> [_ w1890]
                  tunnel: w1866 -> [w1872 w1880]
                  tunnel: [w1872 w1889] -> w1864
                  tunnel: [w1874 w1888] -> w1865
                  tunnel: [w1874 w1887] -> _
                  tunnel: [u16 0 w1886] -> w1863
                  tunnel: w1862 -> [_ w1882]
                  tunnel: w1859 -> [w1871 _]
                  tunnel: [w1870 0] -> w1856
                  frame False {
                    w1874 = FALSE
                    # "Increment timeout"
                    n656 = Increment(x=w1871) -> (x+1=w1870:i32)
                  }
                  frame True {
                    # "Convert Track Angle to UINT16"
                    # "1024/300"
                    # "Move to Tracking Angle \n\nif delta is greater than move servo threshold\nAND less than max move threshold"
                    n657 = Add(x=w1893, y=w1875) -> (x+y=w1896:sgl)
                    n658 = Add(x=w1896, y=sgl 60.0) -> (x+y=w1895:sgl)
                    n659 = Multiply(x=3.413333333333333, y=w1895) -> (x*y=w1876:dbl)
                    n660 = To Word Integer(number=w1880) -> (16bit integer=w1878:i16)
                    n661 = To Unsigned Word Integer(number=w1876) -> (unsigned 16bit integer=w1892:u16)
                    n662 = To Word Integer(number=w1876) -> (16bit integer=w1891:i16)
                    n663 = Subtract(x=w1891, y=w1878) -> (x-y=w1881:i16)
                    n664 = Absolute Value(x=w1881) -> (abs(x)=w1877:i16)
                    n665 = Greater Or Equal?(x=w1877, y=w1890) -> (x >= y?=w1884:bool)
                    n666 = Less Or Equal?(x=w1877, y=w1882) -> (x <= y?=w1883:bool)
                    n667 = And(x=w1884, y=w1883) -> (x .and. y?=w1885:bool)
                    n668 = case shown="True" w1885 {
                      tunnel: w1892 -> [_ w1904]
                      tunnel: [w1899 w1904] -> w1889
                      tunnel: [w1900 w1910] -> w1888
                      tunnel: [w1900 w1910] -> w1887
                      tunnel: w1880 -> [w1899 _]
                      tunnel: w1877 -> [_ w1909]
                      tunnel: [u16 0 w1909] -> w1886
                      tunnel: w1875 -> [_ w1903]
                      frame False {
                        w1900 = FALSE
                        # "Don't Move"
                      }
                      frame True {
                        w1910 = TRUE
                        # "45 DEG MOUNT OFFSET"
                        # "1024/300"
                        # "Current Delta"
                        # "Use new Track Angle"
                        n669 = Divide(x=w1904, y=3.413333333333333) -> (x/y=w1906:dbl)
                        n670 = Negate(x=w1903) -> (-x=w1902:sgl)
                        n671 = Subtract(x=w1906, y=sgl 60.0) -> (x-y=w1908:dbl)
                        n672 = Add(x=w1908, y=w1902) -> (x+y=w1901:dbl)
                        n673 = local write "Last Track Angle - L"(w1901) -> ()
                      }
                    }
                  }
                }
                n674 = local read "Timeout to \nEnable Reactive Predict"() -> (w1857:u16)
                n675 = Less?(x=w1856, y=w1857) -> (x < y?=w1855:bool)
                n676 = case shown="True" w1855 {
                  tunnel: [enum16{"Track", "Reactive Predict", ""}."Reactive Predict" ("Initial Tracking State - Right") enum16{"Track", "Reactive Predict", ""}."Track" ("Initial Tracking State - Right")] -> w1854
                  frame False {
                  }
                  frame True {
                  }
                }
              }
              frame "Reactive Predict" {
                # "Choose New\nTracking State"
                n677 = Or(x=w1914, y=w1917) -> (x .or. y?=w1913:bool)
                n678 = case shown="False" w1913 {
                  tunnel: [w1943 w1995] -> w1930
                  tunnel: w1929 -> [w1942 _]
                  tunnel: w1928 -> [w1941 _]
                  tunnel: w1927 -> [w1940 _]
                  tunnel: w1926 -> [w1939 _]
                  tunnel: w1925 -> [w1938 _]
                  tunnel: w1923 -> [w1937 _]
                  tunnel: [w1936 w1994] -> w1922
                  tunnel: [w1935 w1994] -> w1920
                  tunnel: w1919 -> [w1934 _]
                  tunnel: [w1933 0] -> w1918
                  tunnel: [enum16{"Track", "Reactive Predict", ""}."Reactive Predict" ("Initial Tracking State - Right") enum16{"Track", "Reactive Predict", ""}."Track" ("Initial Tracking State - Right")] -> w1916
                  tunnel: w1924 -> [w1931 w1995]
                  frame False {
                    # "Stay in Reactive State"
                    # "Increment Track Timeout"
                    # "Move Respond Flag"
                    n679 = Increment(x=w1934) -> (x+1=w1933:i32)
                    n680 = case shown="True" w1938 {
                      tunnel: w1942 -> [_ w1958]
                      tunnel: w1941 -> [_ w1957]
                      tunnel: w1940 -> [_ w1956]
                      tunnel: w1939 -> [_ w1955]
                      tunnel: w1937 -> [_ w1952]
                      tunnel: [w1944 w1948] -> w1943
                      tunnel: [w1945 w1947] -> w1936
                      tunnel: [w1945 w1947] -> w1935
                      tunnel: w1931 -> [w1944 w1946]
                      frame False {
                        w1945 = FALSE
                        # "Reset Move Respond = F"
                        # "Move Servo = F"
                      }
                      frame True {
                        w1947 = TRUE
                        # "Position Lock"
                        # "Current Servo\nPosition"
                        # "Reset Move\nRespond = T"
                        # "Move Servo = T"
                        # "Apply Direction \nto Offset (delta sum)"
                        # "Check Last Known Position of Robot"
                        n681 = case shown="True" w1958 {
                          tunnel: w1957 -> [_ w1986]
                          tunnel: w1956 -> [_ w1961]
                          tunnel: w1955 -> [_ w1962]
                          tunnel: [sgl 1.0 ("y") w1960] -> w1954
                          frame False {
                            # "No Position Data Available"
                            # "Default is to move\nSame Direction as other\nServo"
                          }
                          frame True {
                            w1967 = sgl 1.0 ("y")
                            # "Use previous position/orientation to Guess Which Direction to Move Servo"
                            # "Choose Search Direction"
                            # "\"Perpendicular \nThreshold\""
                            # "If Orientation is\n ~Perpendicular -> Start Search\n in Opposite Direction of Other"
                            # "****add 90 until orientation angle is fixed"
                            # "Last Orientation"
                            # "Convert to Rad"
                            # "Avoid Divide by 0"
                            # "-1/m"
                            # "Calculate Normal Line to \nLast Robot Position\nfrom Center Beacon"
                            # "last Position \nCoordinates"
                            n682 = Unbundle(w1986) -> ("X"=w1966:sgl, "Y"=w1965:sgl)
                            n683 = Unbundle(w1962) -> ("X"=w1964:sgl, "Y"=w1963:sgl)
                            n684 = Subtract(x=w1965, y=w1963) -> (x-y=w1982:sgl)
                            n685 = Subtract(x=w1966, y=w1964) -> (x-y=w1980:sgl)
                            n686 = Equal To 0?(x=w1980) -> (x = 0?=w1981:bool)
                            n687 = case shown="False" w1981 {
                              tunnel: w1982 -> [w1989 _]
                              tunnel: w1980 -> [w1988 _]
                              tunnel: [w1987 1000000000000000.0] -> w1979
                              frame False {
                                n688 = Divide(x=w1989, y=w1988) -> (x/y=w1987:sgl)
                              }
                              frame True {
                              }
                            }
                            n689 = Equal To 0?(x=w1979) -> (x = 0?=w1984:bool)
                            n690 = case shown="False" w1984 {
                              tunnel: [w1991 1e-08] -> w1983
                              tunnel: w1979 -> [w1991 _]
                              frame False {
                              }
                              frame True {
                                # "Can't have infinit slope"
                              }
                            }
                            n691 = Divide(x=-1.0, y=w1983) -> (x/y=w1978:dbl)
                            n692 = Inverse Tangent(1:w1978) -> (0:w1976:dbl)
                            n693 = expression code="(x/pi)*180.0" "radians to degrees"(w1976) -> (w1977:dbl)
                            n694 = To Single Precision Float(number=w1977) -> (single precision float=w1974:sgl)
                            n695 = Add(x=w1961, y=sgl 90.0) -> (x+y=w1973:sgl)
                            n696 = Subtract(x=w1974, y=w1973) -> (x-y=w1972:sgl)
                            n697 = Absolute Value(x=w1972) -> (abs(x)=w1971:sgl)
                            n698 = Less Or Equal?(x=w1971, y=sgl 10.0) -> (x <= y?=w1969:bool)
                            n699 = Negate(x=w1967) -> (-x=w1968:sgl)
                            n700 = Select(t=w1968, s=w1969, f=w1967) -> (s? t:f=w1960:sgl)
                          }
                        }
                        n701 = To Word Integer(number=w1954) -> (16bit integer=w1953:i16)
                        n702 = Multiply(x=w1953, y=w1952) -> (x*y=w1951:i32)
                        n703 = To Word Integer(number=w1946) -> (16bit integer=w1950:i16)
                        n704 = Add(x=w1951, y=w1950) -> (x+y=w1949:i32)
                        n705 = To Unsigned Word Integer(number=w1949) -> (unsigned 16bit integer=w1948:u16)
                      }
                    }
                  }
                  frame True {
                    w1994 = TRUE
                    # "Go Directly to Track State"
                  }
                }
              }
            }
            n706 = local read "Tracking Timeout\nThreshold"() -> (w1838:i32)
            n707 = Less?(x=w1831, y=w1838) -> (x < y?=w1839:bool)
            n708 = case shown="False" w1839 {
              tunnel: [T2."Recovery Mode" ("Next Main State") T2."Tracking" ("Next Main State")] -> w1843
              frame False {
              }
              frame True {
              }
            }
          }
          frame "Recovery Mode" {
            w2006 = u16 0
            # "***Compltetly resets as of R17, used to just reset to \"Max Recovery Count - 1\""
            # "Increment Recoveyr Mode Count"
            # "Frames Processed"
            # "Choose Next Main State"
            # "Reset recovery count"
            # "Recovery move\nCount"
            # "Recovery Search\nAttempt count"
            # "Move Servo = T"
            # "delta move sum"
            # "Robot Position Valid"
            n709 = local read "Image Lock - Right"() -> (w2010:bool)
            n710 = Or(x=w2001, y=w2002) -> (x .or. y?=w2000:bool)
            n711 = case shown="\"Recovery Search\"" w2003 {
              tunnel: w2032 -> [_ _]
              tunnel: w2031 -> [_ _]
              tunnel: w2030 -> [_ _]
              tunnel: w2029 -> [_ _]
              tunnel: w2028 -> [_ _]
              tunnel: w2027 -> [_ _]
              tunnel: w2026 -> [w2060 w2146]
              tunnel: [w2052 w2144] -> w2025
              tunnel: [w2049 w2138] -> w2024
              tunnel: [FALSE FALSE] -> w2004
              tunnel: [w2054 w2135] -> w2023
              tunnel: w2020 -> [w2058 _]
              tunnel: w2022 -> [w2061 _]
              tunnel: w2021 -> [w2059 w2141]
              tunnel: [w2051 w2134] -> w2018
              tunnel: [w2050 w2134] -> w2019
              tunnel: w2010 -> [w2048 _]
              tunnel: [w2039 w2145] -> w2017
              tunnel: w2016 -> [w2037 w2129]
              tunnel: w2015 -> [w2042 w2142]
              tunnel: w2014 -> [w2038 w2140]
              tunnel: w2001 -> [_ _]
              tunnel: w2002 -> [_ w2137]
              tunnel: [FALSE w2136] -> w2012
              tunnel: w2009 -> [w2046 _]
              tunnel: w2008 -> [w2045 _]
              tunnel: [w2042 w2133] -> w2007
              frame "Recovery Search" {
                # "Wait for 2 Images to be Processed\nBefore Going to Next Step"
                # "Choose Next Reovery State"
                # "Recovery Search \nAttempt Count"
                # "Move Servo"
                # "Goal Position"
                # "Recovery Search\nmove Count"
                # "Attempt Recovery Search if Other Servo has Valid Angle"
                n712 = local read "Last Track Angle - R"() -> (w2041:sgl)
                n713 = Greater Or Equal?(x=w2037, y=w2038) -> (x >= y?=w2040:bool)
                n714 = case shown="True" w2040 {
                  tunnel: w2061 -> [_ w2081]
                  tunnel: [w2066 w2080] -> w2050
                  tunnel: w2060 -> [w2069 w2079]
                  tunnel: w2059 -> [_ w2078]
                  tunnel: [w2067 w2077] -> w2051
                  tunnel: [w2069 w2076] -> w2052
                  tunnel: [FALSE w2075] -> w2049
                  tunnel: w2046 -> [w2067 w2074]
                  tunnel: w2045 -> [w2066 w2073]
                  tunnel: w2048 -> [_ w2072]
                  tunnel: w2041 -> [_ w2071]
                  tunnel: [w2064 0 ("Frames Processed\nCount - in")] -> w2039
                  tunnel: w2037 -> [w2065 _]
                  frame False {
                    # "Increment Frames Processed"
                    # "WAIT"
                    n715 = Increment(x=w2065) -> (x+1=w2064:i32)
                  }
                  frame True {
                    n716 = case shown="True" w2072 {
                      tunnel: w2071 -> [_ w2094]
                      tunnel: w2074 -> [w2082 w2090]
                      tunnel: w2081 -> [_ w2095]
                      tunnel: [w2085 w2093] -> w2076
                      tunnel: [w2083 w2092] -> w2080
                      tunnel: w2073 -> [w2083 w2091]
                      tunnel: w2079 -> [w2085 w2089]
                      tunnel: w2078 -> [_ w2088]
                      tunnel: [FALSE TRUE] -> w2075
                      tunnel: [w2082 w2086] -> w2077
                      frame False {
                        # "Don't Move bc Other Servo Doesn't Have Image Lock"
                      }
                      frame True {
                        # "Move Servo = T"
                        n717 = Greater Than 0?(x=w2090) -> (x > 0?=w2096:bool)
                        n718 = case shown="False" w2096 {
                          tunnel: w2095 -> [w2103 _]
                          tunnel: w2094 -> [w2097 _]
                          tunnel: [w2102 w2113] -> w2093
                          tunnel: [w2100 w2119] -> w2092
                          tunnel: w2091 -> [w2101 w2119]
                          tunnel: w2090 -> [w2099 w2116]
                          tunnel: [w2098 w2118] -> w2086
                          tunnel: w2089 -> [_ w2114]
                          tunnel: w2088 -> [_ w2111]
                          frame False {
                            # "Increment move count to transition\nto Pan mode"
                            # "Increment Recovery Search Attempt Count"
                            # "1024/300"
                            # "Move Parallel to Other Servo"
                            n719 = Increment(x=w2101) -> (x+1=w2100:i32)
                            n720 = Add(x=w2097, y=w2103) -> (x+y=w2109:sgl)
                            n721 = Add(x=w2109, y=sgl 60.0) -> (x+y=w2108:sgl)
                            n722 = Multiply(x=3.413333333333333, y=w2108) -> (x*y=w2106:dbl)
                            n723 = Add(x=0.5, y=w2106) -> (x+y=w2104:dbl)
                            n724 = To Unsigned Word Integer(number=w2104) -> (unsigned 16bit integer=w2102:u16)
                            n725 = Increment(x=w2099) -> (x+1=w2098:i32)
                          }
                          frame True {
                            # "Apply Direction"
                            # "Step SIze"
                            # "Current Position"
                            # "Attempt to Pan in Steps Towards other Servo"
                            # "Could be same or function of \nregular search step size"
                            # "Max # of Pan\nMoves"
                            # "Pan Towards Other Servo"
                            n726 = Greater Or Equal?(x=w2116, y=u16 20) -> (x >= y?=w2117:bool)
                            n727 = case shown="False" w2117 {
                              tunnel: w2116 -> [w2127 _]
                              tunnel: [w2126 u16 0] -> w2118
                              frame False {
                                # "Increment Pan Count"
                                n728 = Increment(x=w2127) -> (x+1=w2126:i32)
                              }
                              frame True {
                                # "Reset move count"
                              }
                            }
                            n729 = local read "Recovery Search\nDirection - L"() -> (w2112:bool)
                            n730 = case shown="False" w2112 {
                              tunnel: w2114 -> [w2121 w2125]
                              tunnel: w2111 -> [w2122 w2124]
                              tunnel: [w2120 w2123] -> w2113
                              frame False {
                                # "CCW"
                                n731 = Add(x=w2121, y=w2122) -> (x+y=w2120:u16)
                              }
                              frame True {
                                # "CW"
                                n732 = Subtract(x=w2125, y=w2124) -> (x-y=w2123:u16)
                              }
                            }
                          }
                        }
                      }
                    }
                  }
                }
                n733 = local read "Max Recovery Count\n(Recovery Search)"() -> (w2043:u16)
                n734 = local read "Max Recovery\nSearch Attempts"() -> (w2044:u16)
                n735 = Less Or Equal?(x=w2050, y=w2044) -> (x <= y?=w2056:bool)
                n736 = Less Or Equal?(x=w2058, y=w2043) -> (x <= y?=w2057:bool)
                n737 = And(x=w2056, y=w2057) -> (x .and. y?=w2055:bool)
                n738 = case shown="True" w2055 {
                  tunnel: [enum16{"Generic Sweep", "Recovery Search"}."Generic Sweep" enum16{"Generic Sweep", "Recovery Search"}."Recovery Search"] -> w2054
                  frame False {
                  }
                  frame True {
                  }
                }
              }
              frame "Generic Sweep" {
                w2134 = u16 0
                # "Angle Valid?"
                # "Choose Next Recovery State"
                # "Wait for 2 Images to be Processed\nBefore Going to Next Step"
                # "New Goal Position"
                # "Move Servo"
                # "Frames Processed Count"
                n739 = Greater Or Equal?(x=w2129, y=w2140) -> (x >= y?=w2147:bool)
                n740 = case shown="True" w2147 {
                  tunnel: w2146 -> [w2163 w2175]
                  tunnel: w2141 -> [_ w2173]
                  tunnel: w2142 -> [w2162 w2172]
                  tunnel: [w2163 w2169] -> w2144
                  tunnel: [w2161 0] -> w2145
                  tunnel: [FALSE TRUE] -> w2139
                  tunnel: w2129 -> [w2164 _]
                  tunnel: [w2162 w2166] -> w2133
                  frame False {
                    # "Increment Frames Processed"
                    n741 = Increment(x=w2164) -> (x+1=w2161:i32)
                  }
                  frame True {
                    # "Reset Frames\nProcessed Count"
                    # "SWEEP SEARCH - Startup"
                    # "Multiple New Step\nby Step SIze"
                    # "F = CCW\nT = CW"
                    # "Last Direction"
                    # "Min Step"
                    # "add 10 in case\nactual position\nis lower than GP"
                    # "Set New Step #"
                    # "Choose Direction"
                    # "Nearest step"
                    # "Adjust Actual Posiiton\n to pre-determiend steps"
                    # "Move Servo 1 \"Step\" to\nSearch"
                    n742 = Add(x=5, y=w2175) -> (x+y=w2181:i32)
                    n743 = Quotient & Remainder(x=w2181, y=w2173) -> (floor(x/y)=w2179:i32)  [unwired: 1 out]
                    n744 = To Byte Integer(number=w2179) -> (8bit integer=w2170:i8)
                    n745 = Less?(x=w2170, y=1) -> (x < y?=w2176:bool)
                    n746 = case shown="False" w2176 {
                      tunnel: w2170 -> [w2192 w2200]
                      tunnel: [w2194 FALSE] -> w2166
                      tunnel: [w2193 w2200] -> w2178
                      tunnel: w2172 -> [w2191 _]
                      tunnel: w2173 -> [w2189 _]
                      frame False {
                        # "Max Step"
                        # "# of steps\nminus 1"
                        n747 = Divide(x=1024, y=w2189) -> (x/y=w2186:dbl)
                        n748 = To Unsigned Byte Integer(number=w2186) -> (unsigned 8bit integer=w2187:u8)
                        n749 = Greater Or Equal?(x=w2192, y=w2187) -> (x >= y?=w2188:bool)
                        n750 = case shown="True" w2188 {
                          tunnel: [w2195 TRUE] -> w2194
                          tunnel: [w2196 w2197] -> w2193
                          tunnel: w2192 -> [w2196 w2197]
                          tunnel: w2191 -> [w2195 _]
                          frame False {
                            # "No Need to\nChange Direction"
                          }
                          frame True {
                            # "T"
                            # "Move CW"
                          }
                        }
                      }
                      frame True {
                        # "F"
                        # "Move CCW"
                      }
                    }
                    n751 = case shown="True" w2166 {
                      tunnel: w2178 -> [w2183 w2184]
                      tunnel: [w2182 w2185] -> w2174
                      frame False {
                        # "CCW\n+1"
                        n752 = Increment(x=w2183) -> (x+1=w2182:i8)
                      }
                      frame True {
                        # "CW\n-1"
                        n753 = Decrement(x=w2184) -> (x-1=w2185:i8)
                      }
                    }
                    n754 = Multiply(x=w2174, y=w2173) -> (x*y=w2171:u16)
                    n755 = To Unsigned Word Integer(number=w2171) -> (unsigned 16bit integer=w2169:u16)
                  }
                }
                n756 = local read "Track Angle Valid  - Right"() -> (w2132:bool)
                n757 = local read "Image Lock - Right"() -> (w2131:bool)
                n758 = Or(x=w2131, y=w2132) -> (x .or. y?=w2130:bool)
                n759 = case shown="False" w2137 {
                  tunnel: [w2150 w2160] -> w2138
                  tunnel: w2139 -> [w2151 _]
                  tunnel: [w2152 enum16{"Generic Sweep", "Recovery Search"}."Generic Sweep"] -> w2135
                  tunnel: [w2149 w2160] -> w2136
                  tunnel: w2130 -> [w2148 _]
                  frame False {
                    # "Is other servo tracking?"
                    n760 = case shown="True" w2148 {
                      tunnel: [enum16{"Generic Sweep", "Recovery Search"}."Generic Sweep" enum16{"Generic Sweep", "Recovery Search"}."Recovery Search"] -> w2152
                      tunnel: w2151 -> [w2155 _]
                      tunnel: [w2155 FALSE] -> w2150
                      tunnel: [FALSE TRUE] -> w2149
                      frame False {
                        # "Stay in Sweep"
                      }
                      frame True {
                        # "G o to Recovery Search  State"
                      }
                    }
                  }
                  frame True {
                    w2160 = FALSE
                    # "Override Move Servo\nCommand bc an Angle Was Found\nduring this Step"
                    # "Stay In Sweep\nLet Main State Machine transition\ninto Tracking"
                  }
                }
              }
            }
            n761 = Increment(x=w2020) -> (x+1=w1999:i32)
            n762 = case shown="True" w2012 {
              tunnel: w1999 -> [w2035 _]
              tunnel: [w2035 0] -> w2013
              frame False {
              }
              frame True {
              }
            }
            n763 = case shown="False" w2000 {
              tunnel: [T2."Recovery Mode" ("Next Main State") T2."Tracking" ("Next Main State")] -> w2011
              frame False {
              }
              frame True {
              }
            }
          }
        }
        "Current Move Delta - L" <- w1726
        n764 = Less?(x=w1753, y=w1752) -> (x < y?=w1751:bool)
        n765 = local write "New Data  Flag\nLeft Servo"(FALSE) -> ()
        n766 = Select(t=w1752, s=w1751, f=w1753) -> (s? t:f=w1748:u16)
        n767 = Greater?(x=w1748, y=w1749) -> (0:w1750:bool)
        n768 = Select(t=w1749, s=w1750, f=w1748) -> (s? t:f=w1747:u16)
      }
    }
    "Next Main State - Left" <- w1154
    "Next Tracking State - Left" <- w1137
    "Next Recovery State - Left" <- w1135
    n769 = flat-sequence {
      tunnel: w1180 -> [w2207]
      tunnel: w1107 -> [w2206]
      tunnel: w1181 -> [w2209]
      tunnel: w1096 -> [w2208]
      tunnel: [w2207] -> w1194
      tunnel: [w2206] -> w1193
      tunnel: w1194 -> [w2215]
      tunnel: [w2214] -> w1189
      tunnel: [w2213] -> w1190
      tunnel: w1193 -> [w2212]
      frame #0 {
        # "Only Update GP if Moving Servo"
        n770 = case shown="True" w2207 {
          tunnel: w2209 -> [_ w2211]
          frame False {
          }
          frame True {
            # "Update Goal Position"
            n771 = local write "Servo Goal Position\n - Left"(w2211) -> ()
          }
        }
        n772 = case shown="True" w2206 {
          tunnel: w2208 -> [_ w2210]
          frame False {
          }
          frame True {
            # "New Direction"
            # "Update Goal Position"
            # "Update Direction"
            n773 = local write "Servo Goal Position\n - Right"(w2210) -> ()
          }
        }
      }
      frame #1 {
        # "Allow Comm Process to Take Down the Flag\nOnly Raise if not already in motion"
        n774 = local read "Servo Moving - R"() -> (w2220:bool)
        n775 = local read "Servo Moving - L"() -> (w2217:bool)
        n776 = local read "Move Servo - L"() -> (w2216:bool)
        n777 = local read "Move Servo - R"() -> (w2223:bool)
        n778 = Not(x=w2220) -> (.not. x?=w2222:bool)
        n779 = Not(x=w2217) -> (.not. x?=w2219:bool)
        n780 = And(x=w2212, y=w2222) -> (x .and. y?=w2221:bool)
        n781 = And(x=w2215, y=w2219) -> (x .and. y?=w2218:bool)
        n782 = case shown="True" w2221 {
          selector: w2221 -> [_ w2225]
          tunnel: [w2224 w2225] -> w2213
          tunnel: w2223 -> [w2224 _]
          frame False {
          }
          frame True {
          }
        }
        n783 = case shown="False" w2218 {
          selector: w2218 -> [_ w2227]
          tunnel: [w2226 w2227] -> w2214
          tunnel: w2216 -> [w2226 _]
          frame False {
          }
          frame True {
          }
        }
        n784 = local write "Move Servo - R"(w2213) -> ()
        n785 = local write "Move Servo - L"(w2214) -> ()
      }
    }
    n786 = local read "Current Main State - Right"() -> (w1159:T2)
    n787 = local read "Current Main State - Left"() -> (w1160:T2)
    n788 = Equal?(x=w1160, y=w1158) -> (x = y?=w1157:bool)
    n789 = Equal?(x=w1159, y=w1158) -> (x = y?=w1156:bool)
    n790 = And(x=w1157, y=w1189) -> (x .and. y?=w1185:bool)
    n791 = And(x=w1190, y=w1156) -> (x .and. y?=w1186:bool)
    n792 = And(x=w1157, y=w1156) -> (x .and. y?=w1184:bool)
    n793 = Exclusive Or(1:w1186, 2:w1185) -> (0:w1183:bool)
    n794 = case shown="True" w1183 {
      tunnel: [w2238 w2259] -> w1191
      tunnel: [w2239 w2258] -> w1187
      tunnel: w1106 -> [_ w2262]
      tunnel: w1147 -> [w2236 w2263]
      tunnel: w1110 -> [w2234 w2261]
      tunnel: [w2237 w2249] -> w1188
      tunnel: [w2235 w2248] -> w1192
      tunnel: w1155 -> [_ w2260]
      tunnel: w1184 -> [w2233 _]
      tunnel: w1185 -> [_ w2259]
      tunnel: w1186 -> [_ w2258]
      frame False {
        n795 = case shown="False" w2233 {
          tunnel: [w2243 w2245] -> w2239
          tunnel: [w2242 w2245] -> w2238
          tunnel: [w2241 w2244] -> w2237
          tunnel: w2236 -> [w2241 _]
          tunnel: [w2240 w2244] -> w2235
          tunnel: w2234 -> [w2240 _]
          frame False {
            # "No Movement\nRetain All Values"
            n796 = local read "Move Respond - L"() -> (w2243:bool)
            n797 = local read "Move Respond - R"() -> (w2242:bool)
          }
          frame True {
            w2244 = i16 0
            w2245 = FALSE
            # "Reset Delta Move sum\nfor both"
            # "F"
            # "Both Moved,\nMake Flags False"
          }
        }
      }
      frame True {
        w2255 = 200 ("y")
        w2246 = -200 ("y")
        # "Add/Clear Sum for \nServo That didn't move"
        # "Update Moving Servo's  Delta Position"
        # "if one Servo Moves, other should \nmove too eventually,\nUsed in Search Process"
        # "Only 1 Servo is Moving Due to Tracking --> Update delta move sum"
        n798 = case shown="True" w2258 {
          tunnel: w2263 -> [_ w2271]
          tunnel: w2262 -> [_ w2270]
          tunnel: [i16 0 w2269] -> w2256
          frame False {
          }
          frame True {
            n799 = Add(x=w2271, y=w2270) -> (x+y=w2269:i32)
          }
        }
        n800 = case shown="True" w2259 {
          tunnel: w2261 -> [_ w2267]
          tunnel: w2260 -> [_ w2266]
          tunnel: [i16 0 w2265] -> w2253
          frame False {
          }
          frame True {
            n801 = Add(x=w2267, y=w2266) -> (x+y=w2265:i32)
          }
        }
        n802 = Greater?(x=w2256, y=w2255) -> (0:w2257:bool)
        n803 = Greater?(x=w2253, y=w2255) -> (0:w2254:bool)
        n804 = Select(t=w2255, s=w2254, f=w2253) -> (s? t:f=w2250:i32)
        n805 = Select(t=w2255, s=w2257, f=w2256) -> (s? t:f=w2251:i32)
        n806 = Greater?(x=w2251, y=w2246) -> (0:w2247:bool)
        n807 = Greater?(x=w2250, y=w2246) -> (0:w2252:bool)
        n808 = Select(t=w2250, s=w2252, f=w2246) -> (s? t:f=w2248:i32)
        n809 = Select(t=w2251, s=w2247, f=w2246) -> (s? t:f=w2249:i32)
      }
    }
    n810 = case shown="True" w1102 {
      selector: w1102 -> [_ w2205]
      tunnel: [w2202 w2204] -> w1142
      tunnel: [w2201 i16 0] -> w1143
      tunnel: w1191 -> [w2202 _]
      tunnel: w1192 -> [w2201 _]
      frame False {
      }
      frame True {
        n811 = Not(x=w2205) -> (.not. x?=w2204:bool)
      }
    }
    "Move Respond - R" <- w1142
    "deltaMoveServo\n- R" <- w1143
    n812 = case shown="False" w1153 {
      selector: w1153 -> [_ w2232]
      tunnel: [w2229 w2231] -> w1145
      tunnel: [w2228 i16 0] -> w1148
      tunnel: w1187 -> [w2229 _]
      tunnel: w1188 -> [w2228 _]
      frame False {
      }
      frame True {
        n813 = Not(x=w2232) -> (.not. x?=w2231:bool)
      }
    }
    "Move Respond - L" <- w1145
    "deltaMoveServo\n- L" <- w1148
    "Current Main State - Left" <- w1179
    "Frames Processed\nCount - in -L" <- w1171
    "Recovery Mode Count - in Left" <- w1166
    "Recovery Search\nmove Count - in - L" <- w1165
    "Recovery Search\nAttempt Count - in - L" <- w1164
    "Current Main State - Right" <- w1133
    "Frames Processed\nCount - in Right" <- w1116
    "Recovery Search\nmove Count - Right" <- w1118
    "Recovery Search\nAttempt Count - Right" <- w1117
    "Recovery Mode Count in Right" <- w1109
    "Tracking Timeout\nCount - L" <- w1140
    "Tracking Timeout\nCount - R" <- w1125
    "Current Tracking State - Left" <- w1139
    "Current Tracking State - Right 2" <- w1131
    "Current Recovery State - Right" <- w1132
    "Current Recovery State -L" <- w1136
  }
